vi "Main_Marvin Remake.vi"() -> ()   [LabVIEW 2017]
uses:
  PCAN_Driver/ControlCAN.llb/DevType.ctl
  PCAN_Driver/ControlCAN.llb/CAN Channel.ctl
  PCAN_Driver/ControlCAN.llb/VCI_INIT_CONFIG.ctl
  PCAN_Driver/ControlCAN.llb/InitFlag.ctl
  PCAN_Driver/ControlCAN.llb/Fliter.ctl
  PCAN_Driver/ControlCAN.llb/Mode.ctl
  <vilib>/Utility/miscctls.llb/LVRowAndColumnTypeDef.ctl
  <vilib>/Utility/config.llb/Read Key (String).vi
  <vilib>/Utility/config.llb/Write Key (String).vi
  <vilib>/Utility/cursorutil.llb/Set Cursor (Icon Pict).vi
  PCAN_Driver/ControlCAN.lvlib
  <vilib>/Utility/config.llb/NI_LVConfig.lvlib
panel:
  out "ClosePanel":bool=TRUE
  out "UUT SN Report":string
  out "Automation":bool
  out "Test Failed":bool
  out "AuxiOFFResult":bool
  out "AuxiONResult":bool
  out "SensCalResult":bool
  out "VisualInspectionResult":bool
  out "BurnResult":bool
  out "BurnSpeed":bool
  out "BurnTemp":bool
  out "BurnDC":bool
  out "TempControlResult":bool
  out "MotorTempResult":bool
  out "StopTimeResult":bool
  out "SpeedResult":bool=TRUE
  out "VenableDirectionResult":bool
  out "VenableResult":bool
  out "ComTestResult":bool=TRUE
  out "UUT SoftwareVer":string
  out "Next SN":i32
  in  "SetSN":bool
  out "Current SN":i32
  out "Cal":dbl
  out "AO[1]Meas":dbl
  out "FullSpeed2 Speed":dbl
  out "FullSpeed2 Current":dbl
  out "FullSpeed1 Current":dbl
  out "FullSpeed1 Speed":dbl
  out "MaxBurnInTempVal":dbl
  in  "Stop Burn-in":bool
  out "VISA Tester":refnum<visa-resource-name>
  out "UUT":u8
  out "CAN Status":bool
  in  "Channel 2":T1 caption="Channel" items=["Channel 1", "Channel 2"]
  out "Config_CANAT":T7 {"DevType" items=["USB-CAN"=3, "USB-CAN2"=4]; "CanIndex" items=["通道1", "通道2"]; "VCI_INIT_CONFIG"."Fliter" items=["接收所有类型"=3, "只接收标准帧"=4, "只接收扩展帧"=7]; "VCI_INIT_CONFIG"."Mode" items=["正常工作", "自测模式（环回）", "仅侦听模式"]; "VCI_INIT_CONFIG"."InitFlag" items=["使用Flash参数", "使用界面设置参数"]}
  out "Array":u64[][](array[numeric]) format="%016x"
  out "Motor Phase Current RMS":dbl
  out "Ambient Temperature":dbl
  out "Speed error":bool
  out "Commutation err":bool
  out "Under voltage/Over voltage":bool
  out "Derated drive temp":bool
  out "Motor Over temperature":bool
  out "Motor Sensor temp Fauilre":bool
  out "Drive Over temperature":bool
  out "Drive Sensor temp Failure":bool
  out "Ambient Over temp":bool
  out "Ambient Sensor temp":bool
  out "DC Voltage":dbl
  out "DC Current":dbl
  out "Power transistor Heat sink Temp.":dbl
  out "Motor Stator Temp.":dbl
  out "Motor Speed RPM":dbl
  out "ECS State":u16
  out "UUT":string="EBAY"
  in  "Logger Path":path
  in  "Report":bool
  in  "Start":bool
  in  "ATR":string[][](table)=[["Test Communication", "-", "-", "-", "-", ""], ["Set S/N", "-", "-", "-", "-", ""], ["Set Board Number", "-", "-", "-", "-", ""], [" ", "", "", "", "", ""], ["Test Communication", "-", "-", "-", "-", ""], ["Get S/N", "-", "-", "-", "", ""], ["Get Board Number", "-", "-", "-", "", ""], ["Get FW", "-", "-", "-", "", ""], ["Enable Motor", "", "", "", "", ""], ["Small position command", "", "", "", "", ""], ["Measure delta", "", "", "", "", ""], ["Velocity command", "", "", "", "", ""]]
  in  "Settings":bool
  in  "Refresh Button":bool
  out "Status":bool
  in  "VISA Marvin":refnum<visa-resource-name>="COM6"
  in  "Serial Com":bool
  in  "Help Button":bool
  out "Pannel User Message":string
  in  "Stop Button":bool
  # "Marvin"
  # "REDLER TECHNOLOGIES LTD"
  # "ver 1.2o"
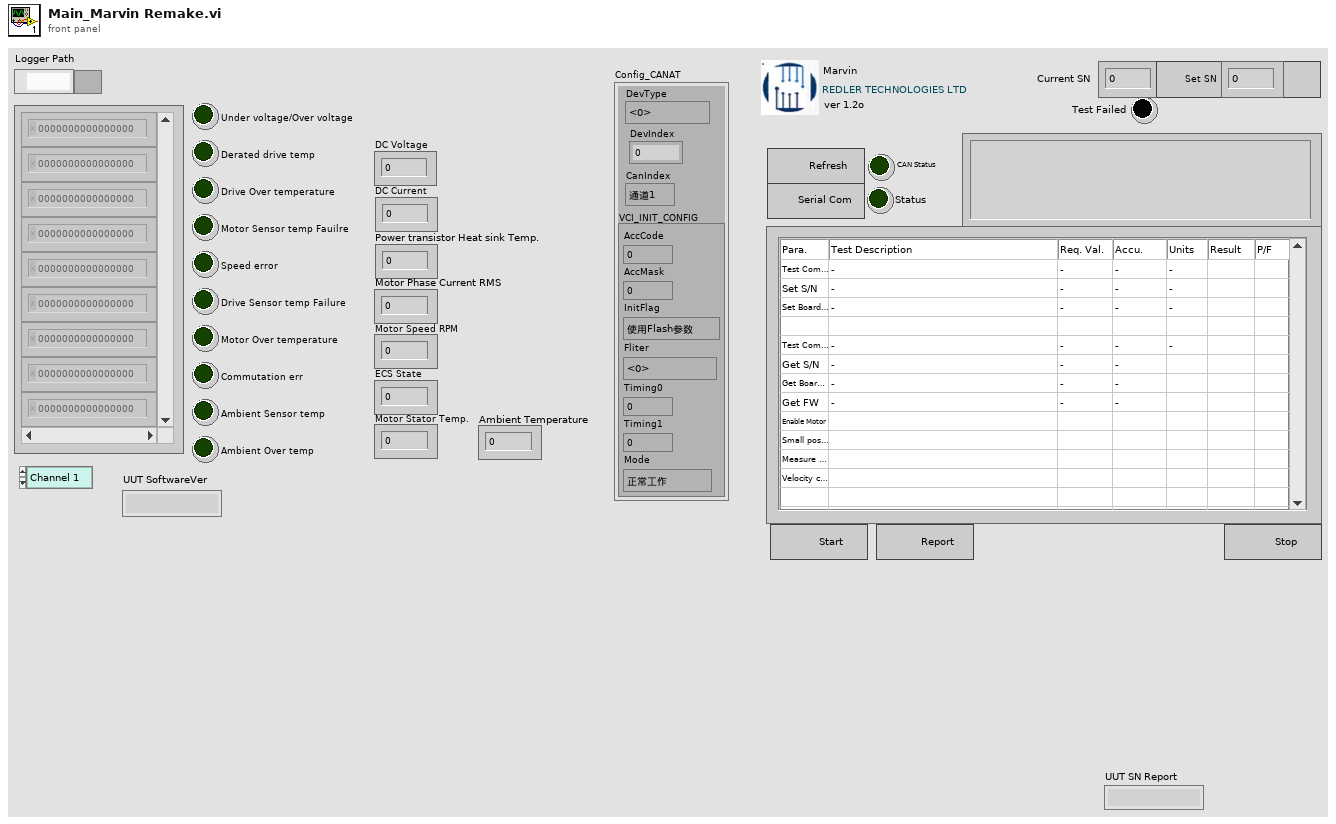
[diagram p1: front panel]
types:
  T1 = typedef "ControlCAN.lvlib/CAN Channel.ctl" = u32
  T2 = typedef "ControlCAN.lvlib/DevType.ctl" = u32
  T3 = typedef "ControlCAN.lvlib/VCI_INIT_CONFIG.ctl" = cluster{"AccCode":u32, "AccMask":u32, "InitFlag":T4, "Fliter":T5, "Timing0":u8, "Timing1":u8, "Mode":T6}
  T4 = typedef "ControlCAN.lvlib/InitFlag.ctl" = u32
  T5 = typedef "ControlCAN.lvlib/Fliter.ctl" = u8
  T6 = typedef "ControlCAN.lvlib/Mode.ctl" = u8
  T7 = cluster{"DevType":T2, "DevIndex":u32, "CanIndex":T1, "VCI_INIT_CONFIG":T3}
  T8 = cluster{"VISA":refnum<visa-resource-name>, "Array Test":enum16{"Auxiliary", "Temp Sens Cal", "Com Test", "Enable Test", "Speed Command", "Stop Time", "Temp Control", "Burn in", "Visual Inspec", "Empty"}[]}
  T9 = cluster{"ID":u32, "MSGTYPE":u8, "LEN":u8, "aDATA":u8[]}[]
  T10 = enum16{"Erase ATR Table", "Stop", "MainProgram", "Initialize"}
  T11 = enum16{"K15", "K16", "K17", "Venable", "Firmeware", "Fan", "Power", "120C", "110C", "100C", "90C", "80C", "70C", "60C", "50C", "40C", "30C", "25C", "20C", "10C", "0C"}
  T12 = enum16{"Stop", "Result", "FullSpeed2", "MD[1]=1", "FullSpeed1", "MD[1]=0"}
  T13 = enum8{"Term1", "Term2", "Current", "Fan", "TempCPU"}
  T14 = enum16{"Stop", "AO[1]=Meas.", "TA[5]", "AO[1]=0", "Start"}
  T15 = enum16{"Stop", "BurnIn", "Ambient Temp", "MotorSpeed", "DC Current Measure", "Start"}
  T16 = enum16{"Auxiliary", "Temp Sens Cal", "Com Test", "Enable Test", "Speed Command", "Stop Time", "Temp Control", "Burn in", "Visual Inspec", "Empty"}[]
  T17 = enum16{"K15", "K16", "K17", "Venable", "Firmeware", "Fan", "Power", "120C", "110C", "100C", "90C", "80C", "70C", "60C", "50C", "40C", "30C", "25C", "20C", "10C", "0C"}[]
  T18 = typedef "NI_LVConfig.lvlib/Config Data RefNum.ctl" = refnum<k1>
  T19 = enum32{"6000", "11500", "15100", "11500-2", "6000-2"}[]
  T20 = enum8{"Enabled", "Disabled", "Disabled and Grayed Out"}
  T21 = typedef "LVRowAndColumnTypeDef.ctl" = cluster{"Row":i32, "Column":i32}
  T22 = enum32{"Invalid", "Standard", "Closed", "Hidden", "Minimized", "Maximized"}
  T23 = cluster{"ID":u32, "MSGTYPE":u8, "LEN":u8, "aDATA":u8[]}
  T24 = enum16{"Auxiliary", "Temp Sens Cal", "Com Test", "Enable Test", "Speed Command", "Stop Time", "Temp Control", "Burn in", "Visual Inspec", "Empty"}
  T25 = enum16{"open", "replace", "create", "open or create", "replace or create", "replace or create with confirmation"}
  T26 = typedef "ControlCAN.lvlib/VCI_CAN_OBJ.ctl" = cluster{"ID":u32, "TimeStamp":u32, "TimeFlag":u8, "SendType":u8, "RemoteFlag":u8, "ExternFlag":u8, "DataLen":u8, "Data":u8[], "Reserved":u8[]}
  T27 = cluster{"Type":enum16{"接收", "发送"}, "Channel":T1, "Time":timestamp, "VCI_CAN_OBJ":T26}[]
  T28 = cluster{"Type":enum16{"接收", "发送"}, "Channel":T1, "Time":timestamp, "VCI_CAN_OBJ":T26}
  T29 = typedef "LVPoint32TypeDef.ctl" = cluster{"Horizontal":i32, "Vertical":i32}
  T30 = enum8{"Term1", "Term2", "Current", "Fan", "TempCPU"}[]
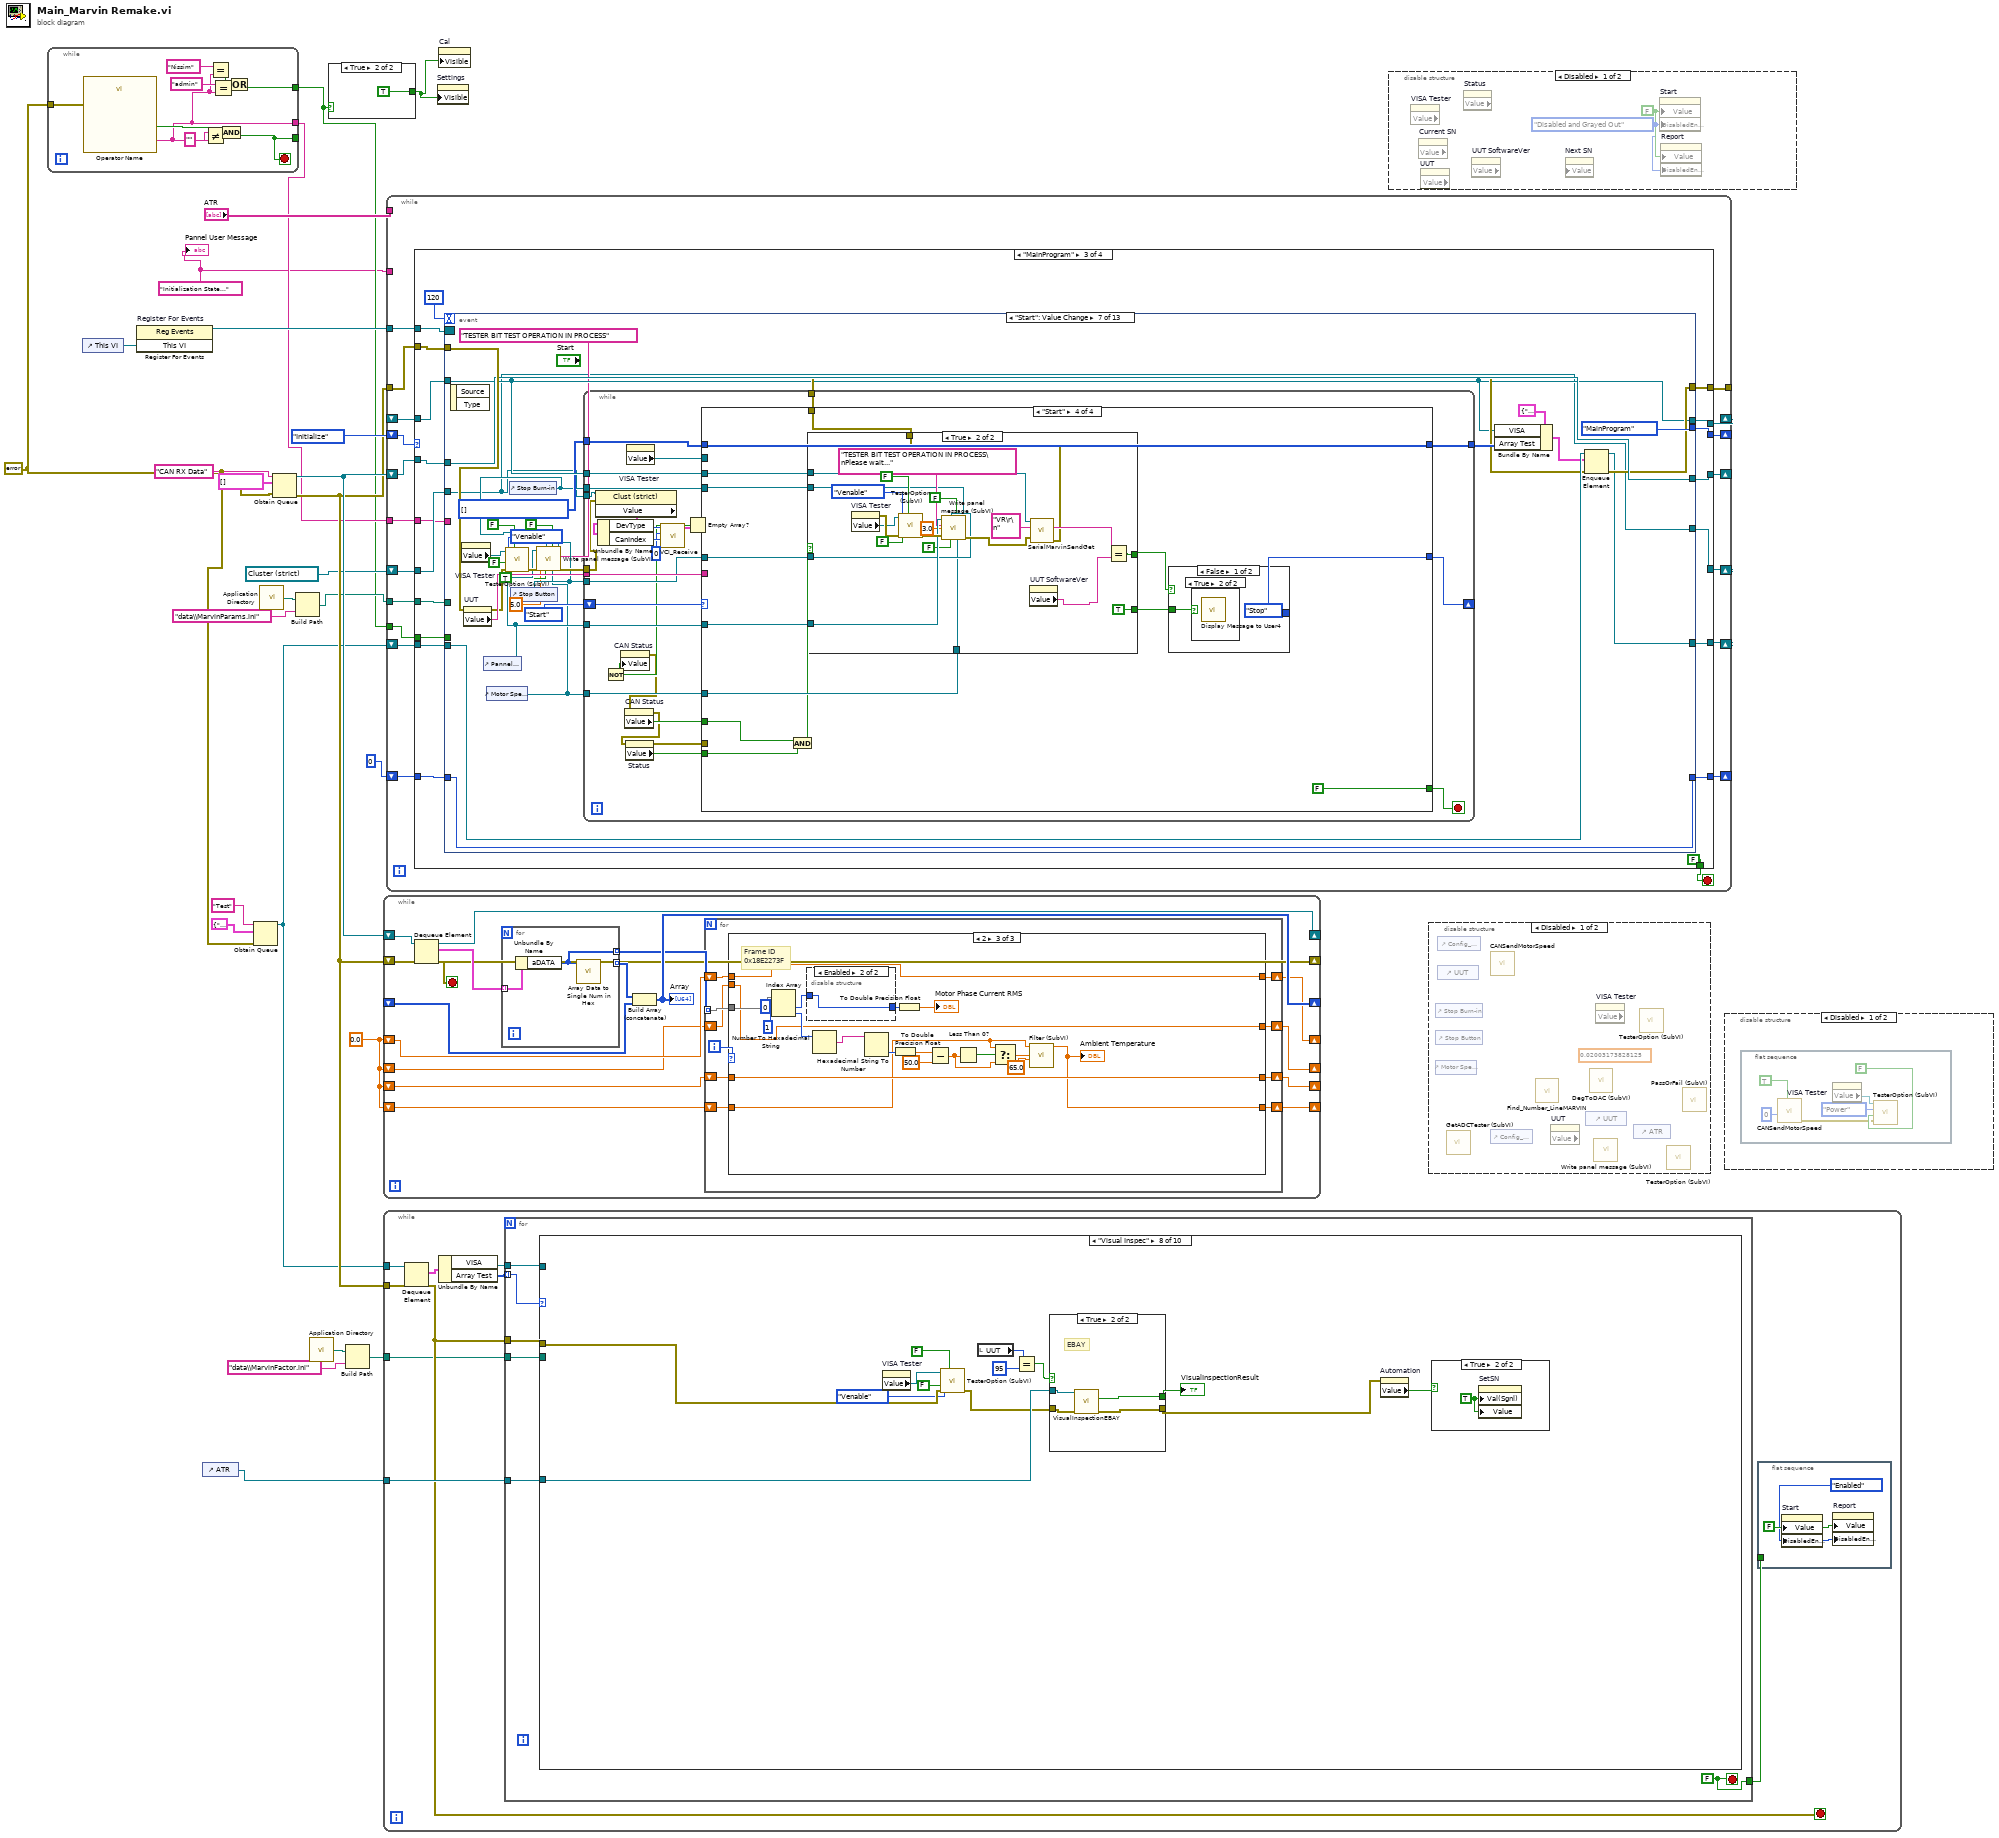
[diagram p0: block diagram]
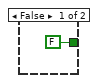
[diagram p2: hidden frame]
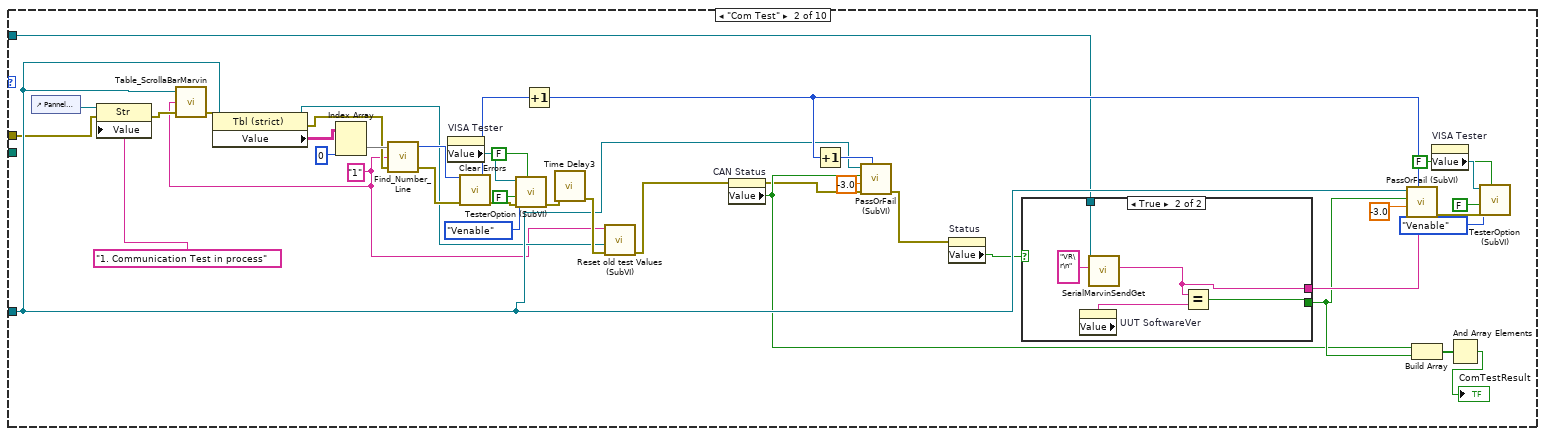
[diagram p7: hidden frame]
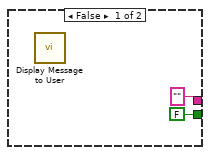
[diagram p8: hidden frame]
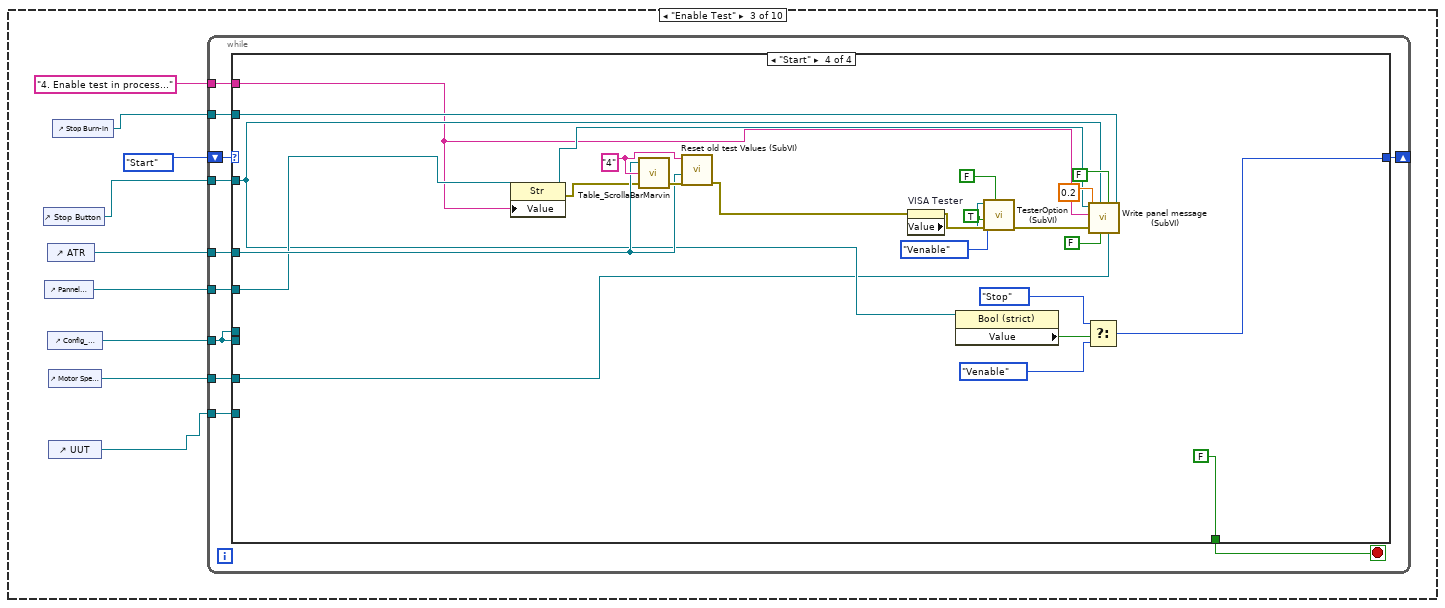
[diagram p9: hidden frame]
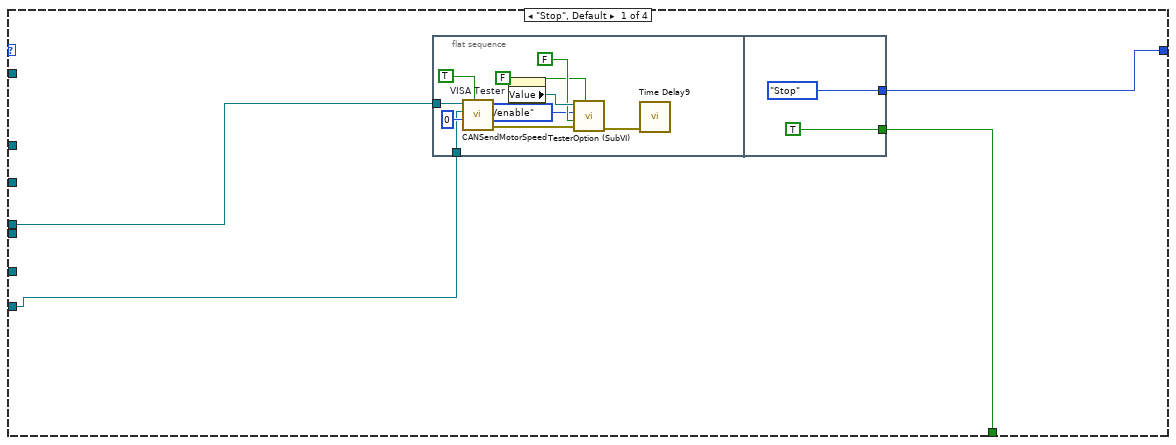
[diagram p10: hidden frame]
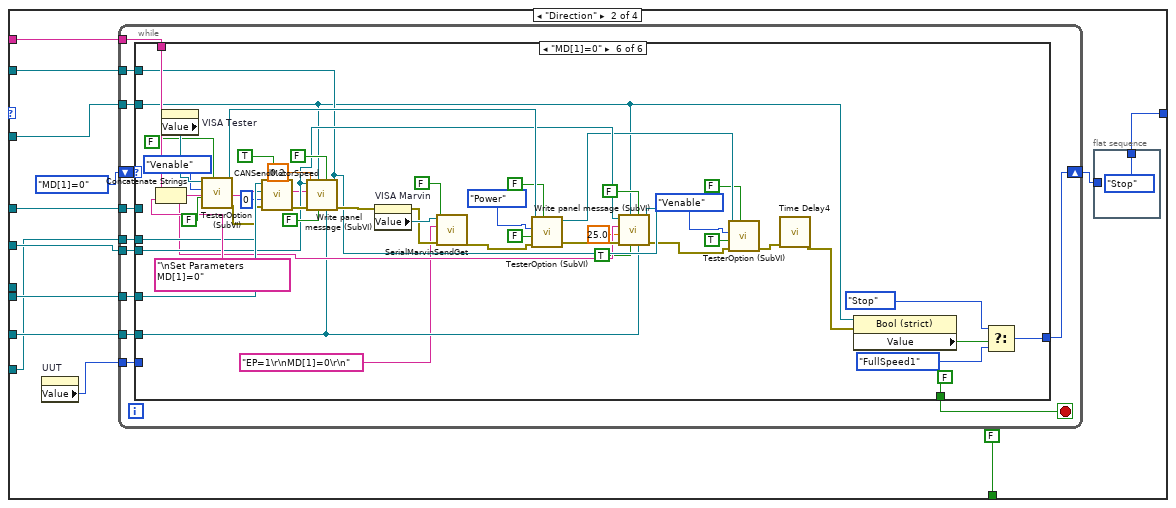
[diagram p11: hidden frame]
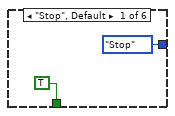
[diagram p12: hidden frame]
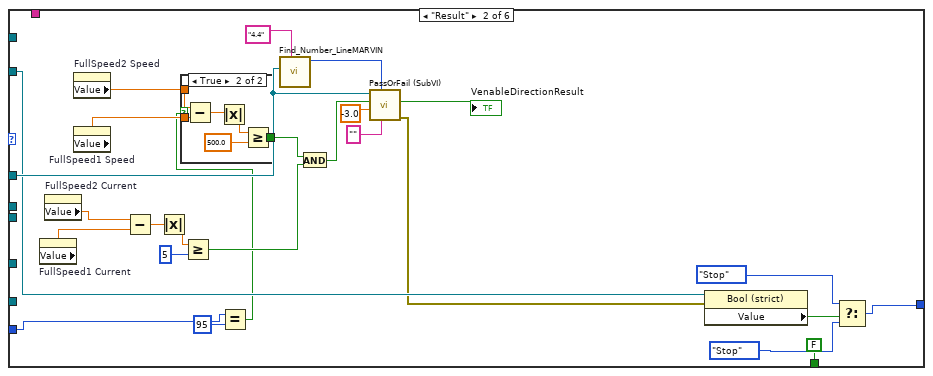
[diagram p13: hidden frame]
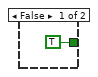
[diagram p14: hidden frame]
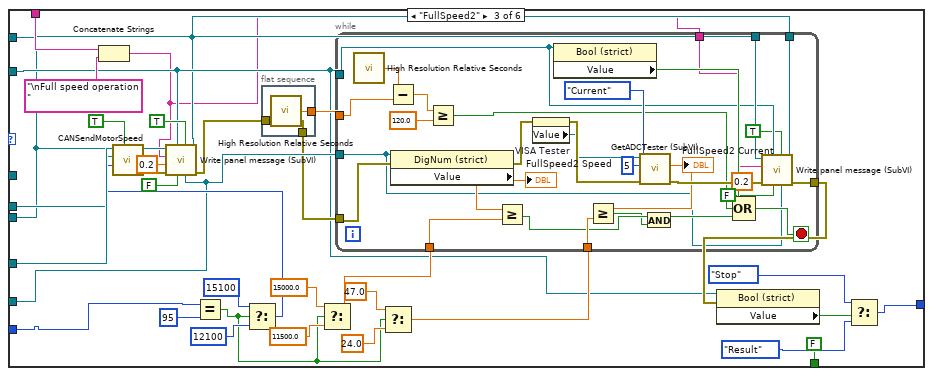
[diagram p15: hidden frame]
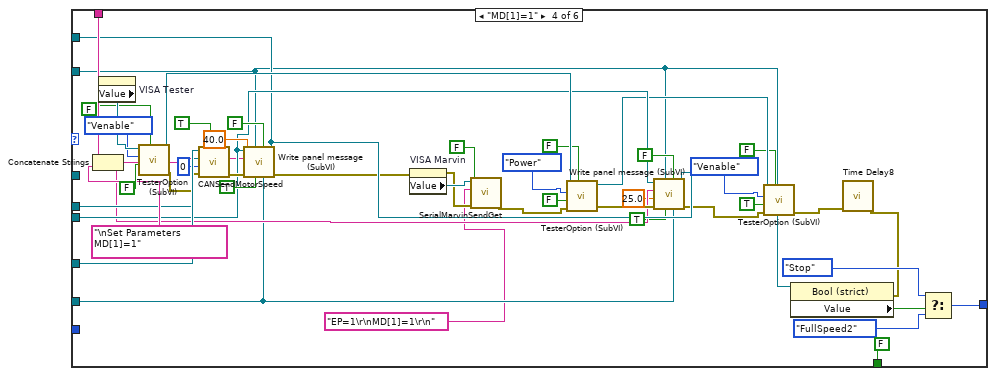
[diagram p16: hidden frame]
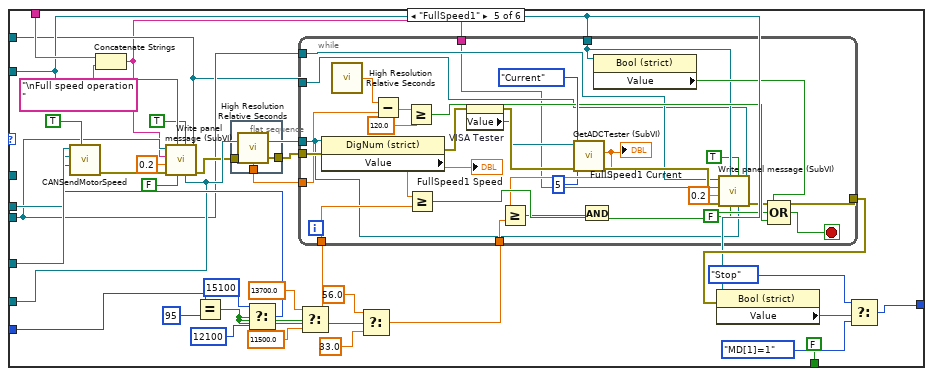
[diagram p17: hidden frame]
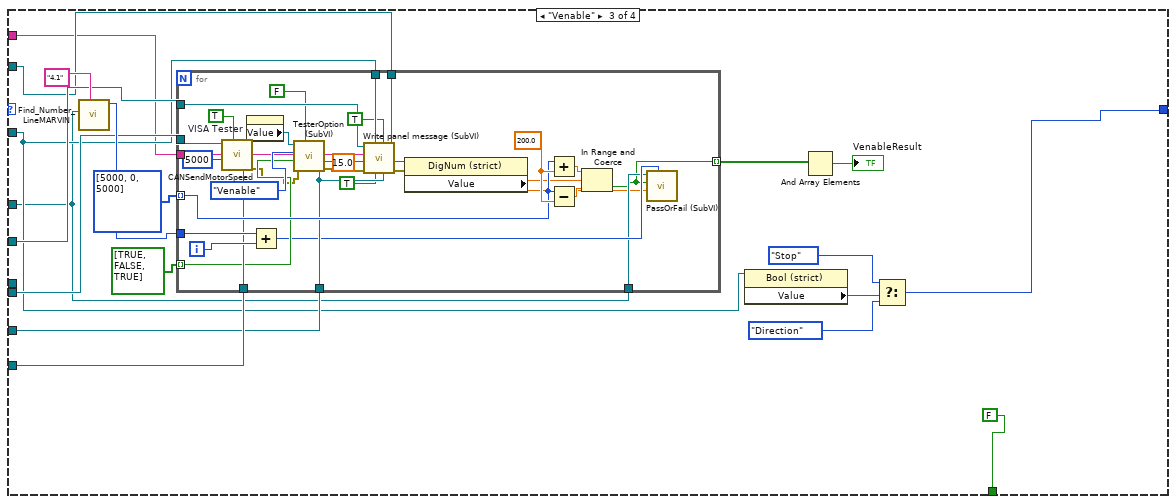
[diagram p18: hidden frame]
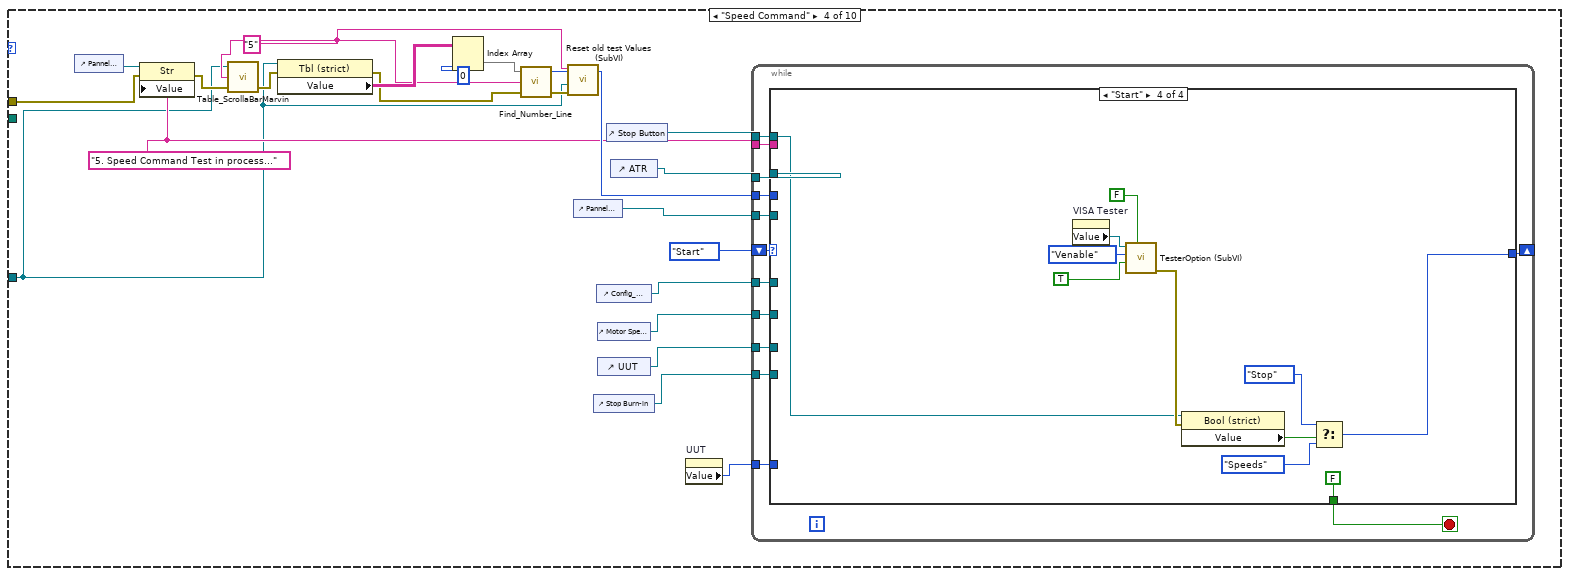
[diagram p19: hidden frame]
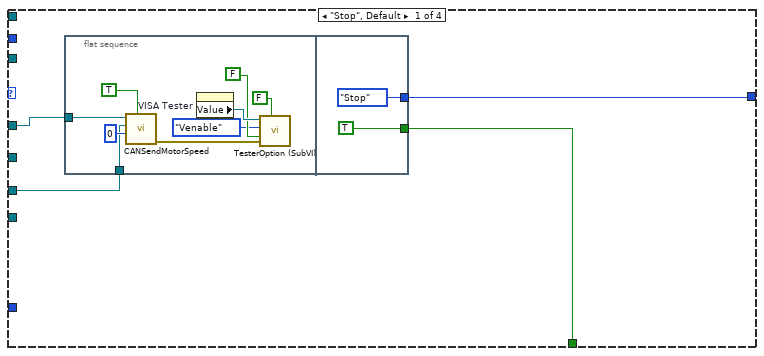
[diagram p20: hidden frame]
diagram:
  w5 = "Initialization State..."
  w16 = 0.0
  w15 = errorcluster {"status"=FALSE, "code"=0, "source"=""} ("error in (no error)")
  n1 = while {
    tunnel: [w34] -> _
    tunnel: [w30] -> w10
    tunnel: [w31] -> w6
    tunnel: w15 -> [w27]
    stop <- w34 stop-if-true
    n2 = call "Operator Name"("error in (no error)"=w27) -> ("Operator Name"=w30:string, "OK"=w35:bool)  [unwired: 16 in, 1 out]
    n3 = Not Equal?(x=w30, y="") -> (x != y?=w36:bool)
    n4 = Equal?(x="Nissim", y=w30) -> (x = y?=w28:bool)
    n5 = Equal?(x="admin", y=w30) -> (x = y?=w32:bool)
    n6 = And(x=w35, y=w36) -> (x .and. y?=w34:bool)
    n7 = Or(x=w28, y=w32) -> (x .or. y?=w31:bool)
  }
  n8 = control-ref of="This VI"() -> (w12:refnum<vi>)
  n9 = register-events "Register For Events"(w12) -> (reference out=w11:refnum<event-registration>)  [unwired: 2 in, 1 out]
  n10 = control-ref of="ATR"() -> (w4:refnum<vi>)
  n11 = Obtain Queue(name (unnamed)="Test", element data type=T8 {"VISA"="COM1", "Array Test"=[]}, error in (no error)=w15) -> (queue out=w20:refnum<queue>)  [unwired: 2 in, 2 out]
  n12 = call <vilib>:"Application Directory.vi"() -> ("Application Directory"=w14:path)
  n13 = Obtain Queue(name (unnamed)="CAN RX Data", element data type=T9 [], error in (no error)=w15) -> (queue out=w23:refnum<queue>, error out=w21:errorcluster)  [unwired: 2 in, 1 out]
  n14 = Build Path(base path=w14, name or relative path="data\\MarvinParams.ini") -> (appended path=w8:path)
  n15 = call <vilib>:"Application Directory.vi"() -> ("Application Directory"=w2:path)
  n16 = case shown="True" w6 {
    tunnel: [FALSE TRUE] -> w7
    frame False {
    }
    frame True {
    }
  }
  n17 = Build Path(base path=w2, name or relative path="data\\MarvinFactor.ini") -> (appended path=w1:path)
  n18 = while {
    shift-right: [w54] -> _
    shift-left: w23 -> [w56]
    shift-right: [w52] -> _
    shift-left: _ -> [w53]
    shift-right: [w48] -> _
    shift-left: w21 -> [w48]
    shift-right: [w46] -> _
    shift-left: w16 -> [w47]
    shift-right: [w45] -> _
    shift-left: w16 -> [w44]
    shift-right: [w43] -> _
    shift-left: w16 -> [w42]
    shift-right: [w41] -> _
    shift-left: w16 -> [w40]
    stop <- w55 stop-if-true
    n19 = Dequeue Element(queue=w56, error in (no error)=w48) -> (queue out=w54:refnum<queue>, element=w49:T9, error out=w55:errorcluster)  [unwired: 1 in, 1 out]
    n20 = for {
      tunnel: [w185] -> w51 mode=indexing
      tunnel: w49 -> [w184] mode=indexing
      tunnel: [w183] -> w50 mode=indexing
      n21 = Unbundle By Name(w184) -> ("aDATA"=w183:u8[])
      n22 = call "Array Data to Single Num in Hex.vi"("aDATA"=w183) -> ("Numeric"=w185:u64)  [unwired: 10 in]
    }
    n23 = Build Array (concatenate)(w51, w53) -> (w52:u64[][])
    "Array" <- w52
    n24 = for {
      tunnel: w50 -> [w66] mode=indexing
      shift-right: [w63] -> w46
      shift-left: w47 -> [w64]
      shift-right: [w62] -> w45
      shift-left: w44 -> [w61]
      shift-right: [w60] -> w43
      shift-left: w42 -> [w59]
      shift-right: [w58] -> w41
      shift-left: w40 -> [w57]
      i -> [w65]
      n25 = case shown="2" w65 {
        tunnel: w66 -> [w106 w139 w178]
        tunnel: w64 -> [w80 w128 w167]
        tunnel: [w78 w128 w167] -> w63
        tunnel: [w75 w127 w166] -> w62
        tunnel: w61 -> [w74 w127 w166]
        tunnel: [w69 w126 w165] -> w60
        tunnel: w59 -> [w68 w126 w165]
        tunnel: [w67 w125 w160] -> w58
        tunnel: w57 -> [w67 w125 w159]
        frame 0, Default {
          # "Frame ID\n0x18E1273F"
          n26 = Index Array(array=w106, index #1=0 ("index"), index #2=1 ("index"), index #3=2 ("index"), index #4=3 ("index"), index #5=4 ("index"), index #6=5 ("index"), index #7=6 ("index"), index #8=7 ("index")) -> (element #1=w90:u8, element #2=w92:u8, element #3=w93:u8, element #4=w97:u8, element #5=w100:u8, element #6=w104:u8, element #7=w105:u8, element #8=w103:u8)
          n27 = Number To Hexadecimal String(2:w103) -> (0:w117:string)  [unwired: 1 in]
          n28 = Join Numbers(hi=w105, lo=w104) -> ((hi.lo)=w124:u16)
          n29 = Join Numbers(hi=w93, lo=w92) -> ((hi.lo)=w94:u16)
          n30 = Number To Hexadecimal String(2:w100) -> (0:w101:string)  [unwired: 1 in]
          n31 = Number To Hexadecimal String(2:w124) -> (0:w123:string)  [unwired: 1 in]
          n32 = Number To Hexadecimal String(2:w90) -> (0:w91:string)  [unwired: 1 in]
          n33 = Number To Hexadecimal String(2:w94) -> (0:w95:string)  [unwired: 1 in]
          n34 = Number To Hexadecimal String(2:w97) -> (0:w98:string)  [unwired: 1 in]
          n35 = Hexadecimal String To Number(string=w117) -> (number=w116:u32)  [unwired: 2 in, 1 out]
          n36 = To Double Precision Float(number=w116) -> (double precision float=→"DC Current":dbl)
          n37 = Hexadecimal String To Number(string=w101) -> (number=w102:u32)  [unwired: 2 in, 1 out]
          n38 = Hexadecimal String To Number(string=w123) -> (number=w122:u32)  [unwired: 2 in, 1 out]
          n39 = Hexadecimal String To Number(string=w91) -> (number=w88:u32)  [unwired: 2 in, 1 out]
          n40 = Hexadecimal String To Number(string=w95) -> (number=w96:u32)  [unwired: 2 in, 1 out]
          n41 = Hexadecimal String To Number(string=w98) -> (number=w99:u32)  [unwired: 2 in, 1 out]
          n42 = To Double Precision Float(number=u32 10 ("y")) -> (double precision float=w120:dbl)
          n43 = To Double Precision Float(number=w122) -> (double precision float=w119:dbl)
          n44 = To Double Precision Float(number=w102) -> (double precision float=w85:dbl)
          n45 = To Double Precision Float(number=w96) -> (double precision float=w81:dbl)
          n46 = To Double Precision Float(number=w99) -> (double precision float=w87:dbl)
          n47 = Divide(x=w119, y=w120) -> (x/y=→"DC Voltage":dbl)
          n48 = To Unsigned Word Integer(number=w88) -> (unsigned 16bit integer=→"ECS State":u16)
          n49 = Subtract(x=w85, y=50.0 ("x")) -> (x-y=w73:dbl)
          n50 = Subtract(x=w87, y=50.0 ("x")) -> (x-y=w76:dbl)
          n51 = call "Filter (SubVI).vi"("Delta"=5000.0, "NewVal"=w81, "OldVal"=w80) -> ("Val"=w78:dbl)  [unwired: 8 in]
          "Motor Speed RPM" <- w78
          n52 = Less Than 0?(x=w76) -> (x < 0?=w83:bool)
          n53 = Less Than 0?(x=w73) -> (x < 0?=w82:bool)
          n54 = Select(t=w74, s=w83, f=w76) -> (s? t:f=w77:dbl)
          n55 = Select(t=w68, s=w82, f=w73) -> (s? t:f=w72:dbl)
          n56 = call "Filter (SubVI).vi"("Delta"=130.0, "NewVal"=w77, "OldVal"=w74) -> ("Val"=w75:dbl)  [unwired: 8 in]
          "Motor Stator Temp." <- w75
          n57 = call "Filter (SubVI).vi"("Delta"=100.0, "NewVal"=w72, "OldVal"=w68) -> ("Val"=w69:dbl)  [unwired: 8 in]
          "Power transistor Heat sink Temp." <- w69
        }
        frame 1 {
          # "Framde ID\n0x18E3273F"
          n58 = control-ref of="UUT"() -> (w129:refnum<vi>)
          n59 = property on="Property Node" class="DigNum (strict)"(reference=w129) -> ("Value"=w130:u8)  [unwired: 1 in, 2 out]
          n60 = Index Array(array=w139, index #1=0 ("index"), index #2=1 ("index")) -> (element #1=w137:u8, element #2=w132:u8)
          n61 = Number To Boolean Array(number=w137) -> (Boolean array=w136:bool[])
          n62 = Number To Boolean Array(number=w132) -> (Boolean array=w134:bool[])
          n63 = Boolean To (0,1)(Boolean=w134) -> (0, 1=w131:i16[])
          n64 = Boolean To (0,1)(Boolean=w136) -> (0, 1=w135:i16[])
          n65 = case shown="95" w130 {
            tunnel: w131 -> [_ w140]
            frame 0, Default {
            }
            frame 95 {
              n66 = for {
                tunnel: w140 -> [w145] mode=indexing
                i -> [w141]
                stop <- w143 stop-if-true
                n67 = Not Equal To 0?(x=w145) -> (x != 0?=w144:bool)
                n68 = case shown="0, Default" w141 {
                  tunnel: w144 -> [w146 w147]
                  frame 0, Default {
                    "Ambient Sensor temp" <- w146
                  }
                  frame 1 {
                    "Ambient Over temp" <- w147
                  }
                }
                n69 = Equal?(x=w141, y=1.0) -> (x = y?=w143:bool)
              }
            }
          }
          n70 = for {
            tunnel: w135 -> [w149] mode=indexing
            i -> [w150]
            n71 = Not Equal To 0?(x=w149) -> (x != 0?=w148:bool)
            n72 = case shown="1" w150 {
              tunnel: w148 -> [w151 w152 w153 w154 w155 w156 w157 w158]
              frame 0, Default {
                "Drive Sensor temp Failure" <- w151
              }
              frame 1 {
                "Drive Over temperature" <- w152
              }
              frame 2 {
                "Motor Sensor temp Fauilre" <- w153
              }
              frame 3 {
                "Motor Over temperature" <- w154
              }
              frame 4 {
                "Derated drive temp" <- w155
              }
              frame 5 {
                "Under voltage/Over voltage" <- w156
              }
              frame 6 {
                "Commutation err" <- w157
              }
              frame 7 {
                "Speed error" <- w158
              }
            }
          }
        }
        frame 2 {
          # "Frame ID\n0x18E2273F"
          n73 = Index Array(array=w178, index #1=0 ("index"), index #2=1 ("index")) -> (element #1=w175:u8, element #2=w172:u8)
          n74 = disable-structure shown="Enabled" {
            disable-tunnel: [w181 w182] -> w176
            disable-tunnel: w175 -> [w180 w182]
            frame Disabled {
              n75 = Number To Hexadecimal String(2:w180) -> (0:w179:string)  [unwired: 1 in]
              n76 = Hexadecimal String To Number(string=w179) -> (number=w181:u32)  [unwired: 2 in, 1 out]
            }
            frame Enabled {
            }
          }
          n77 = Number To Hexadecimal String(2:w172) -> (0:w170:string)  [unwired: 1 in]
          n78 = Hexadecimal String To Number(string=w170) -> (number=w171:u32)  [unwired: 2 in, 1 out]
          n79 = To Double Precision Float(number=w171) -> (double precision float=w169:dbl)
          n80 = To Double Precision Float(number=w176) -> (double precision float=→"Motor Phase Current RMS":dbl)
          n81 = Subtract(x=w169, y=50.0) -> (x-y=w163:dbl)
          n82 = Less Than 0?(x=w163) -> (x < 0?=w164:bool)
          n83 = Select(t=w159, s=w164, f=w163) -> (s? t:f=w162:dbl)
          n84 = call "Filter (SubVI).vi"("Delta"=65.0, "NewVal"=w162, "OldVal"=w159) -> ("Val"=w160:dbl)  [unwired: 8 in]
          "Ambient Temperature" <- w160
        }
      }
    }
  }
  n85 = while {
    tunnel: w4 -> [w194]
    tunnel: w21 -> [w192]
    tunnel: w20 -> [w193]
    tunnel: w1 -> [w186]
    stop <- w188 stop-if-true
    n86 = Dequeue Element(queue=w193, error in (no error)=w192) -> (element=w191:T8, error out=w188:errorcluster)  [unwired: 1 in, 2 out]
    n87 = Unbundle By Name(w191) -> ("VISA"=w190:refnum<visa-resource-name>, "Array Test"=w189:T16)
    n88 = for {
      tunnel: w189 -> [w199] mode=indexing
      tunnel: w190 -> [w202]
      tunnel: w194 -> [w201]
      tunnel: w188 -> [w200]
      tunnel: [w198] -> w187
      tunnel: w186 -> [w197]
      stop <- w198 stop-if-true
      w198 = FALSE
      n89 = case shown="\"Visual Inspec\"" w199 {
        tunnel: w202 -> [_ w226 _ _ w810 _ _ _ w1384 _]
        tunnel: w201 -> [_ w233 _ w645 w806 w983 _ w1370 w1391 w1603]
        tunnel: w200 -> [_ w230 _ w660 w816 w965 _ w1369 w1389 w1602]
        tunnel: w197 -> [_ _ _ _ _ w967 _ _ _ _]
        frame "Empty", Default {
        }
        frame "Com Test" {
          w209 = "1" ("Test Paragraph")
          n90 = control-ref of="Pannel User Message"() -> (w231:refnum<vi>)
          n91 = property class="Str"(reference=w231, error in=w230, "Value"="1. Communication Test in process") -> (error out=w229:errorcluster)  [unwired: 1 out]
          n92 = call "Table_ScrollaBarMarvin.vi"("error in"=w229, "Line to focus"=w209, "reference in"=w233) -> ("error out"=w232:errorcluster)  [unwired: 2 out]
          n93 = property class="Tbl (strict)"(reference=w233, error in=w232) -> (reference out=w210:refnum<vi>, error out=w240:errorcluster, "Value"=w241:string[][])
          n94 = Index Array(array=w241, index (col)=0 ("disabled index (col)")) -> (element=w242:string[])  [unwired: 1 in]
          n95 = call "Find_Number_Line.vi"("error in"=w240, "Test Paragraph"=w209, "Row Headers[]"=w242) -> ("error out"=w238:errorcluster, "Line number"=w237:i32)  [unwired: 1 out]
          n96 = property on="VISA Tester" class="VISAName"() -> ("Value"=w220:refnum<visa-resource-name>)  [unwired: 2 in, 2 out]
          n97 = call <vilib>:"Clear Errors.vi"("error in (no error)"=w238) -> ("error out"=w222:errorcluster)  [unwired: 5 in, 1 out]
          n98 = call "TesterOption (SubVI).vi"("2 Options"=FALSE, "error in (no error)"=w222, "On/Off"=FALSE, "Tester Option"=T11."Venable", "VISA Refnum in"=w220) -> ("error out"=w221:errorcluster)  [unwired: 5 in, 1 out]
          n99 = Increment(x=w237) -> (x+1=w236:i32)
          n100 = call "Time Delay3"("error in (no error)"=w221) -> ("error out"=w234:errorcluster)  [unwired: 10 in]
          n101 = call "Reset old test Values (SubVI).vi"("error in"=w234, "Atr in"=w210, "Test Paragraph"=w209) -> ("error out"=w204:errorcluster)  [unwired: 8 in]
          n102 = property on="CAN Status" class="Bool (strict)"(error in=w204) -> (error out=w203:errorcluster, "Value"=w205:bool)  [unwired: 1 in, 1 out]
          n103 = Increment(x=w236) -> (x+1=w235:i32)
          n104 = call "PassOrFail (SubVI).vi"("index (row)"=w235, "error in (no error)"=w203, "Data in"=-3.0, "Pass?Fail"=w205, "Table in"=w233) -> ("error out"=w225:errorcluster)  [unwired: 6 in]
          n105 = property on="Status" class="Bool (strict)"(error in=w225) -> ("Value"=w227:bool)  [unwired: 1 in, 2 out]
          n106 = case shown="True" w227 {
            tunnel: w226 -> [_ w249]
            tunnel: [FALSE w246] -> w207
            tunnel: ["" ("read buffer") w245] -> w224
            frame False {
              n107 = call "Display Message to User"() -> ()  [unwired: 10 in, 2 out]
            }
            frame True {
              n108 = property on="UUT SoftwareVer" class="Str"() -> ("Value"=w247:string)  [unwired: 2 in, 2 out]
              n109 = call "SerialMarvinSendGet.vi"("write buffer"="VR\r\n", "VISA resource name"=w249) -> ("read buffer"=w245:string)  [unwired: 8 in, 1 out]
              n110 = Equal?(x=w245, y=w247) -> (x = y?=w246:bool)
            }
          }
          n111 = call "PassOrFail (SubVI).vi"("String Res"=w224, "index (row)"=w236, "Data in"=-3.0, "Pass?Fail"=w207, "Table in"=w233) -> ("error out"=w216:errorcluster)  [unwired: 6 in]
          n112 = Build Array(w205, w207) -> (w208:bool[])
          n113 = property on="VISA Tester" class="VISAName"() -> ("Value"=w215:refnum<visa-resource-name>)  [unwired: 2 in, 2 out]
          n114 = And Array Elements(Boolean array=w208) -> (logical AND=→"ComTestResult":bool)
          n115 = call "TesterOption (SubVI).vi"("2 Options"=FALSE, "error in (no error)"=w216, "On/Off"=FALSE, "Tester Option"=T11."Venable", "VISA Refnum in"=w215) -> ()  [unwired: 5 in, 2 out]
        }
        frame "Enable Test" {
          n116 = control-ref of="Stop Button"() -> (w252:refnum<vi>)
          n117 = control-ref of="Pannel User Message"() -> (w254:refnum<vi>)
          n118 = control-ref of="ATR"() -> (w253:refnum<vi>)
          n119 = control-ref of="Config_CANAT"() -> (w255:refnum<vi>)
          n120 = control-ref of="Motor Speed RPM"() -> (w256:refnum<vi>)
          n121 = control-ref of="UUT"() -> (w257:refnum<vi>)
          n122 = control-ref of="Stop Burn-in"() -> (w258:refnum<vi>)
          n123 = while {
            shift-right: [w263] -> _
            shift-left: enum16{"Stop", "Direction", "Venable", "Start"}."Start" -> [w269]
            tunnel: w252 -> [w268]
            tunnel: w253 -> [w267]
            tunnel: w254 -> [w266]
            tunnel: w255 -> [w259]
            tunnel: w256 -> [w265]
            tunnel: w257 -> [w260]
            tunnel: w258 -> [w262]
            tunnel: "4. Enable test in process..." ("Strin") -> [w261]
            stop <- w264 stop-if-true
            n124 = case shown="\"Start\"" w269 {
              tunnel: w268 -> [_ w296 w577 w624]
              tunnel: w267 -> [_ w291 w575 w631]
              tunnel: w266 -> [_ w294 w579 w630]
              tunnel: w259 -> [_ w297 w582 _]
              tunnel: w265 -> [_ w293 w580 w622]
              tunnel: w260 -> [w270 w287 w581 _]
              tunnel: [w273 FALSE FALSE FALSE] -> w264
              tunnel: [w271 w290 w576 w628] -> w263
              tunnel: w262 -> [_ w295 w578 w623]
              tunnel: w261 -> [_ w292 w574 w621]
              tunnel: w259 -> [w272 _ _ _]
              frame "Stop", Default {
                n125 = flat-sequence {
                  tunnel: w270 -> [w279]
                  tunnel: w272 -> [w278]
                  tunnel: [TRUE] -> w273
                  tunnel: [enum16{"Stop", "Direction", "Venable", "Start"}."Stop"] -> w271
                  frame #0 {
                    n126 = call "CANSendMotorSpeed.vi"("Remote"=TRUE, "Motor Speed RPM"=u16 0, "UUT"=w279, "CAN Cluster in"=w278) -> ("error out"=w282:errorcluster)  [unwired: 7 in]
                    n127 = property on="VISA Tester" class="VISAName"() -> ("Value"=w283:refnum<visa-resource-name>)  [unwired: 2 in, 2 out]
                    n128 = call "TesterOption (SubVI).vi"("2 Options"=FALSE, "error in (no error)"=w282, "On/Off"=FALSE, "Tester Option"=T11."Venable", "VISA Refnum in"=w283) -> ("error out"=w274:errorcluster)  [unwired: 5 in, 1 out]
                    n129 = call "Time Delay9"("error in (no error)"=w274) -> ()  [unwired: 10 in, 1 out]
                  }
                  frame #1 {
                  }
                }
              }
              frame "Direction" {
                n130 = property on="UUT" class="DigNum (strict)"() -> ("Value"=w286:u8)  [unwired: 2 in, 2 out]
                n131 = while {
                  shift-right: [w310] -> w289
                  shift-left: T12."MD[1]=0" -> [w311]
                  tunnel: w297 -> [w308]
                  tunnel: w287 -> [w307]
                  tunnel: w296 -> [w306]
                  tunnel: w295 -> [w305]
                  tunnel: w294 -> [w304]
                  tunnel: w293 -> [w303]
                  tunnel: w292 -> [w302]
                  tunnel: w291 -> [w301]
                  tunnel: w286 -> [w300]
                  stop <- w309 stop-if-true
                  n132 = case shown="\"MD[1]=0\"" w311 {
                    tunnel: [T12."Stop" w335 w377 w457 w490 w570] -> w310
                    tunnel: [TRUE FALSE FALSE FALSE FALSE FALSE] -> w309
                    tunnel: w308 -> [_ _ w375 w451 w488 w564]
                    tunnel: w307 -> [_ _ w371 w430 w484 w542]
                    tunnel: w306 -> [_ w322 w350 w421 w466 w532]
                    tunnel: w305 -> [_ _ w348 w431 w464 w543]
                    tunnel: w304 -> [_ _ w349 w432 w465 w544]
                    tunnel: w303 -> [_ _ w366 w419 w480 w538]
                    tunnel: w302 -> [_ _ w361 w440 w478 w552]
                    tunnel: w301 -> [_ w326 _ _ _ _]
                    tunnel: w300 -> [_ w314 w346 _ w459 _]
                    frame "Stop", Default {
                    }
                    frame "Result" {
                      n133 = property on="FullSpeed1 Current" class="DigNum (strict)"() -> ("Value"=w330:dbl)  [unwired: 2 in, 2 out]
                      n134 = property on="FullSpeed2 Current" class="DigNum (strict)"() -> ("Value"=w331:dbl)  [unwired: 2 in, 2 out]
                      n135 = property on="FullSpeed2 Speed" class="DigNum (strict)"() -> ("Value"=w333:dbl)  [unwired: 2 in, 2 out]
                      n136 = property on="FullSpeed1 Speed" class="DigNum (strict)"() -> ("Value"=w332:dbl)  [unwired: 2 in, 2 out]
                      n137 = Subtract(x=w331, y=w330) -> (x-y=w329:dbl)
                      n138 = Absolute Value(x=w329) -> (abs(x)=w318:dbl)
                      n139 = Greater Or Equal?(x=w318, y=u32 5) -> (x >= y?=w324:bool)
                      n140 = Equal?(x=w314, y=u8 95) -> (x = y?=w316:bool)
                      n141 = case shown="True" w316 {
                        tunnel: w333 -> [_ w344]
                        tunnel: w332 -> [_ w343]
                        tunnel: [TRUE w340] -> w325
                        frame False {
                        }
                        frame True {
                          n142 = Subtract(x=w344, y=w343) -> (x-y=w345:dbl)
                          n143 = Absolute Value(x=w345) -> (abs(x)=w342:dbl)
                          n144 = Greater Or Equal?(x=w342, y=500.0) -> (x >= y?=w340:bool)
                        }
                      }
                      n145 = call "Find_Number_LineMARVIN.vi"("Test Paragraph"="4.4", "TableIn"=w326) -> ("Line number"=w323:i32)  [unwired: 3 in, 3 out]
                      n146 = And(x=w325, y=w324) -> (x .and. y?=w315:bool)
                      "VenableDirectionResult" <- w315
                      n147 = call "PassOrFail (SubVI).vi"("String Res"="", "index (row)"=w323, "Data in"=-3.0, "Pass?Fail"=w315, "Table in"=w326) -> ("error out"=w321:errorcluster)  [unwired: 6 in]
                      n148 = property class="Bool (strict)"(reference=w322, error in=w321) -> ("Value"=w338:bool)  [unwired: 2 out]
                      n149 = Select(t=T12."Stop", s=w338, f=T12."Stop") -> (s? t:f=w335:T12)
                    }
                    frame "FullSpeed2" {
                      n150 = Concatenate Strings(w361, "\nFull speed operation " ("string")) -> (w347:string)
                      n151 = Equal?(x=w346, y=u8 95) -> (x = y?=w356:bool)
                      n152 = Select(t=u16 15100, s=w356, f=u16 12100 ("y")) -> (s? t:f=w370:u16)
                      n153 = call "CANSendMotorSpeed.vi"("Remote"=TRUE, "Motor Speed RPM"=w370, "UUT"=w371, "CAN Cluster in"=w375) -> ("error out"=w368:errorcluster)  [unwired: 7 in]
                      n154 = call "Write panel message (SubVI).vi"("Stop BurnIn"=w348, 4:"rpm"=w366, 5:"rpm"=TRUE ("rpm"), "PrintTime"=FALSE, "Stop"=w350, "error in (no error)"=w368, "Time to wait"=0.2, "Strin"=w347, "String in"=w349) -> ("error out"=w353:errorcluster)  [unwired: 2 in]
                      n155 = flat-sequence {
                        tunnel: w353 -> [w382]
                        tunnel: [w382] -> w352
                        tunnel: [w381] -> w351
                        frame #0 {
                          n156 = call <vilib>:"High Resolution Relative Seconds.vi"() -> ("relative seconds"=w381:dbl)
                        }
                      }
                      n157 = Select(t=15000.0, s=w356, f=11500.0) -> (s? t:f=w355:dbl)
                      n158 = Select(t=47.0, s=w356, f=24.0) -> (s? t:f=w354:dbl)
                      n159 = while {
                        tunnel: w366 -> [w384]
                        tunnel: w352 -> [w412]
                        tunnel: [w392] -> w363
                        tunnel: w355 -> [w405]
                        tunnel: w354 -> [w404]
                        tunnel: w351 -> [w400]
                        tunnel: w350 -> [w390]
                        tunnel: w349 -> [w391]
                        tunnel: w348 -> [w388]
                        tunnel: w347 -> [w387]
                        stop <- w402 stop-if-true
                        n160 = call <vilib>:"High Resolution Relative Seconds.vi"() -> ("relative seconds"=w401:dbl)
                        n161 = Subtract(x=w401, y=w400) -> (x-y=w399:dbl)
                        n162 = property class="DigNum (strict)"(reference=w384, error in=w412) -> (error out=w411:errorcluster, "Value"=w406:dbl)  [unwired: 1 out]
                        "FullSpeed2 Speed" <- w406
                        n163 = Greater Or Equal?(x=w399, y=120.0) -> (x >= y?=w397:bool)
                        n164 = Greater Or Equal?(x=w406, y=w405) -> (x >= y?=w396:bool)
                        n165 = property on="VISA Tester" class="VISAName"(error in=w411) -> (error out=w410:errorcluster, "Value"=w409:refnum<visa-resource-name>)  [unwired: 1 in, 1 out]
                        n166 = property class="Bool (strict)"(reference=w390) -> ("Value"=w395:bool)  [unwired: 1 in, 2 out]
                        n167 = call "GetADCTester (SubVI).vi"("error in (no error)"=w410, "GetADCTester"=T13."Current", "TimeToGet"=5, "VISA Refnum in"=w409) -> ("error out"=w407:errorcluster, "ADCValOutput Single"=w403:dbl)  [unwired: 5 in, 1 out]
                        "FullSpeed2 Current" <- w403
                        n168 = Greater Or Equal?(x=w403, y=w404) -> (x >= y?=w393:bool)
                        n169 = And(x=w396, y=w393) -> (x .and. y?=w394:bool)
                        n170 = Compound Arithmetic op=OR(w395, w397, w394) -> (w402:bool)
                        n171 = call "Write panel message (SubVI).vi"("Stop BurnIn"=w388, 4:"rpm"=w384, 5:"rpm"=TRUE ("rpm"), "PrintTime"=FALSE, "Stop"=w390, "error in (no error)"=w407, "Time to wait"=0.2, "Strin"=w387, "String in"=w391) -> ("error out"=w392:errorcluster)  [unwired: 2 in]
                      }
                      n172 = property class="Bool (strict)"(reference=w350, error in=w363) -> ("Value"=w380:bool)  [unwired: 2 out]
                      n173 = Select(t=T12."Stop", s=w380, f=T12."Result") -> (s? t:f=w377:T12)
                    }
                    frame "MD[1]=1" {
                      n174 = Concatenate Strings(w440, "\nSet Parameters MD[1]=1" ("Strin")) -> (w429:string)
                      n175 = property on="VISA Tester" class="VISAName"() -> ("Value"=w445:refnum<visa-resource-name>)  [unwired: 2 in, 2 out]
                      n176 = call "TesterOption (SubVI).vi"("2 Options"=FALSE, "On/Off"=FALSE, "Tester Option"=T11."Venable", "VISA Refnum in"=w445) -> ("error out"=w446:errorcluster, "VISA Refnum out"=w436:refnum<visa-resource-name>)  [unwired: 6 in]
                      n177 = call "CANSendMotorSpeed.vi"("Remote"=TRUE, "error in (no error)"=w446, "Motor Speed RPM"=u16 0, "UUT"=w430, "CAN Cluster in"=w451) -> ("error out"=w448:errorcluster)  [unwired: 6 in]
                      n178 = call "Write panel message (SubVI).vi"("Stop BurnIn"=w431, 4:"rpm"=w419, 5:"rpm"=FALSE ("rpm"), "PrintTime"=TRUE, "Stop"=w421, "error in (no error)"=w448, "Time to wait"=40.0, "Strin"=w429, "String in"=w432) -> ("error out"=w418:errorcluster)  [unwired: 2 in]
                      n179 = property on="VISA Marvin" class="VISAName"(error in=w418) -> (error out=w447:errorcluster, "Value"=w453:refnum<visa-resource-name>)  [unwired: 1 in, 1 out]
                      n180 = call "SerialMarvinSendGet.vi"("error in (no error)"=w447, "Clear Log"=FALSE, "write buffer"="EP=1\r\nMD[1]=1\r\n", "VISA resource name"=w453) -> ("error out"=w435:errorcluster)  [unwired: 6 in, 1 out]
                      n181 = call "TesterOption (SubVI).vi"("2 Options"=FALSE, "error in (no error)"=w435, "On/Off"=FALSE, "Tester Option"=T11."Power", "VISA Refnum in"=w436) -> ("error out"=w433:errorcluster, "VISA Refnum out"=w422:refnum<visa-resource-name>)  [unwired: 5 in]
                      n182 = call "Write panel message (SubVI).vi"("Stop BurnIn"=w431, 4:"rpm"=w419, 5:"rpm"=FALSE ("rpm"), "PrintTime"=TRUE, "Stop"=w421, "error in (no error)"=w433, "Time to wait"=25.0, "Strin"=w429, "String in"=w432) -> ("error out"=w423:errorcluster)  [unwired: 2 in]
                      n183 = call "TesterOption (SubVI).vi"("2 Options"=FALSE, "error in (no error)"=w423, "On/Off"=TRUE, "Tester Option"=T11."Venable", "VISA Refnum in"=w422) -> ("error out"=w420:errorcluster)  [unwired: 5 in, 1 out]
                      n184 = call "Time Delay8"("error in (no error)"=w420) -> ("error out"=w416:errorcluster)  [unwired: 10 in]
                      n185 = property class="Bool (strict)"(reference=w421, error in=w416) -> ("Value"=w458:bool)  [unwired: 2 out]
                      n186 = Select(t=T12."Stop", s=w458, f=T12."FullSpeed2") -> (s? t:f=w457:T12)
                    }
                    frame "FullSpeed1" {
                      n187 = Concatenate Strings(w478, "\nFull speed operation " ("string")) -> (w463:string)
                      n188 = Equal?(x=w459, y=u8 95) -> (x = y?=w476:bool)
                      n189 = flat-sequence {
                        tunnel: w469 -> [w495]
                        tunnel: [w495] -> w468
                        tunnel: [w494] -> w467
                        frame #0 {
                          n190 = call <vilib>:"High Resolution Relative Seconds.vi"() -> ("relative seconds"=w494:dbl)
                        }
                      }
                      n191 = Select(t=u16 15100, s=w476, f=u16 12100 ("y")) -> (s? t:f=w483:u16)
                      n192 = call "CANSendMotorSpeed.vi"("Remote"=TRUE, "Motor Speed RPM"=w483, "UUT"=w484, "CAN Cluster in"=w488) -> ("error out"=w481:errorcluster)  [unwired: 7 in]
                      n193 = call "Write panel message (SubVI).vi"("Stop BurnIn"=w464, 4:"rpm"=w480, 5:"rpm"=TRUE ("rpm"), "PrintTime"=FALSE, "Stop"=w466, "error in (no error)"=w481, "Time to wait"=0.2, "Strin"=w463, "String in"=w465) -> ("error out"=w469:errorcluster)  [unwired: 2 in]
                      n194 = Select(t=13700.0, s=w476, f=11500.0) -> (s? t:f=w471:dbl)
                      n195 = Select(t=56.0, s=w476, f=33.0) -> (s? t:f=w470:dbl)
                      n196 = while {
                        tunnel: w480 -> [w497]
                        tunnel: w468 -> [w525]
                        tunnel: [w505] -> w479
                        tunnel: w471 -> [w517]
                        tunnel: w470 -> [w514]
                        tunnel: w467 -> [w512]
                        tunnel: w466 -> [w503]
                        tunnel: w465 -> [w504]
                        tunnel: w464 -> [w501]
                        tunnel: w463 -> [w500]
                        stop <- w519 stop-if-true
                        n197 = property class="DigNum (strict)"(reference=w497, error in=w525) -> (error out=w524:errorcluster, "Value"=w518:dbl)  [unwired: 1 out]
                        "FullSpeed1 Speed" <- w518
                        n198 = call <vilib>:"High Resolution Relative Seconds.vi"() -> ("relative seconds"=w513:dbl)
                        n199 = Subtract(x=w513, y=w512) -> (x-y=w511:dbl)
                        n200 = Greater Or Equal?(x=w511, y=120.0) -> (x >= y?=w509:bool)
                        n201 = Greater Or Equal?(x=w518, y=w517) -> (x >= y?=w516:bool)
                        n202 = property on="VISA Tester" class="VISAName"(error in=w524) -> (error out=w523:errorcluster, "Value"=w522:refnum<visa-resource-name>)  [unwired: 1 in, 1 out]
                        n203 = call "GetADCTester (SubVI).vi"("error in (no error)"=w523, "GetADCTester"=T13."Current", "TimeToGet"=5, "VISA Refnum in"=w522) -> ("error out"=w520:errorcluster, "ADCValOutput Single"=w515:dbl)  [unwired: 5 in, 1 out]
                        "FullSpeed1 Current" <- w515
                        n204 = Greater Or Equal?(x=w515, y=w514) -> (x >= y?=w506:bool)
                        n205 = And(x=w506, y=w516) -> (x .and. y?=w507:bool)
                        n206 = property class="Bool (strict)"(reference=w503) -> ("Value"=w508:bool)  [unwired: 1 in, 2 out]
                        n207 = call "Write panel message (SubVI).vi"("Stop BurnIn"=w501, 4:"rpm"=w497, 5:"rpm"=TRUE ("rpm"), "PrintTime"=FALSE, "Stop"=w503, "error in (no error)"=w520, "Time to wait"=0.2, "Strin"=w500, "String in"=w504) -> ("error out"=w505:errorcluster)  [unwired: 2 in]
                        n208 = Compound Arithmetic op=OR(w508, w507, w509) -> (w519:bool)
                      }
                      n209 = property class="Bool (strict)"(reference=w466, error in=w479) -> ("Value"=w493:bool)  [unwired: 2 out]
                      n210 = Select(t=T12."Stop", s=w493, f=T12."MD[1]=1") -> (s? t:f=w490:T12)
                    }
                    frame "MD[1]=0" {
                      n211 = Concatenate Strings(w552, "\nSet Parameters MD[1]=0" ("Strin")) -> (w541:string)
                      n212 = property on="VISA Tester" class="VISAName"() -> ("Value"=w558:refnum<visa-resource-name>)  [unwired: 2 in, 2 out]
                      n213 = call "TesterOption (SubVI).vi"("2 Options"=FALSE, "On/Off"=FALSE, "Tester Option"=T11."Venable", "VISA Refnum in"=w558) -> ("error out"=w559:errorcluster, "VISA Refnum out"=w548:refnum<visa-resource-name>)  [unwired: 6 in]
                      n214 = call "CANSendMotorSpeed.vi"("Remote"=TRUE, "error in (no error)"=w559, "Motor Speed RPM"=u16 0, "UUT"=w542, "CAN Cluster in"=w564) -> ("error out"=w561:errorcluster)  [unwired: 6 in]
                      n215 = call "Write panel message (SubVI).vi"("Stop BurnIn"=w543, 4:"rpm"=w538, 5:"rpm"=FALSE ("rpm"), "PrintTime"=FALSE, "Stop"=w532, "error in (no error)"=w561, "Time to wait"=0.2, "Strin"=w541, "String in"=w544) -> ("error out"=w555:errorcluster)  [unwired: 2 in]
                      n216 = property on="VISA Marvin" class="VISAName"(error in=w555) -> (error out=w560:errorcluster, "Value"=w566:refnum<visa-resource-name>)  [unwired: 1 in, 1 out]
                      n217 = call "SerialMarvinSendGet.vi"("error in (no error)"=w560, "Clear Log"=FALSE, "write buffer"="EP=1\r\nMD[1]=0\r\n", "VISA resource name"=w566) -> ("error out"=w547:errorcluster)  [unwired: 6 in, 1 out]
                      n218 = call "TesterOption (SubVI).vi"("2 Options"=FALSE, "error in (no error)"=w547, "On/Off"=FALSE, "Tester Option"=T11."Power", "VISA Refnum in"=w548) -> ("error out"=w545:errorcluster, "VISA Refnum out"=w533:refnum<visa-resource-name>)  [unwired: 5 in]
                      n219 = call "Write panel message (SubVI).vi"("Stop BurnIn"=w543, 4:"rpm"=w538, 5:"rpm"=FALSE ("rpm"), "PrintTime"=TRUE, "Stop"=w532, "error in (no error)"=w545, "Time to wait"=25.0, "Strin"=w541, "String in"=w544) -> ("error out"=w534:errorcluster)  [unwired: 2 in]
                      n220 = call "TesterOption (SubVI).vi"("2 Options"=FALSE, "error in (no error)"=w534, "On/Off"=TRUE, "Tester Option"=T11."Venable", "VISA Refnum in"=w533) -> ("error out"=w531:errorcluster)  [unwired: 5 in, 1 out]
                      n221 = call "Time Delay4"("error in (no error)"=w531) -> ("error out"=w527:errorcluster)  [unwired: 10 in]
                      n222 = property class="Bool (strict)"(reference=w532, error in=w527) -> ("Value"=w571:bool)  [unwired: 2 out]
                      n223 = Select(t=T12."Stop", s=w571, f=T12."FullSpeed1") -> (s? t:f=w570:T12)
                    }
                  }
                }
                n224 = flat-sequence {
                  tunnel: [enum16{"Stop", "Direction", "Venable", "Start"}."Stop"] -> w290
                  tunnel: w289 -> [_]
                  frame #0 {
                  }
                }
              }
              frame "Venable" {
                n225 = call "Find_Number_LineMARVIN.vi"("Test Paragraph"="4.1", "TableIn"=w575) -> ("Line number"=w583:i32)  [unwired: 3 in, 3 out]
                n226 = for {
                  tunnel: u16[] [5000, 0, 5000] -> [w613] mode=indexing
                  tunnel: bool[] [TRUE, FALSE, TRUE] -> [w608] mode=indexing
                  tunnel: w583 -> [w614]
                  tunnel: w582 -> [w612]
                  tunnel: w581 -> [w611]
                  tunnel: w580 -> [w599]
                  tunnel: w579 -> [w603]
                  tunnel: w577 -> [w602]
                  tunnel: w578 -> [w601]
                  tunnel: w575 -> [w595]
                  tunnel: w574 -> [w593]
                  tunnel: [w592] -> w573 mode=indexing
                  i -> [w615]
                  w617 = 200.0 ("y")
                  n227 = call "CANSendMotorSpeed.vi"("Remote"=TRUE, "Motor Speed RPM"=u16 5000, "UUT"=w611, "CAN Cluster in"=w612) -> ("error out"=w607:errorcluster)  [unwired: 7 in]
                  n228 = property on="VISA Tester" class="VISAName"() -> ("Value"=w606:refnum<visa-resource-name>)  [unwired: 2 in, 2 out]
                  n229 = Add(x=w614, y=w615) -> (x+y=w596:i32)
                  n230 = call "TesterOption (SubVI).vi"("2 Options"=FALSE, "error in (no error)"=w607, "On/Off"=w608, "Tester Option"=T11."Venable", "VISA Refnum in"=w606) -> ("error out"=w605:errorcluster)  [unwired: 5 in, 1 out]
                  n231 = call "Write panel message (SubVI).vi"("Stop BurnIn"=w601, 4:"rpm"=w599, 5:"rpm"=TRUE ("rpm"), "PrintTime"=TRUE, "Stop"=w602, "error in (no error)"=w605, "Time to wait"=15.0, "Strin"=w593, "String in"=w603) -> ("error out"=w604:errorcluster)  [unwired: 2 in]
                  n232 = property class="DigNum (strict)"(reference=w599, error in=w604) -> ("Value"=w594:dbl)  [unwired: 2 out]
                  n233 = Add(x=w613, y=w617) -> (x+y=w619:dbl)
                  n234 = Subtract(x=w613, y=w617) -> (x-y=w618:dbl)
                  n235 = In Range and Coerce(upper limit=w619, x=w594, lower limit=w618) -> (In Range?=w592:bool)  [unwired: 1 out]
                  n236 = call "PassOrFail (SubVI).vi"("index (row)"=w596, "Data in"=w594, "Pass?Fail"=w592, "Table in"=w595) -> ()  [unwired: 7 in, 1 out]
                }
                n237 = property class="Bool (strict)"(reference=w577) -> ("Value"=w590:bool)  [unwired: 1 in, 2 out]
                n238 = And Array Elements(Boolean array=w573) -> (logical AND=→"VenableResult":bool)
                n239 = Select(t=enum16{"Stop", "Direction", "Venable", "Start"}."Stop", s=w590, f=enum16{"Stop", "Direction", "Venable", "Start"}."Direction") -> (s? t:f=w576:enum16{"Stop", "Direction", "Venable", "Start"})
              }
              frame "Start" {
                w639 = "4" ("Test Paragraph")
                n240 = property class="Str"(reference=w630, "Value"=w621) -> (reference out=w640:refnum<vi>, error out=w627:errorcluster)  [unwired: 1 in]
                n241 = call "Table_ScrollaBarMarvin.vi"("error in"=w627, "Line to focus"=w639, "reference in"=w631) -> ("error out"=w636:errorcluster)  [unwired: 2 out]
                n242 = call "Reset old test Values (SubVI).vi"("error in"=w636, "Atr in"=w631, "Test Paragraph"=w639) -> ("error out"=w635:errorcluster)  [unwired: 8 in]
                n243 = property on="VISA Tester" class="VISAName"(error in=w635) -> (error out=w634:errorcluster, "Value"=w633:refnum<visa-resource-name>)  [unwired: 1 in, 1 out]
                n244 = property class="Bool (strict)"(reference=w624) -> ("Value"=w644:bool)  [unwired: 1 in, 2 out]
                n245 = call "TesterOption (SubVI).vi"("2 Options"=FALSE, "error in (no error)"=w634, "On/Off"=TRUE, "Tester Option"=T11."Venable", "VISA Refnum in"=w633) -> ("error out"=w632:errorcluster)  [unwired: 5 in, 1 out]
                n246 = Select(t=enum16{"Stop", "Direction", "Venable", "Start"}."Stop", s=w644, f=enum16{"Stop", "Direction", "Venable", "Start"}."Venable") -> (s? t:f=w628:enum16{"Stop", "Direction", "Venable", "Start"})
                n247 = call "Write panel message (SubVI).vi"("Stop BurnIn"=w623, 4:"rpm"=w622, 5:"rpm"=FALSE ("rpm"), "PrintTime"=FALSE, "Stop"=w624, "error in (no error)"=w632, "Time to wait"=0.2, "Strin"=w621, "String in"=w640) -> ()  [unwired: 2 in, 1 out]
              }
            }
          }
        }
        frame "Speed Command" {
          w649 = "5. Speed Command Test in process..." ("Value")
          w646 = "5" ("Test Paragraph")
          n248 = control-ref of="Pannel User Message"() -> (w661:refnum<vi>)
          n249 = property class="Str"(reference=w661, error in=w660, "Value"=w649) -> (error out=w659:errorcluster)  [unwired: 1 out]
          n250 = call "Table_ScrollaBarMarvin.vi"("error in"=w659, "Line to focus"=w646, "reference in"=w645) -> ("error out"=w662:errorcluster)  [unwired: 2 out]
          n251 = property class="Tbl (strict)"(reference=w645, error in=w662) -> (error out=w664:errorcluster, "Value"=w665:string[][])  [unwired: 1 out]
          n252 = Index Array(array=w665, index (col)=0 ("disabled index (col)")) -> (element=w666:string[])  [unwired: 1 in]
          n253 = call "Find_Number_Line.vi"("error in"=w664, "Test Paragraph"=w646, "Row Headers[]"=w666) -> ("error out"=w647:errorcluster, "Line number"=w650:i32)  [unwired: 1 out]
          n254 = call "Reset old test Values (SubVI).vi"("error in"=w647, "Atr in"=w645, "Test Paragraph"=w646) -> ()  [unwired: 8 in, 1 out]
          n255 = control-ref of="Pannel User Message"() -> (w654:refnum<vi>)
          n256 = control-ref of="Stop Burn-in"() -> (w658:refnum<vi>)
          n257 = control-ref of="Config_CANAT"() -> (w655:refnum<vi>)
          n258 = control-ref of="Motor Speed RPM"() -> (w656:refnum<vi>)
          n259 = control-ref of="UUT"() -> (w657:refnum<vi>)
          n260 = control-ref of="Stop Button"() -> (w652:refnum<vi>)
          n261 = control-ref of="ATR"() -> (w653:refnum<vi>)
          n262 = property on="UUT" class="DigNum (strict)"() -> ("Value"=w648:u8)  [unwired: 2 in, 2 out]
          n263 = while {
            shift-right: [w678] -> _
            shift-left: enum16{"Stop", "StopTime", "Speeds", "Start"}."Start" -> [w679]
            tunnel: w652 -> [w677]
            tunnel: w653 -> [w676]
            tunnel: w654 -> [w675]
            tunnel: w655 -> [w674]
            tunnel: w656 -> [w673]
            tunnel: w657 -> [w672]
            tunnel: w658 -> [w671]
            tunnel: w650 -> [w670]
            tunnel: w649 -> [w669]
            tunnel: w648 -> [w667]
            stop <- w668 stop-if-true
            n264 = case shown="\"Start\"" w679 {
              tunnel: [w683 w712 w753 w797] -> w678
              tunnel: w677 -> [_ w707 w757 w795]
              tunnel: w676 -> [_ w697 w761 _]
              tunnel: w675 -> [_ w708 w758 _]
              tunnel: w674 -> [w681 w710 w760 _]
              tunnel: w673 -> [_ w705 w755 _]
              tunnel: w672 -> [w682 w709 w752 _]
              tunnel: w671 -> [_ w706 w756 _]
              tunnel: w670 -> [_ _ w762 _]
              tunnel: w669 -> [_ _ w759 _]
              tunnel: [w680 w711 w754 FALSE ("Value")] -> w668
              tunnel: w667 -> [_ _ w745 _]
              frame "Stop", Default {
                n265 = flat-sequence {
                  tunnel: w682 -> [w686]
                  tunnel: w681 -> [w685]
                  tunnel: [enum16{"Stop", "StopTime", "Speeds", "Start"}."Stop"] -> w683
                  tunnel: [TRUE] -> w680
                  frame #0 {
                    n266 = call "CANSendMotorSpeed.vi"("Remote"=TRUE, "Motor Speed RPM"=u16 0, "UUT"=w686, "CAN Cluster in"=w685) -> ("error out"=w691:errorcluster)  [unwired: 7 in]
                    n267 = property on="VISA Tester" class="VISAName"() -> ("Value"=w692:refnum<visa-resource-name>)  [unwired: 2 in, 2 out]
                    n268 = call "TesterOption (SubVI).vi"("2 Options"=FALSE, "error in (no error)"=w691, "On/Off"=FALSE, "Tester Option"=T11."Venable", "VISA Refnum in"=w692) -> ()  [unwired: 5 in, 2 out]
                  }
                  frame #1 {
                  }
                }
              }
              frame "StopTime" {
                n269 = call "Table_ScrollaBarMarvin.vi"("Line to focus"="6", "reference in"=w697) -> ("error out"=w698:errorcluster)  [unwired: 1 in, 2 out]
                n270 = call "CANSendMotorSpeed.vi"("Remote"=TRUE, "error in (no error)"=w698, "Motor Speed RPM"=u16 0, "UUT"=w709, "CAN Cluster in"=w710) -> ("error out"=w716:errorcluster)  [unwired: 6 in]
                n271 = flat-sequence {
                  tunnel: [w742] -> w715
                  tunnel: w716 -> [w741]
                  tunnel: [w741] -> w717
                  frame #0 {
                    n272 = call <vilib>:"High Resolution Relative Seconds.vi"() -> ("relative seconds"=w742:dbl)
                  }
                }
                n273 = while {
                  tunnel: [w737] -> w711
                  tunnel: w708 -> [w735]
                  tunnel: w707 -> [w734]
                  tunnel: w706 -> [w732]
                  tunnel: w705 -> [w731]
                  tunnel: "6. Stop Time Test in process..." ("Value") -> [w719]
                  tunnel: [w727] -> w695
                  tunnel: w717 -> [w739]
                  tunnel: [w728] -> w703
                  tunnel: w715 -> [w738]
                  tunnel: [w726] -> w699
                  stop <- w718 stop-if-true
                  n274 = call "Write panel message (SubVI).vi"("Stop BurnIn"=w732, 4:"rpm"=w731, 5:"rpm"=TRUE ("rpm"), "PrintTime"=FALSE, "Stop"=w734, "error in (no error)"=w739, "Time to wait"=0.1, "Strin"=w719, "String in"=w735) -> ("error out"=w736:errorcluster)  [unwired: 2 in]
                  n275 = control-ref of="Motor Speed RPM"() -> (w725:refnum<vi>)
                  n276 = property class="DigNum (strict)"(reference=w725, error in=w736) -> (error out=w728:errorcluster, "Value"=w724:dbl)  [unwired: 1 out]
                  n277 = call <vilib>:"High Resolution Relative Seconds.vi"() -> ("relative seconds"=w722:dbl)
                  n278 = property class="Bool (strict)"(reference=w734) -> ("Value"=w737:bool)  [unwired: 1 in, 2 out]
                  n279 = Subtract(x=w722, y=w738) -> (x-y=w726:dbl)
                  n280 = Greater Or Equal?(x=w726, y=50.0) -> (x >= y?=w720:bool)
                  n281 = Less Or Equal?(x=w724, y=0.0) -> (x <= y?=w727:bool)
                  n282 = Compound Arithmetic op=OR(w727, w720, w737) -> (w718:bool)
                }
                "StopTimeResult" <- w695
                n283 = call "Find_Number_LineMARVIN.vi"("Test Paragraph"="6", "TableIn"=w697) -> ("Line number"=w700:i32)  [unwired: 3 in, 3 out]
                n284 = call "PassOrFail (SubVI).vi"("index (row)"=w700, "error in (no error)"=w703, "Data in"=w699, "Pass?Fail"=w695, "Table in"=w697) -> ("error out"=w702:errorcluster)  [unwired: 6 in]
                n285 = flat-sequence {
                  tunnel: [enum16{"Stop", "StopTime", "Speeds", "Start"}."Stop"] -> w712
                  tunnel: w702 -> [_]
                  frame #0 {
                  }
                }
              }
              frame "Speeds" {
                n286 = Equal?(x=w745, y=u8 95) -> (x = y?=w750:bool)
                n287 = Select(t=u16[] [6000, 11500, 15100], s=w750, f=u16[] [6000, 9000, 12100]) -> (s? t:f=w747:u16[])
                n288 = for {
                  tunnel: w747 -> [w788] mode=indexing
                  tunnel: w762 -> [w781]
                  tunnel: w761 -> [w780]
                  tunnel: w752 -> [w779]
                  tunnel: w760 -> [w778]
                  tunnel: w759 -> [w777]
                  tunnel: w758 -> [w776]
                  tunnel: w757 -> [w775]
                  tunnel: w756 -> [w773]
                  tunnel: w755 -> [w771]
                  tunnel: [w769] -> w754
                  tunnel: [w768] -> w746
                  tunnel: [w767] -> w744 mode=indexing
                  i -> [w787]
                  stop <- w769 stop-if-true
                  w789 = 200.0 ("y")
                  n289 = Increment(x=w787) -> (x+1=w786:i32)
                  n290 = Add(x=w781, y=w786) -> (x+y=w782:i32)
                  n291 = call "CANSendMotorSpeed.vi"("Remote"=TRUE, "Motor Speed RPM"=w788, "UUT"=w779, "CAN Cluster in"=w778) -> ("error out"=w793:errorcluster)  [unwired: 7 in]
                  n292 = control-ref of="Motor Speed RPM"() -> (w794:refnum<vi>)
                  n293 = call "Write panel message (SubVI).vi"("Stop BurnIn"=w773, 4:"rpm"=w771, 5:"rpm"=TRUE ("rpm"), "PrintTime"=TRUE, "Stop"=w775, "error in (no error)"=w793, "Time to wait"=25.0 ("Delay Time (sec)"), "Strin"=w777, "String in"=w776) -> ("error out"=w785:errorcluster)  [unwired: 2 in]
                  n294 = property class="DigNum (strict)"(reference=w794, error in=w785) -> (error out=w792:errorcluster, "Value"=w770:dbl)  [unwired: 1 out]
                  n295 = property class="Bool (strict)"(reference=w775) -> ("Value"=w769:bool)  [unwired: 1 in, 2 out]
                  n296 = Add(x=w788, y=w789) -> (x+y=w791:dbl)
                  n297 = Subtract(x=w788, y=w789) -> (x-y=w790:dbl)
                  n298 = In Range and Coerce(upper limit=w791, x=w770, lower limit=w790) -> (In Range?=w767:bool)  [unwired: 1 out]
                  n299 = call "PassOrFail (SubVI).vi"("index (row)"=w782, "error in (no error)"=w792, "Data in"=w770, "Pass?Fail"=w767, "Table in"=w780) -> ("error out"=w768:errorcluster)  [unwired: 6 in]
                }
                n300 = flat-sequence {
                  tunnel: w754 -> [w766]
                  tunnel: [w764] -> w753
                  tunnel: w746 -> [_]
                  frame #0 {
                    n301 = Select(t=enum16{"Stop", "StopTime", "Speeds", "Start"}."Stop", s=w766, f=enum16{"Stop", "StopTime", "Speeds", "Start"}."StopTime") -> (s? t:f=w764:enum16{"Stop", "StopTime", "Speeds", "Start"})
                  }
                }
                n302 = And Array Elements(Boolean array=w744) -> (logical AND=→"SpeedResult":bool)
              }
              frame "Start" {
                n303 = property on="VISA Tester" class="VISAName"() -> ("Value"=w805:refnum<visa-resource-name>)  [unwired: 2 in, 2 out]
                n304 = call "TesterOption (SubVI).vi"("2 Options"=FALSE, "On/Off"=TRUE, "Tester Option"=T11."Venable", "VISA Refnum in"=w805) -> ("error out"=w796:errorcluster)  [unwired: 6 in, 1 out]
                n305 = property class="Bool (strict)"(reference=w795, error in=w796) -> ("Value"=w801:bool)  [unwired: 2 out]
                n306 = Select(t=enum16{"Stop", "StopTime", "Speeds", "Start"}."Stop", s=w801, f=enum16{"Stop", "StopTime", "Speeds", "Start"}."Speeds") -> (s? t:f=w797:enum16{"Stop", "StopTime", "Speeds", "Start"})
              }
            }
          }
        }
        frame "Stop Time" {
          w809 = "3. Motor Temperature test in process..." ("Value")
          w807 = "3" ("Test Paragraph")
          n307 = control-ref of="Pannel User Message"() -> (w817:refnum<vi>)
          n308 = property class="Str"(reference=w817, error in=w816, "Value"=w809) -> (error out=w815:errorcluster)  [unwired: 1 out]
          n309 = call "Table_ScrollaBarMarvin.vi"("error in"=w815, "Line to focus"=w807, "reference in"=w806) -> ("error out"=w819:errorcluster)  [unwired: 2 out]
          n310 = property class="Tbl (strict)"(reference=w806, error in=w819) -> (reference out=w812:refnum<vi>, error out=w821:errorcluster, "Value"=w822:string[][])
          n311 = Index Array(array=w822, index (col)=0 ("disabled index (col)")) -> (element=w823:string[])  [unwired: 1 in]
          n312 = call "Find_Number_LineMARVIN.vi"("Test Paragraph"=w807, "error in"=w821, "TableIn"=w806, "Row Headers[]"=w823) -> ("error out"=w818:errorcluster, "Line number"=w811:i32)  [unwired: 1 in, 2 out]
          n313 = call "Reset old test Values (SubVI).vi"("error in"=w818, "Atr in"=w806, "Test Paragraph"=w807) -> ("error out"=w808:errorcluster)  [unwired: 8 in]
          n314 = property on="Status" class="Bool (strict)"(error in=w808) -> (error out=w813:errorcluster, "Value"=w814:bool)  [unwired: 1 in, 1 out]
          n315 = case shown="True" w814 {
            selector: w814 -> [w827 _]
            tunnel: w813 -> [w829 _]
            tunnel: w812 -> [w826 _]
            tunnel: w811 -> [w825 w832]
            tunnel: w810 -> [_ w837]
            tunnel: w809 -> [_ w833]
            frame False {
              n316 = flat-sequence {
                tunnel: w829 -> [w830]
                tunnel: [w830] -> w828
                frame #0 {
                  n317 = One Button Dialog(message="Please establish RS connection.") -> ()  [unwired: 1 in, 1 out]
                }
              }
              n318 = Increment(x=w825) -> (x+1=w824:i32)
              n319 = call "PassOrFail (SubVI).vi"("index (row)"=w824, "error in (no error)"=w828, "Pass?Fail"=w827, "Table in"=w826) -> ()  [unwired: 7 in, 1 out]
            }
            frame True {
              n320 = control-ref of="Stop Burn-in"() -> (w839:refnum<vi>)
              n321 = control-ref of="Pannel User Message"() -> (w841:refnum<vi>)
              n322 = control-ref of="Config_CANAT"() -> (w835:refnum<vi>)
              n323 = control-ref of="ATR"() -> (w842:refnum<vi>)
              n324 = control-ref of="Motor Speed RPM"() -> (w843:refnum<vi>)
              n325 = control-ref of="UUT"() -> (w834:refnum<vi>)
              n326 = control-ref of="Stop Button"() -> (w840:refnum<vi>)
              n327 = property on="VISA Tester" class="VISAName"() -> ("Value"=w836:refnum<visa-resource-name>)  [unwired: 2 in, 2 out]
              n328 = while {
                shift-right: [w847] -> _
                shift-left: T14."Start" -> [w857]
                tunnel: w839 -> [w856]
                tunnel: w840 -> [w855]
                tunnel: w841 -> [w854]
                tunnel: w842 -> [w853]
                tunnel: w843 -> [w852]
                tunnel: w837 -> [w851]
                tunnel: w836 -> [w850]
                tunnel: w835 -> [w849]
                tunnel: w834 -> [w848]
                tunnel: w833 -> [w845]
                tunnel: w832 -> [w844]
                stop <- w846 stop-if-true
                n329 = case shown="\"Start\"" w857 {
                  tunnel: w856 -> [_ w880 w939]
                  tunnel: w855 -> [_ w872 w941]
                  tunnel: w854 -> [_ w881 w943]
                  tunnel: w853 -> [_ w870 _]
                  tunnel: w852 -> [_ w879 w938]
                  tunnel: w851 -> [_ w884 _]
                  tunnel: w850 -> [w860 w883 w932]
                  tunnel: w849 -> [_ _ w949]
                  tunnel: w848 -> [_ _ w948]
                  tunnel: [w858 w873 w934] -> w847
                  tunnel: [w859 FALSE FALSE] -> w846
                  tunnel: w845 -> [_ w882 _]
                  tunnel: w844 -> [_ w869 _]
                  frame "Stop", Default {
                    n330 = flat-sequence {
                      tunnel: w860 -> [w861]
                      tunnel: [TRUE] -> w859
                      tunnel: [T14."Stop"] -> w858
                      frame #0 {
                        n331 = call "TesterOption (SubVI).vi"("2 Options"=FALSE, "On/Off"=FALSE, "Tester Option"=T11."Venable", "VISA Refnum in"=w861) -> ()  [unwired: 6 in, 2 out]
                      }
                      frame #1 {
                      }
                    }
                  }
                  frame "TA[5]" {
                    w885 = T17 [enum."60C", enum."90C", enum."120C"] items=["K15", "K16", "K17", "Venable", "Firmeware", "Fan", "Power", "120C", "110C", "100C", "90C", "80C", "70C", "60C", "50C", "40C", "30C", "25C", "20C", "10C", "0C"]
                    n332 = for {
                      tunnel: w885 -> [w909] mode=indexing
                      tunnel: w884 -> [w908]
                      tunnel: w883 -> [w907]
                      tunnel: w882 -> [w906]
                      tunnel: w881 -> [w905]
                      tunnel: w872 -> [w904]
                      tunnel: w880 -> [w903]
                      tunnel: w879 -> [w902]
                      tunnel: dbl[] [60.0, 90.0, 120.0] -> [w892] mode=indexing
                      tunnel: [w891] -> w871
                      tunnel: w870 -> [w898]
                      tunnel: w869 -> [w897]
                      tunnel: [w886] -> w868 mode=indexing
                      i -> [w895]
                      w890 = 3.0 ("y")
                      n333 = for {
                        N: 5 -> [_]
                        tunnel: w909 -> [w911]
                        tunnel: w908 -> [w927]
                        tunnel: w907 -> [w923]
                        tunnel: w906 -> [w921]
                        tunnel: w905 -> [w920]
                        tunnel: w904 -> [w919]
                        tunnel: w903 -> [w917]
                        tunnel: w902 -> [w914]
                        tunnel: [w913] -> w901 mode=indexing
                        tunnel: [w912] -> w899
                        n334 = call "TesterOption (SubVI).vi"("2 Options"=FALSE, "On/Off"=TRUE, "Tester Option"=w911, "VISA Refnum in"=w923) -> ("error out"=w924:errorcluster)  [unwired: 6 in, 1 out]
                        n335 = call "Write panel message (SubVI).vi"("Stop BurnIn"=w917, 4:"rpm"=w914, 5:"rpm"=FALSE ("rpm"), "PrintTime"=FALSE, "Stop"=w919, "error in (no error)"=w924, "Time to wait"=1.0, "Strin"=w921, "String in"=w920) -> ("error out"=w922:errorcluster)  [unwired: 2 in]
                        n336 = call "SerialMarvinSendGet.vi"("error in (no error)"=w922, "write buffer"="TA[2]\r\n", "VISA resource name"=w927) -> ("error out"=w912:errorcluster, "read buffer"=w925:string)  [unwired: 7 in]
                        n337 = Fract/Exp String To Number(string=w925) -> (number=w913:dbl)  [unwired: 3 in, 1 out]
                      }
                      n338 = Increment(x=w895) -> (x+1=w894:i32)
                      n339 = Add Array Elements(numeric array=w901) -> (sum=w900:dbl)
                      n340 = Add(x=w892, y=w890) -> (x+y=w889:dbl)
                      n341 = Subtract(x=w892, y=w890) -> (x-y=w888:dbl)
                      n342 = Divide(x=w900, y=5.0) -> (x/y=w887:dbl)
                      n343 = In Range and Coerce(upper limit=w889, x=w887, lower limit=w888) -> (In Range?=w886:bool)  [unwired: 1 out]
                      n344 = Add(x=w897, y=w894) -> (x+y=w896:i32)
                      n345 = call "PassOrFail (SubVI).vi"("index (row)"=w896, "error in (no error)"=w899, "Data in"=w887, "Pass?Fail"=w886, "Table in"=w898) -> ("error out"=w891:errorcluster)  [unwired: 6 in]
                    }
                    n346 = property class="Bool (strict)"(reference=w872, error in=w871) -> ("Value"=w877:bool)  [unwired: 2 out]
                    n347 = Select(t=T14."Stop", s=w877, f=T14."Stop") -> (s? t:f=w873:T14)
                    n348 = And Array Elements(Boolean array=w868) -> (logical AND=→"MotorTempResult":bool)
                  }
                  frame "Start" {
                    n349 = call "Write panel message (SubVI).vi"("Stop BurnIn"=w939, 4:"rpm"=w938, 5:"rpm"=FALSE ("rpm"), "PrintTime"=FALSE, "Stop"=w941, "Time to wait"=0.1, "Strin"="3. Motor Temperature test in process...\nInitialization state...", "String in"=w943) -> ("error out"=w944:errorcluster)  [unwired: 3 in]
                    n350 = call "TesterOption (SubVI).vi"("2 Options"=FALSE, "error in (no error)"=w944, "On/Off"=FALSE, "Tester Option"=T11."Venable", "VISA Refnum in"=w932) -> ("error out"=w946:errorcluster)  [unwired: 5 in, 1 out]
                    n351 = call "CANSendMotorSpeed.vi"("Remote"=TRUE, "error in (no error)"=w946, "Motor Speed RPM"=u16 0, "UUT"=w948, "CAN Cluster in"=w949) -> ("error out"=w931:errorcluster)  [unwired: 6 in]
                    n352 = property class="Bool (strict)"(reference=w941, error in=w931) -> ("Value"=w953:bool)  [unwired: 2 out]
                    n353 = Select(t=T14."Stop", s=w953, f=T14."TA[5]") -> (s? t:f=w934:T14)
                  }
                }
              }
            }
          }
        }
        frame "Temp Control" {
          w971 = "7. Temperature control test in process..." ("Value")
          w969 = "7" ("Test Paragraph")
          n354 = control-ref of="Pannel User Message"() -> (w982:refnum<vi>)
          n355 = call <vilib>:"Open Config Data.vi"("error in (no error)"=w965, "create file if necessary (T)"=FALSE, "configuration file path"=w967) -> ("error out"=w968:errorcluster, "refnum"=w964:T18)  [unwired: 7 out]
          n356 = property class="Str"(reference=w982, error in=w965, "Value"=w971) -> (error out=w981:errorcluster)  [unwired: 1 out]
          n357 = call-poly <vilib>:"Read Key.vi"("section"="Marvin", "error in (no error)"=w968, "default value"="10", "key"="Temp Algorithm", "refnum"=w964) -> ("error out"=w960:errorcluster, "value"=w958:string, "refnum out"=w959:T18)  [unwired: 1 in, 3 out]
          n358 = Decimal String To Number(string=w958) -> (number=w956:i32)  [unwired: 2 in, 1 out]
          n359 = Less Or Equal To 0?(x=w956) -> (x <= 0?=w957:bool)
          n360 = Select(t=10, s=w957, f=w956) -> (s? t:f=w955:i32)
          n361 = call <vilib>:"Close Config Data.vi"("error in (no error)"=w960, "refnum"=w959) -> ()  [unwired: 8 in, 2 out]
          n362 = control-ref of="Pannel User Message"() -> (w976:refnum<vi>)
          n363 = control-ref of="Motor Speed RPM"() -> (w974:refnum<vi>)
          n364 = control-ref of="Stop Button"() -> (w978:refnum<vi>)
          n365 = control-ref of="ATR"() -> (w977:refnum<vi>)
          n366 = control-ref of="Config_CANAT"() -> (w975:refnum<vi>)
          n367 = control-ref of="UUT"() -> (w973:refnum<vi>)
          n368 = control-ref of="Stop Burn-in"() -> (w972:refnum<vi>)
          n369 = call "Table_ScrollaBarMarvin.vi"("error in"=w981, "Line to focus"=w969, "reference in"=w983) -> ("error out"=w980:errorcluster)  [unwired: 2 out]
          n370 = call "Reset old test Values (SubVI).vi"("error in"=w980, "Atr in"=w983, "Test Paragraph"=w969) -> ("error out"=w970:errorcluster)  [unwired: 8 in]
          n371 = while {
            tunnel: w970 -> [w996]
            shift-right: [w994] -> _
            shift-left: enum16{"Stop", "Algorithm", "Start"}."Start" -> [w995]
            tunnel: w978 -> [w993]
            tunnel: w977 -> [w992]
            tunnel: w976 -> [w991]
            tunnel: w975 -> [w990]
            tunnel: w974 -> [w989]
            tunnel: w973 -> [w988]
            tunnel: w972 -> [w986]
            tunnel: w971 -> [w985]
            tunnel: w955 -> [w984]
            stop <- w987 stop-if-true
            n372 = case shown="\"Algorithm\"" w995 {
              tunnel: w996 -> [_ _ w1120]
              tunnel: [w997 w1018 w1109] -> w994
              tunnel: w993 -> [_ w1029 w1113]
              tunnel: w992 -> [_ w1025 _]
              tunnel: w991 -> [_ w1030 _]
              tunnel: w990 -> [w1000 _ w1106]
              tunnel: w989 -> [_ w1026 _]
              tunnel: w988 -> [w999 _ w1105]
              tunnel: [w998 FALSE FALSE] -> w987
              tunnel: w986 -> [_ w1028 _]
              tunnel: w985 -> [_ w1027 _]
              tunnel: w984 -> [_ w1012 _]
              frame "Stop", Default {
                n373 = flat-sequence {
                  tunnel: w1000 -> [w1005]
                  tunnel: w999 -> [w1003]
                  tunnel: [TRUE] -> w998
                  tunnel: [enum16{"Stop", "Algorithm", "Start"}."Stop"] -> w997
                  frame #0 {
                    n374 = call "CANSendMotorSpeed.vi"("Remote"=TRUE, "Motor Speed RPM"=u16 0, "UUT"=w1003, "CAN Cluster in"=w1005) -> ("error out"=w1001:errorcluster)  [unwired: 7 in]
                    n375 = property on="VISA Tester" class="VISAName"() -> ("Value"=w1009:refnum<visa-resource-name>)  [unwired: 2 in, 2 out]
                    n376 = call "TesterOption (SubVI).vi"("2 Options"=FALSE, "error in (no error)"=w1001, "On/Off"=FALSE, "Tester Option"=T11."Venable", "VISA Refnum in"=w1009) -> ()  [unwired: 5 in, 2 out]
                  }
                  frame #1 {
                  }
                  frame #2 {
                  }
                }
              }
              frame "Algorithm" {
                w1013 = T19 [enum."6000", enum."11500", enum."15100", enum."11500-2", enum."6000-2"] items=["6000", "11500", "15100", "11500-2", "6000-2"]
                # "Speed Goal"
                # "Speed Ind"
                # "Temp Goal"
                # "50 Deg"
                n377 = for {
                  tunnel: w1030 -> [w1058]
                  tunnel: w1029 -> [w1057]
                  tunnel: w1028 -> [w1056]
                  tunnel: w1027 -> [w1055]
                  tunnel: w1026 -> [w1054]
                  tunnel: w1025 -> [w1041]
                  tunnel: string[] ["7.1", "7.3", "7.5", "7.7", "7.9"] -> [w1039] mode=indexing
                  shift-right: [w1051] -> _
                  shift-left: 1202.0 ("Rt") -> [w1052]
                  tunnel: dbl[] [68.0, 68.0, 88.0, 80.0, 60.0] -> [w1050] mode=indexing
                  tunnel: dbl[] [6000.0, 11500.0, 15100.0, 11500.0, 6000.0] -> [w1049] mode=indexing
                  tunnel: dbl[] [6000.0, 6400.0, 11700.0, 14600.0, 11000.0] -> [w1048] mode=indexing
                  tunnel: [w1037] -> w1019
                  tunnel: [w1036] -> w1015 mode=indexing
                  tunnel: [w1035] -> w1016 mode=indexing
                  tunnel: w1013 -> [w1034] mode=indexing
                  tunnel: w1012 -> [w1033]
                  stop <- w1053 stop-if-true
                  n378 = call <vilib>:"High Resolution Relative Seconds.vi"() -> ("relative seconds"=w1047:dbl)
                  n379 = while {
                    tunnel: w1058 -> [w1087]
                    tunnel: w1057 -> [w1079]
                    tunnel: w1056 -> [w1086]
                    tunnel: w1055 -> [w1065]
                    tunnel: w1054 -> [w1088]
                    shift-right: [w1084] -> w1051
                    shift-left: w1052 -> [w1083]
                    tunnel: w1034 -> [w1085]
                    tunnel: w1050 -> [w1082]
                    tunnel: w1049 -> [w1081]
                    tunnel: w1048 -> [w1080]
                    tunnel: w1047 -> [w1076]
                    tunnel: [w1071] -> w1042
                    tunnel: [w1070] -> w1035
                    tunnel: [w1069] -> w1040
                    tunnel: [w1068] -> w1036
                    tunnel: [w1067] -> w1038
                    tunnel: w1033 -> [w1059]
                    stop <- w1077 stop-if-true
                    n380 = call "DegToDAC (SubVI).vi"("R2"=0.0, "Rt"=w1083) -> ("error out"=w1095:errorcluster, "output array"=w1096:u8[])  [unwired: 8 in]
                    n381 = call <vilib>:"High Resolution Relative Seconds.vi"() -> ("relative seconds"=w1075:dbl)
                    n382 = property on="VISA Tester" class="VISAName"() -> ("Value"=w1098:refnum<visa-resource-name>)  [unwired: 2 in, 2 out]
                    n383 = Byte Array To String(unsigned byte array=w1096) -> (string=w1097:string)
                    n384 = Subtract(x=w1076, y=w1075) -> (x-y=w1074:dbl)
                    n385 = VISA Write(VISA resource name=w1098, write buffer=w1097, error in (no error)=w1095) -> (error out=w1094:errorcluster)  [unwired: 2 out]
                    n386 = Greater Or Equal?(x=w1074, y=120.0) -> (x >= y?=w1072:bool)
                    n387 = call <vilib>:"Clear Errors.vi"("error in (no error)"=w1094) -> ("error out"=w1093:errorcluster)  [unwired: 5 in, 1 out]
                    n388 = control-ref of="Ambient Temperature"() -> (w1066:refnum<vi>)
                    n389 = property class="DigNum (strict)"(reference=w1066) -> ("Value"=w1064:dbl)  [unwired: 1 in, 2 out]
                    n390 = property class="Bool (strict)"(reference=w1079) -> ("Value"=w1078:bool)  [unwired: 1 in, 2 out]
                    n391 = Number To Fractional String(number=w1064, precision (6)=i16 2) -> (F-format string=w1061:string)  [unwired: 2 in]
                    n392 = Concatenate Strings(w1065, "\nAmbient  Temp. [C]: " ("string"), w1061) -> (w1060:string)
                    n393 = call "Write panel message (SubVI).vi"("Stop BurnIn"=w1086, 4:"rpm"=w1088, 5:"rpm"=TRUE ("rpm"), "PrintTime"=TRUE, "Stop"=w1079, "error in (no error)"=w1093, "Time to wait"=3.0, "Strin"=w1060, "String in"=w1087) -> ("error out"=w1092:errorcluster)  [unwired: 2 in]
                    n394 = call "TempAlgoTest (SubVI).vi"("Temp"=w1066, "Speed Ind"=w1080, "Motor Speed RPM"=w1088, "Round"=w1085, "Temp Up In"=w1083, "error in (no error)"=w1092, "String in"=w1087, "Temp Goal"=w1082, "Stop"=w1079, "Speed Goal"=w1081, "Stop BurnIn"=w1086, "AD Resistor Step"=w1059, "Strin"=w1060) -> (14:"Speed Pass/Fail"=w1070:bool, "Temp  Pass/Fail"=w1069:dbl, "Temp Up Out"=w1084:dbl, 17:"Speed Pass/Fail"=w1071:dbl, "Temp Pass/Fail"=w1068:bool, "error out"=w1067:errorcluster)  [unwired: 1 in]
                    n395 = Compound Arithmetic op=OR(w1072, w1070, w1078) -> (w1077:bool)
                  }
                  n396 = property class="Bool (strict)"(reference=w1057) -> ("Value"=w1053:bool)  [unwired: 1 in, 2 out]
                  n397 = call "Find_Number_LineMARVIN.vi"("Test Paragraph"=w1039, "error in"=w1038, "TableIn"=w1041) -> ("error out"=w1043:errorcluster, "Line number"=w1046:i32)  [unwired: 2 in, 2 out]
                  n398 = Increment(x=w1046) -> (x+1=w1045:i32)
                  n399 = call "PassOrFail (SubVI).vi"("index (row)"=w1045, "error in (no error)"=w1043, "Data in"=w1040, "Pass?Fail"=w1036, "Table in"=w1041) -> ("error out"=w1044:errorcluster)  [unwired: 6 in]
                  n400 = call "PassOrFail (SubVI).vi"("index (row)"=w1046, "error in (no error)"=w1044, "Data in"=w1042, "Pass?Fail"=w1035, "Table in"=w1041) -> ("error out"=w1037:errorcluster)  [unwired: 6 in]
                }
                n401 = Build Array (concatenate)(w1016, w1015) -> (w1017:bool[])
                n402 = flat-sequence {
                  tunnel: w1019 -> [_]
                  tunnel: [enum16{"Stop", "Algorithm", "Start"}."Stop"] -> w1018
                  frame #0 {
                  }
                }
                n403 = And Array Elements(Boolean array=w1017) -> (logical AND=→"TempControlResult":bool)
              }
              frame "Start" {
                n404 = call <vilib>:"Clear Errors.vi"("error in (no error)"=w1120) -> ("error out"=w1102:errorcluster)  [unwired: 5 in, 1 out]
                n405 = property on="VISA Tester" class="VISAName"() -> ("Value"=w1119:refnum<visa-resource-name>)  [unwired: 2 in, 2 out]
                n406 = call "TesterOption (SubVI).vi"("On/Off 2"=TRUE, "Tester Option 2"=T11."Venable", "2 Options"=TRUE, "error in (no error)"=w1102, "On/Off"=TRUE, "Tester Option"=T11."K16", "VISA Refnum in"=w1119) -> ("error out"=w1101:errorcluster)  [unwired: 3 in, 1 out]
                n407 = call "Time Delay12"("error in (no error)"=w1101) -> ("error out"=w1100:errorcluster)  [unwired: 10 in]
                n408 = call "CANSendMotorSpeed.vi"("Remote"=FALSE, "error in (no error)"=w1100, "Motor Speed RPM"=u16 0, "UUT"=w1105, "CAN Cluster in"=w1106) -> ("error out"=w1107:errorcluster)  [unwired: 6 in]
                n409 = property class="Bool (strict)"(reference=w1113, error in=w1107) -> ("Value"=w1112:bool)  [unwired: 2 out]
                n410 = Select(t=enum16{"Stop", "Algorithm", "Start"}."Stop", s=w1112, f=enum16{"Stop", "Algorithm", "Start"}."Algorithm") -> (s? t:f=w1109:enum16{"Stop", "Algorithm", "Start"})
              }
            }
          }
        }
        frame "Burn in" {
          n411 = control-ref of="Stop Button"() -> (w1124:refnum<vi>)
          n412 = control-ref of="Pannel User Message"() -> (w1127:refnum<vi>)
          n413 = control-ref of="ATR"() -> (w1123:refnum<vi>)
          n414 = control-ref of="Config_CANAT"() -> (w1126:refnum<vi>)
          n415 = control-ref of="UUT"() -> (w1125:refnum<vi>)
          n416 = control-ref of="Stop Burn-in"() -> (w1122:refnum<vi>)
          n417 = property on="UUT" class="DigNum (strict)"() -> ("Value"=w1121:u8)  [unwired: 2 in, 2 out]
          n418 = while {
            tunnel: w1127 -> [w1138]
            tunnel: w1123 -> [w1137]
            tunnel: w1126 -> [w1136]
            tunnel: w1125 -> [w1135]
            tunnel: w1124 -> [w1134]
            shift-right: [w1133] -> _
            shift-left: T15."Start" -> [w1140]
            shift-right: [w1139] -> _
            shift-left: _ -> [w1131]
            tunnel: w1122 -> [w1130]
            tunnel: w1121 -> [w1129]
            stop <- w1132 stop-if-true
            n419 = case shown="\"BurnIn\"" w1140 {
              tunnel: [w1143 w1178 w1246 w1275 w1308 w1344] -> w1139
              tunnel: w1138 -> [_ w1170 _ _ _ w1343]
              tunnel: w1137 -> [_ w1173 w1219 w1262 w1294 w1330]
              tunnel: w1136 -> [_ w1169 _ _ _ w1342]
              tunnel: w1135 -> [_ w1166 _ _ _ w1321]
              tunnel: w1134 -> [_ _ w1248 w1277 w1312 w1336]
              tunnel: [w1141 T15."Stop" w1249 w1278 w1313 w1332] -> w1133
              tunnel: [w1142 FALSE FALSE FALSE FALSE FALSE] -> w1132
              tunnel: w1131 -> [w1143 w1178 w1246 w1275 w1308 _]
              tunnel: w1130 -> [_ _ _ _ _ w1326]
              tunnel: w1129 -> [_ w1158 w1210 w1254 w1286 w1320]
              frame "Stop", Default {
                n420 = flat-sequence {
                  tunnel: [TRUE] -> w1142
                  tunnel: [T15."Stop"] -> w1141
                  frame #0 {
                    n421 = property on="VISA Tester" class="VISAName"() -> ("Value"=w1148:refnum<visa-resource-name>)  [unwired: 2 in, 2 out]
                    n422 = call "TesterOption (SubVI).vi"("2 Options"=FALSE, "On/Off"=FALSE, "Tester Option"=T11."Venable", "VISA Refnum in"=w1148) -> ("error out"=w1145:errorcluster)  [unwired: 6 in, 1 out]
                    n423 = property on="Stop Burn-in" class="Bool (strict)"(error in=w1145, "Visible"=FALSE) -> ()  [unwired: 1 in, 2 out]
                  }
                  frame #1 {
                  }
                }
              }
              frame "BurnIn" {
                w1162 = FALSE ("Stop Burn-in")
                n424 = control-ref of="Motor Speed RPM"() -> (w1172:refnum<vi>)
                n425 = control-ref of="Stop Button"() -> (w1171:refnum<vi>)
                n426 = property on="Stop Burn-in" class="Bool (strict)"("Visible"=TRUE) -> (error out=w1174:errorcluster)  [unwired: 2 in, 1 out]
                n427 = Equal?(x=w1158, y=u8 95) -> (x = y?=w1155:bool)
                n428 = Select(t="8. " ("Test Paragraph"), s=w1155, f="7. " ("Test Paragraph")) -> (s? t:f=w1154:string)
                n429 = Select(t="8.4" ("Test Paragraph"), s=w1155, f="7.4" ("Test Paragraph")) -> (s? t:f=w1159:string)
                n430 = call "Find_Number_LineMARVIN.vi"("Test Paragraph"=w1159, "error in"=w1174, "TableIn"=w1173) -> ("error out"=w1176:errorcluster, "Line number"=w1177:i32)  [unwired: 2 in, 2 out]
                n431 = Select(t=u16 15100, s=w1155, f=u16 12100 ("y")) -> (s? t:f=w1164:u16)
                n432 = for {
                  tunnel: w1176 -> [w1198]
                  tunnel: dbl[] [600.0, 600.0, 600.0] -> [w1202] mode=indexing
                  tunnel: w1177 -> [w1207]
                  tunnel: w1173 -> [w1197]
                  tunnel: w1172 -> [w1196]
                  tunnel: w1171 -> [w1195]
                  tunnel: w1170 -> [w1194]
                  tunnel: w1169 -> [w1190]
                  tunnel: w1166 -> [w1189]
                  tunnel: w1164 -> [w1188]
                  tunnel: [w1186] -> w1163
                  tunnel: w1154 -> [w1183]
                  tunnel: [w1182] -> w1153 mode=indexing
                  i -> [w1204]
                  n433 = call "CANSendMotorSpeed.vi"("Remote"=TRUE, "error in (no error)"=w1198, "Motor Speed RPM"=w1188, "UUT"=w1189, "CAN Cluster in"=w1190) -> ("error out"=w1192:errorcluster)  [unwired: 6 in]
                  n434 = control-ref of="Stop Burn-in"() -> (w1193:refnum<vi>)
                  n435 = Concatenate Strings(w1183, "Burn-in test in process..." ("Strin")) -> (w1184:string)
                  n436 = Add(x=w1207, y=w1204) -> (x+y=w1203:i32)
                  n437 = call "Write panel message (SubVI).vi"("Stop BurnIn"=w1193, 4:"rpm"=w1196, 5:"rpm"=TRUE ("rpm"), "PrintTime"=TRUE, "Stop"=w1195, "error in (no error)"=w1192, "Time to wait"=w1202, "Strin"=w1184, "String in"=w1194) -> ("error out"=w1199:errorcluster)  [unwired: 2 in]
                  n438 = control-ref of="Power transistor Heat sink Temp."() -> (w1208:refnum<vi>)
                  n439 = property on="MaxBurnInTempVal" class="DigNum (strict)"() -> ("Value"=w1206:dbl)  [unwired: 2 in, 2 out]
                  n440 = property class="DigNum (strict)"(reference=w1208, error in=w1199) -> (error out=w1187:errorcluster, "Value"=w1205:dbl)  [unwired: 1 out]
                  n441 = Less Or Equal?(x=w1205, y=w1206) -> (x <= y?=w1182:bool)
                  n442 = call "PassOrFail (SubVI).vi"("index (row)"=w1203, "error in (no error)"=w1187, "Data in"=w1205, "Pass?Fail"=w1182, "Table in"=w1197) -> ("error out"=w1186:errorcluster)  [unwired: 6 in]
                }
                n443 = And Array Elements(Boolean array=w1153) -> (logical AND=→"BurnResult":bool)
                n444 = property on="Stop Burn-in" class="Bool (strict)"(error in=w1163, "Value"=w1162, "Visible"=w1162) -> ()  [unwired: 1 in, 2 out]
              }
              frame "Ambient Temp" {
                w1224 = 2 ("disabled index (col)")
                n445 = control-ref of="Power transistor Heat sink Temp."() -> (w1234:refnum<vi>)
                n446 = Equal?(x=w1210, y=u8 95) -> (x = y?=w1213:bool)
                n447 = Select(t="8.3" ("Test Paragraph"), s=w1213, f="7.3" ("Test Paragraph")) -> (s? t:f=w1211:string)
                n448 = call "Find_Number_LineMARVIN.vi"("Test Paragraph"=w1211, "TableIn"=w1219) -> ("error out"=w1245:errorcluster, "Line number"=w1225:i32)  [unwired: 3 in, 2 out]
                n449 = property class="DigNum (strict)"(reference=w1234, error in=w1245) -> (error out=w1236:errorcluster, "Value"=w1226:dbl)  [unwired: 1 out]
                n450 = Select(t=25.0 ("y"), s=w1213, f=25.0 ("y")) -> (s? t:f=w1235:dbl)
                n451 = Select(t=13.0 ("y"), s=w1213, f=13.0) -> (s? t:f=w1237:dbl)
                n452 = Add(x=w1235, y=w1237) -> (x+y=w1244:dbl)
                n453 = Subtract(x=w1235, y=w1237) -> (x-y=w1243:dbl)
                n454 = In Range and Coerce(upper limit=w1244, x=w1226, lower limit=w1243) -> (In Range?=w1209:bool)  [unwired: 1 out]
                "BurnTemp" <- w1209
                n455 = call "PassOrFail (SubVI).vi"("index (row)"=w1225, "error in (no error)"=w1236, "Data in"=w1226, "Pass?Fail"=w1209, "Table in"=w1219) -> ("error out"=w1216:errorcluster)  [unwired: 6 in]
                n456 = property class="Tbl (strict)"(reference=w1219, error in=w1216) -> (reference out=w1218:refnum<vi>, error out=w1233:errorcluster, "Value"=w1232:string[][])
                n457 = Add(x=w1226, y=25.0) -> (x+y=w1217:dbl)
                "MaxBurnInTempVal" <- w1217
                n458 = Number To Fractional String(number=w1217, precision (6)=i16 0) -> (F-format string=w1231:string)  [unwired: 2 in]
                n459 = Concatenate Strings("< " ("string"), w1231) -> (w1220:string)
                n460 = Increment(x=w1225) -> (x+1=w1223:i32)
                n461 = Increment(x=w1223) -> (x+1=w1222:i32)
                n462 = Increment(x=w1222) -> (x+1=w1221:i32)
                n463 = Replace Array Subset(array=w1232, new element #1=w1220, index (row) #1=w1223, index (col) #1=w1224, new element #2=w1220, index (row) #2=w1222, index (col) #2=w1224, new element #3=w1220, index (row) #3=w1221, index (col) #3=w1224) -> (w1230:string[][])
                n464 = property class="Tbl (strict)"(reference=w1218, error in=w1233, "Value"=w1230) -> (error out=w1215:errorcluster)  [unwired: 1 out]
                n465 = property class="Bool (strict)"(reference=w1248, error in=w1215) -> ("Value"=w1252:bool)  [unwired: 2 out]
                n466 = Select(t=T15."Stop", s=w1252, f=T15."BurnIn") -> (s? t:f=w1249:T15)
              }
              frame "MotorSpeed" {
                n467 = control-ref of="Motor Speed RPM"() -> (w1260:refnum<vi>)
                n468 = Equal?(x=w1254, y=u8 95) -> (x = y?=w1257:bool)
                n469 = Select(t="8.2" ("Test Paragraph"), s=w1257, f="7.2" ("Test Paragraph")) -> (s? t:f=w1255:string)
                n470 = call "Find_Number_LineMARVIN.vi"("Test Paragraph"=w1255, "TableIn"=w1262) -> ("error out"=w1274:errorcluster, "Line number"=w1265:i32)  [unwired: 3 in, 2 out]
                n471 = property class="DigNum (strict)"(reference=w1260, error in=w1274) -> (error out=w1263:errorcluster, "Value"=w1264:dbl)  [unwired: 1 out]
                n472 = Select(t=15100.0 ("y"), s=w1257, f=12100.0 ("y")) -> (s? t:f=w1261:dbl)
                n473 = Select(t=200.0 ("y"), s=w1257, f=200.0) -> (s? t:f=w1266:dbl)
                n474 = Add(x=w1261, y=w1266) -> (x+y=w1273:dbl)
                n475 = Subtract(x=w1261, y=w1266) -> (x-y=w1272:dbl)
                n476 = In Range and Coerce(upper limit=w1273, x=w1264, lower limit=w1272) -> (In Range?=w1253:bool)  [unwired: 1 out]
                "BurnSpeed" <- w1253
                n477 = call "PassOrFail (SubVI).vi"("index (row)"=w1265, "error in (no error)"=w1263, "Data in"=w1264, "Pass?Fail"=w1253, "Table in"=w1262) -> ("error out"=w1259:errorcluster)  [unwired: 6 in]
                n478 = property class="Bool (strict)"(reference=w1277, error in=w1259) -> ("Value"=w1281:bool)  [unwired: 2 out]
                n479 = Select(t=T15."Stop", s=w1281, f=T15."Ambient Temp") -> (s? t:f=w1278:T15)
              }
              frame "DC Current Measure" {
                n480 = property on="VISA Tester" class="VISAName"() -> (error out=w1306:errorcluster, "Value"=w1310:refnum<visa-resource-name>)  [unwired: 2 in, 1 out]
                n481 = call "GetADCTester (SubVI).vi"("error in (no error)"=w1306, "GetADCTester"=T13."Current", "TimeToGet"=10, "VISA Refnum in"=w1310) -> ("error out"=w1307:errorcluster, "ADCValOutput Single"=w1293:dbl)  [unwired: 5 in, 1 out]
                n482 = Equal?(x=w1286, y=u8 95) -> (x = y?=w1290:bool)
                n483 = Select(t="8.1" ("Test Paragraph"), s=w1290, f="7.1" ("Test Paragraph")) -> (s? t:f=w1288:string)
                n484 = call "Find_Number_LineMARVIN.vi"("Test Paragraph"=w1288, "error in"=w1307, "TableIn"=w1294) -> ("error out"=w1305:errorcluster, "Line number"=w1295:i32)  [unwired: 2 in, 2 out]
                n485 = Select(t=50.0 ("y"), s=w1290, f=28.0 ("y")) -> (s? t:f=w1297:dbl)
                n486 = Select(t=5.0 ("y"), s=w1290, f=3.0) -> (s? t:f=w1296:dbl)
                n487 = Add(x=w1297, y=w1296) -> (x+y=w1304:dbl)
                n488 = Subtract(x=w1297, y=w1296) -> (x-y=w1303:dbl)
                n489 = In Range and Coerce(upper limit=w1304, x=w1293, lower limit=w1303) -> (In Range?=w1284:bool)  [unwired: 1 out]
                "BurnDC" <- w1284
                n490 = call "PassOrFail (SubVI).vi"("index (row)"=w1295, "error in (no error)"=w1305, "Data in"=w1293, "Pass?Fail"=w1284, "Table in"=w1294) -> ("error out"=w1292:errorcluster)  [unwired: 6 in]
                n491 = property class="Bool (strict)"(reference=w1312, error in=w1292) -> ("Value"=w1283:bool)  [unwired: 2 out]
                n492 = Not(x=w1284) -> (.not. x?=w1282:bool)
                n493 = Or(x=w1282, y=w1283) -> (x .or. y?=w1285:bool)
                n494 = Select(t=T15."Stop", s=w1285, f=T15."MotorSpeed") -> (s? t:f=w1313:T15)
              }
              frame "Start" {
                n495 = Equal?(x=w1320, y=u8 95) -> (x = y?=w1322:bool)
                n496 = Select(t="8" ("Test Paragraph"), s=w1322, f="7" ("Test Paragraph")) -> (s? t:f=w1317:string)
                n497 = Concatenate Strings(w1317, ". Burn-in test in process...\nFull Speed Operation" ("Value")) -> (w1316:string)
                n498 = property class="Str"(reference=w1343, "Value"=w1316) -> (reference out=w1340:refnum<vi>, error out=w1325:errorcluster)  [unwired: 1 in]
                n499 = call "Find_Number_LineMARVIN.vi"("Test Paragraph"=w1317, "error in"=w1325, "TableIn"=w1330) -> ("error out"=w1350:errorcluster, "Line number"=w1351:i32)  [unwired: 2 in, 2 out]
                n500 = Select(t=u16 15100 ("y"), s=w1322, f=u16 12100 ("y")) -> (s? t:f=w1357:u16)
                n501 = call "Table_ScrollaBarMarvin.vi"("error in"=w1350, "Line to focus"=w1317, "reference in"=w1330) -> ("error out"=w1352:errorcluster)  [unwired: 2 out]
                n502 = call "Reset old test Values (SubVI).vi"("error in"=w1352, "Atr in"=w1330, "Test Paragraph"=w1317) -> ("error out"=w1353:errorcluster)  [unwired: 8 in]
                n503 = Increment(x=w1351) -> (x+1=w1344:i32)
                n504 = property on="VISA Tester" class="VISAName"(error in=w1353) -> (error out=w1354:errorcluster, "Value"=w1355:refnum<visa-resource-name>)  [unwired: 1 in, 1 out]
                n505 = call "TesterOption (SubVI).vi"("2 Options"=FALSE, "error in (no error)"=w1354, "On/Off"=TRUE, "Tester Option"=T11."Venable", "VISA Refnum in"=w1355) -> ("error out"=w1356:errorcluster)  [unwired: 5 in, 1 out]
                n506 = call "CANSendMotorSpeed.vi"("Remote"=TRUE, "error in (no error)"=w1356, "Motor Speed RPM"=w1357, "UUT"=w1321, "CAN Cluster in"=w1342) -> ("error out"=w1341:errorcluster)  [unwired: 6 in]
                n507 = control-ref of="Motor Speed RPM"() -> (w1329:refnum<vi>)
                n508 = call "Write panel message (SubVI).vi"("Stop BurnIn"=w1326, 4:"rpm"=w1329, 5:"rpm"=TRUE ("rpm"), "PrintTime"=TRUE, "Stop"=w1336, "error in (no error)"=w1341, "Time to wait"=50.0, "Strin"=w1316, "String in"=w1340) -> ("error out"=w1328:errorcluster)  [unwired: 2 in]
                n509 = property class="Bool (strict)"(reference=w1336, error in=w1328) -> ("Value"=w1335:bool)  [unwired: 2 out]
                n510 = Select(t=T15."Stop", s=w1335, f=T15."DC Current Measure") -> (s? t:f=w1332:T15)
              }
            }
          }
        }
        frame "Visual Inspec" {
          n511 = property on="VISA Tester" class="VISAName"() -> ("Value"=w1368:refnum<visa-resource-name>)  [unwired: 2 in, 2 out]
          n512 = call "TesterOption (SubVI).vi"("2 Options"=FALSE, "error in (no error)"=w1369, "On/Off"=FALSE, "Tester Option"=T11."Venable", "VISA Refnum in"=w1368) -> ("error out"=w1364:errorcluster)  [unwired: 5 in, 1 out]
          n513 = local read "UUT"() -> (w1360:u8)
          n514 = Equal?(x=w1360, y=u8 95) -> (x = y?=w1361:bool)
          n515 = case shown="True" w1361 {
            tunnel: w1370 -> [w1374 w1378]
            tunnel: w1364 -> [w1373 w1377]
            tunnel: [w1371 w1376] -> w1363
            tunnel: [w1372 w1375] -> w1359
            frame False {
              # "AHU"
              n516 = call "VisualInspectionAHU.vi"("error in (no error)"=w1373, "TableRef"=w1374) -> ("error out"=w1372:errorcluster, "VisualInspectionResult"=w1371:bool)  [unwired: 8 in]
            }
            frame True {
              # "EBAY"
              n517 = call "VisualInspectionEBAY.vi"("error in (no error)"=w1377, "TableRef"=w1378) -> ("error out"=w1375:errorcluster, "VisualInspectionResult"=w1376:bool)  [unwired: 8 in]
            }
          }
          "VisualInspectionResult" <- w1363
          n518 = property on="Automation" class="Bool (strict)"(error in=w1359) -> ("Value"=w1358:bool)  [unwired: 1 in, 2 out]
          n519 = case shown="True" w1358 {
            frame False {
            }
            frame True {
              w1379 = TRUE ("Value (Signaling)")
              n520 = property on="SetSN" class="Bool (strict)"("Val(Sgnl)"=w1379, "Value"=w1379) -> ()  [unwired: 2 in, 2 out]
            }
          }
        }
        frame "Temp Sens Cal" {
          w1383 = "2. Temperature sensor calibration test in process..." ("Value")
          w1381 = "2" ("Test Paragraph")
          n521 = control-ref of="Pannel User Message"() -> (w1390:refnum<vi>)
          n522 = property class="Str"(reference=w1390, error in=w1389, "Value"=w1383) -> (error out=w1388:errorcluster)  [unwired: 1 out]
          n523 = call "Table_ScrollaBarMarvin.vi"("error in"=w1388, "Line to focus"=w1381, "reference in"=w1391) -> ("error out"=w1393:errorcluster)  [unwired: 2 out]
          n524 = property class="Tbl (strict)"(reference=w1391, error in=w1393) -> (reference out=w1380:refnum<vi>, error out=w1395:errorcluster, "Value"=w1396:string[][])
          n525 = Index Array(array=w1396, index (col)=0 ("disabled index (col)")) -> (element=w1397:string[])  [unwired: 1 in]
          n526 = call "Find_Number_Line.vi"("error in"=w1395, "Test Paragraph"=w1381, "Row Headers[]"=w1397) -> ("error out"=w1392:errorcluster, "Line number"=w1385:i32)  [unwired: 1 out]
          n527 = property on="Status" class="Bool (strict)"(error in=w1392) -> (error out=w1386:errorcluster, "Value"=w1387:bool)  [unwired: 1 in, 1 out]
          n528 = call "Reset old test Values (SubVI).vi"("error in"=w1386, "Atr in"=w1380, "Test Paragraph"=w1381) -> ("error out"=w1382:errorcluster)  [unwired: 8 in]
          n529 = case shown="True" w1387 {
            selector: w1387 -> [w1401 _]
            tunnel: w1382 -> [w1403 _]
            tunnel: w1380 -> [w1400 _]
            tunnel: w1385 -> [w1399 _]
            tunnel: w1384 -> [_ w1410]
            tunnel: w1383 -> [_ w1406]
            frame False {
              n530 = flat-sequence {
                tunnel: w1403 -> [w1404]
                tunnel: [w1404] -> w1402
                frame #0 {
                  n531 = One Button Dialog(message="Please establish RS connection.") -> ()  [unwired: 1 in, 1 out]
                }
              }
              n532 = Increment(x=w1399) -> (x+1=w1398:i32)
              n533 = call "PassOrFail (SubVI).vi"("index (row)"=w1398, "error in (no error)"=w1402, "Pass?Fail"=w1401, "Table in"=w1400) -> ()  [unwired: 7 in, 1 out]
            }
            frame True {
              n534 = control-ref of="Stop Burn-in"() -> (w1412:refnum<vi>)
              n535 = control-ref of="Pannel User Message"() -> (w1414:refnum<vi>)
              n536 = control-ref of="Config_CANAT"() -> (w1408:refnum<vi>)
              n537 = control-ref of="ATR"() -> (w1415:refnum<vi>)
              n538 = control-ref of="Motor Speed RPM"() -> (w1416:refnum<vi>)
              n539 = control-ref of="UUT"() -> (w1407:refnum<vi>)
              n540 = control-ref of="Stop Button"() -> (w1413:refnum<vi>)
              n541 = property on="VISA Tester" class="VISAName"() -> ("Value"=w1409:refnum<visa-resource-name>)  [unwired: 2 in, 2 out]
              n542 = while {
                shift-right: [w1419] -> _
                shift-left: T14."Start" -> [w1429]
                tunnel: w1412 -> [w1428]
                tunnel: w1413 -> [w1427]
                tunnel: w1414 -> [w1426]
                tunnel: w1415 -> [w1425]
                tunnel: w1416 -> [w1424]
                tunnel: w1410 -> [w1423]
                tunnel: w1409 -> [w1422]
                tunnel: w1408 -> [w1421]
                tunnel: w1407 -> [w1420]
                tunnel: w1406 -> [w1417]
                stop <- w1418 stop-if-true
                n543 = case shown="\"Start\"" w1429 {
                  tunnel: w1428 -> [_ w1464 w1491 w1546 w1576]
                  tunnel: w1427 -> [_ w1465 w1483 w1532 w1578]
                  tunnel: w1426 -> [_ w1462 w1492 w1544 w1580]
                  tunnel: w1425 -> [_ w1442 _ _ _]
                  tunnel: w1424 -> [_ w1466 w1490 w1547 w1575]
                  tunnel: w1423 -> [_ w1475 w1495 w1556 w1572]
                  tunnel: w1422 -> [w1432 w1471 w1494 w1552 w1560]
                  tunnel: w1421 -> [_ _ _ _ w1586]
                  tunnel: w1420 -> [_ _ _ _ w1585]
                  tunnel: [w1430 w1451 w1484 w1535 w1563] -> w1419
                  tunnel: [w1431 FALSE FALSE FALSE FALSE] -> w1418
                  tunnel: w1417 -> [_ _ w1493 _ _]
                  frame "Stop", Default {
                    n544 = flat-sequence {
                      tunnel: w1432 -> [w1433]
                      tunnel: [TRUE] -> w1431
                      tunnel: [T14."Stop"] -> w1430
                      frame #0 {
                        n545 = call "TesterOption (SubVI).vi"("2 Options"=FALSE, "On/Off"=FALSE, "Tester Option"=T11."Venable", "VISA Refnum in"=w1433) -> ()  [unwired: 6 in, 2 out]
                      }
                      frame #1 {
                      }
                    }
                  }
                  frame "AO[1]=Meas." {
                    n546 = property on="AO[1]Meas" class="DigNum (strict)"() -> ("Value"=w1445:dbl)  [unwired: 2 in, 2 out]
                    n547 = Number To Fractional String(number=w1445) -> (F-format string=w1453:string)  [unwired: 3 in]
                    n548 = Search and Replace String(input string="EP=1\r\nAO[1]=0\r\n" ("write buffer"), search string="0", replace string=w1453) -> (result string=w1452:string)  [unwired: 5 in, 3 out]
                    n549 = call "SerialMarvinSendGet.vi"("Clear Log"=FALSE, "write buffer"=w1452, "VISA resource name"=w1475) -> ("error out"=w1470:errorcluster)  [unwired: 7 in, 1 out]
                    n550 = call "TesterOption (SubVI).vi"("2 Options"=FALSE, "error in (no error)"=w1470, "On/Off"=FALSE, "Tester Option"=T11."Power", "VISA Refnum in"=w1471) -> ("error out"=w1469:errorcluster, "VISA Refnum out"=w1456:refnum<visa-resource-name>)  [unwired: 5 in]
                    n551 = call "Write panel message (SubVI).vi"("Stop BurnIn"=w1464, 4:"rpm"=w1466, 5:"rpm"=FALSE ("rpm"), "PrintTime"=TRUE, "Stop"=w1465, "error in (no error)"=w1469, "Time to wait"=20.0, "Strin"="2. Temperature sensor calibration test in process...\nSet Parameters...", "String in"=w1462) -> ("error out"=w1457:errorcluster)  [unwired: 2 in]
                    n552 = call "TesterOption (SubVI).vi"("2 Options"=FALSE, "error in (no error)"=w1457, "On/Off"=FALSE, "Tester Option"=T11."Venable", "VISA Refnum in"=w1456) -> ("error out"=w1450:errorcluster)  [unwired: 5 in, 1 out]
                    n553 = flat-sequence {
                      tunnel: [T14."Stop"] -> w1451
                      tunnel: w1443 -> [_]
                      frame #0 {
                      }
                    }
                    n554 = In Range and Coerce(upper limit=0.1, x=w1445, lower limit=-0.1) -> (In Range?=w1440:bool)  [unwired: 1 out]
                    "SensCalResult" <- w1440
                    n555 = call "Find_Number_LineMARVIN.vi"("Test Paragraph"="2.1", "error in"=w1450, "TableIn"=w1442) -> ("error out"=w1444:errorcluster, "Line number"=w1448:i32)  [unwired: 2 in, 2 out]
                    n556 = call "PassOrFail (SubVI).vi"("Test#"="2", "index (row)"=w1448, "error in (no error)"=w1444, "Data in"=w1445, "Pass?Fail"=w1440, "Table in"=w1442) -> ("error out"=w1443:errorcluster)  [unwired: 5 in]
                  }
                  frame "TA[5]" {
                    w1496 = T17 [enum."50C", enum."80C", enum."100C", enum."120C"] items=["K15", "K16", "K17", "Venable", "Firmeware", "Fan", "Power", "120C", "110C", "100C", "90C", "80C", "70C", "60C", "50C", "40C", "30C", "25C", "20C", "10C", "0C"]
                    n557 = for {
                      tunnel: w1496 -> [w1511] mode=indexing
                      tunnel: w1495 -> [w1510]
                      tunnel: w1494 -> [w1509]
                      tunnel: w1493 -> [w1508]
                      tunnel: w1492 -> [w1507]
                      tunnel: w1483 -> [w1506]
                      tunnel: w1491 -> [w1505]
                      tunnel: w1490 -> [w1504]
                      tunnel: dbl[] [0.59774, 0.65238, 0.68545, 0.71584] -> [w1499] mode=indexing
                      tunnel: [w1498] -> w1479 mode=indexing
                      tunnel: [w1497] -> w1482
                      n558 = for {
                        N: 5 -> [_]
                        tunnel: w1511 -> [w1529]
                        tunnel: w1510 -> [w1528]
                        tunnel: w1509 -> [w1524]
                        tunnel: w1508 -> [w1522]
                        tunnel: w1507 -> [w1521]
                        tunnel: w1506 -> [w1520]
                        tunnel: w1505 -> [w1518]
                        tunnel: w1504 -> [w1515]
                        tunnel: [w1514] -> w1503 mode=indexing
                        tunnel: [w1513] -> w1497
                        n559 = call "TesterOption (SubVI).vi"("2 Options"=FALSE, "On/Off"=TRUE, "Tester Option"=w1529, "VISA Refnum in"=w1524) -> ("error out"=w1525:errorcluster)  [unwired: 6 in, 1 out]
                        n560 = call "Write panel message (SubVI).vi"("Stop BurnIn"=w1518, 4:"rpm"=w1515, 5:"rpm"=FALSE ("rpm"), "PrintTime"=FALSE, "Stop"=w1520, "error in (no error)"=w1525, "Time to wait"=1.0, "Strin"=w1522, "String in"=w1521) -> ("error out"=w1523:errorcluster)  [unwired: 2 in]
                        n561 = call "SerialMarvinSendGet.vi"("error in (no error)"=w1523, "write buffer"="TA[5]\r\n", "VISA resource name"=w1528) -> ("error out"=w1513:errorcluster, "read buffer"=w1526:string)  [unwired: 7 in]
                        n562 = Fract/Exp String To Number(string=w1526) -> (number=w1514:dbl)  [unwired: 3 in, 1 out]
                      }
                      n563 = Add Array Elements(numeric array=w1503) -> (sum=w1502:dbl)
                      n564 = Divide(x=w1502, y=5.0) -> (x/y=w1500:dbl)
                      n565 = Subtract(x=w1500, y=w1499) -> (x-y=w1498:dbl)
                    }
                    n566 = property class="Bool (strict)"(reference=w1483, error in=w1482) -> ("Value"=w1488:bool)  [unwired: 2 out]
                    n567 = Select(t=T14."Stop", s=w1488, f=T14."AO[1]=Meas.") -> (s? t:f=w1484:T14)
                    n568 = Array Size(array=w1479) -> (size(s)=w1478:i32)
                    n569 = Add Array Elements(numeric array=w1479) -> (sum=w1481:dbl)
                    n570 = Divide(x=w1481, y=w1478) -> (x/y=→"AO[1]Meas":dbl)
                  }
                  frame "AO[1]=0" {
                    n571 = call "SerialMarvinSendGet.vi"("write buffer"="EP=1\r\nAO[1]=0\r\n", "VISA resource name"=w1556) -> ("error out"=w1551:errorcluster)  [unwired: 8 in, 1 out]
                    n572 = call "TesterOption (SubVI).vi"("2 Options"=FALSE, "error in (no error)"=w1551, "On/Off"=FALSE, "Tester Option"=T11."Power", "VISA Refnum in"=w1552) -> ("error out"=w1550:errorcluster, "VISA Refnum out"=w1538:refnum<visa-resource-name>)  [unwired: 5 in]
                    n573 = call "Write panel message (SubVI).vi"("Stop BurnIn"=w1546, 4:"rpm"=w1547, 5:"rpm"=FALSE ("rpm"), "PrintTime"=TRUE, "Stop"=w1532, "error in (no error)"=w1550, "Time to wait"=20.0, "Strin"="2. Temperature sensor calibration test in process...\nSet Parameters...", "String in"=w1544) -> ("error out"=w1539:errorcluster)  [unwired: 2 in]
                    n574 = call "TesterOption (SubVI).vi"("2 Options"=FALSE, "error in (no error)"=w1539, "On/Off"=FALSE, "Tester Option"=T11."Venable", "VISA Refnum in"=w1538) -> ("error out"=w1533:errorcluster)  [unwired: 5 in, 1 out]
                    n575 = property class="Bool (strict)"(reference=w1532, error in=w1533) -> ("Value"=w1537:bool)  [unwired: 2 out]
                    n576 = Select(t=T14."Stop", s=w1537, f=T14."TA[5]") -> (s? t:f=w1535:T14)
                  }
                  frame "Start" {
                    n577 = call "Write panel message (SubVI).vi"("Stop BurnIn"=w1576, 4:"rpm"=w1575, 5:"rpm"=FALSE ("rpm"), "PrintTime"=FALSE, "Stop"=w1578, "Time to wait"=0.1, "Strin"="2. Temperature sensor calibration test in process...\nInitialization state...", "String in"=w1580) -> ("error out"=w1581:errorcluster)  [unwired: 3 in]
                    n578 = call "TesterOption (SubVI).vi"("2 Options"=FALSE, "error in (no error)"=w1581, "On/Off"=FALSE, "Tester Option"=T11."Venable", "VISA Refnum in"=w1560) -> ("error out"=w1583:errorcluster)  [unwired: 5 in, 1 out]
                    n579 = call "CANSendMotorSpeed.vi"("Remote"=TRUE, "error in (no error)"=w1583, "Motor Speed RPM"=u16 0, "UUT"=w1585, "CAN Cluster in"=w1586) -> ("error out"=w1570:errorcluster)  [unwired: 6 in]
                    n580 = call "SerialMarvinSendGet.vi"("error in (no error)"=w1570, "write buffer"="AO[1]\r\n", "VISA resource name"=w1572) -> ("error out"=w1559:errorcluster, "read buffer"=w1569:string)  [unwired: 7 in]
                    n581 = Equal?(x=w1569, y="0.0") -> (x = y?=w1561:bool)
                    n582 = property class="Bool (strict)"(reference=w1578, error in=w1559) -> ("Value"=w1590:bool)  [unwired: 2 out]
                    n583 = Select(t=T14."TA[5]", s=w1561, f=T14."AO[1]=0") -> (s? t:f=w1565:T14)
                    n584 = Select(t=T14."Stop", s=w1590, f=w1565) -> (s? t:f=w1563:T14)
                  }
                }
              }
            }
          }
        }
        frame "Auxiliary" {
          w1594 = "9. Auxiliary test in process..." ("Value")
          w1606 = "9" ("Test Paragraph")
          n585 = control-ref of="Pannel User Message"() -> (w1605:refnum<vi>)
          n586 = property class="Str"(reference=w1605, error in=w1602, "Value"=w1594) -> (error out=w1604:errorcluster)  [unwired: 1 out]
          n587 = call "Table_ScrollaBarMarvin.vi"("error in"=w1604, "Line to focus"=w1606, "reference in"=w1603) -> ("error out"=w1612:errorcluster)  [unwired: 2 out]
          n588 = property class="Tbl (strict)"(reference=w1603, error in=w1612) -> (reference out=w1601:refnum<vi>, error out=w1611:errorcluster, "Value"=w1610:string[][])
          n589 = Index Array(array=w1610, index (col)=0 ("disabled index (col)")) -> (element=w1609:string[])  [unwired: 1 in]
          n590 = call "Find_Number_Line.vi"("error in"=w1611, "Test Paragraph"=w1606, "Row Headers[]"=w1609) -> ("error out"=w1607:errorcluster, "Line number"=w1592:i32)  [unwired: 1 out]
          n591 = call "Reset old test Values (SubVI).vi"("error in"=w1607, "Atr in"=w1601, "Test Paragraph"=w1606) -> ("error out"=w1599:errorcluster)  [unwired: 8 in]
          n592 = property on="VISA Tester" class="VISAName"() -> ("Value"=w1593:refnum<visa-resource-name>)  [unwired: 2 in, 2 out]
          n593 = control-ref of="Stop Burn-in"() -> (w1596:refnum<vi>)
          n594 = control-ref of="Stop Button"() -> (w1597:refnum<vi>)
          n595 = control-ref of="Pannel User Message"() -> (w1598:refnum<vi>)
          n596 = control-ref of="ATR"() -> (w1591:refnum<vi>)
          n597 = control-ref of="Config_CANAT"() -> ()  [unwired: 1 out]
          n598 = control-ref of="Motor Speed RPM"() -> (w1595:refnum<vi>)
          n599 = while {
            shift-right: [w1617] -> _
            shift-left: enum16{"Stop", "CoolingON", "HotGunON", "Start"}."Start" -> [w1624]
            tunnel: w1599 -> [w1615]
            tunnel: w1598 -> [w1623]
            tunnel: w1597 -> [w1622]
            tunnel: w1596 -> [w1621]
            tunnel: w1595 -> [w1620]
            tunnel: w1594 -> [w1619]
            tunnel: w1593 -> [w1618]
            tunnel: w1592 -> [w1614]
            tunnel: w1591 -> [w1613]
            stop <- w1616 stop-if-true
            n600 = case shown="\"CoolingON\"" w1624 {
              tunnel: w1623 -> [_ w1669 w1764 w1824]
              tunnel: w1622 -> [_ w1664 w1759 w1810]
              tunnel: w1621 -> [_ w1668 w1763 w1823]
              tunnel: w1620 -> [_ w1667 w1762 w1819]
              tunnel: w1619 -> [_ w1658 w1753 w1818]
              tunnel: w1618 -> [_ w1659 w1754 w1811]
              tunnel: [w1626 w1661 w1756 w1806] -> w1617
              tunnel: [w1625 FALSE FALSE FALSE] -> w1616
              tunnel: w1615 -> [_ w1657 w1752 _]
              tunnel: w1614 -> [_ w1652 w1747 _]
              tunnel: w1613 -> [_ w1648 w1744 _]
              frame "Stop", Default {
                n601 = flat-sequence {
                  tunnel: [enum16{"Stop", "CoolingON", "HotGunON", "Start"}."Stop"] -> w1626
                  tunnel: [TRUE] -> w1625
                  frame #0 {
                    n602 = property on="VISA Tester" class="VISAName"() -> ("Value"=w1630:refnum<visa-resource-name>)  [unwired: 2 in, 2 out]
                    n603 = call "TesterOption (SubVI).vi"("2 Options"=FALSE, "On/Off"=FALSE, "Tester Option"=T11."Venable", "VISA Refnum in"=w1630) -> ()  [unwired: 6 in, 2 out]
                  }
                  frame #1 {
                  }
                }
              }
              frame "CoolingON" {
                n604 = while {
                  tunnel: w1669 -> [w1704]
                  tunnel: w1668 -> [w1703]
                  tunnel: w1667 -> [w1699]
                  tunnel: [w1696] -> w1637
                  tunnel: w1664 -> [w1687]
                  tunnel: w1659 -> [w1673]
                  tunnel: w1658 -> [w1691]
                  tunnel: w1657 -> [w1688]
                  shift-right: [w1680] -> _
                  shift-left: 0.0 -> [w1681]
                  shift-right: [w1676] -> w1636
                  shift-left: 0.0 ("Value") -> [w1678]
                  tunnel: [w1671] -> w1640
                  stop <- w1685 stop-if-true
                  n605 = control-ref of="Power transistor Heat sink Temp."() -> (w1697:refnum<vi>)
                  n606 = property class="DigNum (strict)"(reference=w1697, error in=w1688) -> (error out=w1694:errorcluster, "Value"=w1676:dbl)  [unwired: 1 out]
                  n607 = Equal?(x=w1676, y=w1678) -> (x = y?=w1677:bool)
                  n608 = Number To Fractional String(number=w1676, precision (6)=i16 2) -> (F-format string=w1690:string)  [unwired: 2 in]
                  n609 = case shown="True" w1677 {
                    tunnel: w1681 -> [_ w1724]
                    tunnel: [0.0 w1722] -> w1680
                    tunnel: [FALSE w1721] -> w1679
                    frame False {
                    }
                    frame True {
                      n610 = Increment(x=w1724) -> (x+1=w1722:dbl)
                      n611 = Greater Or Equal?(x=w1722, y=300.0) -> (x >= y?=w1721:bool)
                    }
                  }
                  n612 = Concatenate Strings(w1691, "\nPCB Temperature [C]: " ("string"), w1690) -> (w1689:string)
                  n613 = call "Write panel message (SubVI).vi"("Stop BurnIn"=w1703, 4:"rpm"=w1699, 5:"rpm"=FALSE ("rpm"), "PrintTime"=FALSE, "Stop"=w1687, "error in (no error)"=w1694, "Time to wait"=0.2, "Strin"=w1689, "String in"=w1704) -> ("error out"=w1693:errorcluster)  [unwired: 2 in]
                  n614 = property class="Bool (strict)"(reference=w1687) -> ("Value"=w1686:bool)  [unwired: 1 in, 2 out]
                  n615 = Less Or Equal?(x=w1676, y=52.0) -> (x <= y?=w1675:bool)
                  n616 = call "GetADCTester (SubVI).vi"("error in (no error)"=w1693, "GetADCTester"=T13."Fan", "VISA Refnum in"=w1673) -> ("error out"=w1696:errorcluster, "ADCValOutput Single"=w1683:dbl)  [unwired: 6 in, 1 out]
                  n617 = Greater?(x=w1683, y=u32 2400) -> (0:w1672:bool)
                  n618 = case shown="True" w1675 {
                    tunnel: [w1711 w1718] -> w1674
                    tunnel: w1675 -> [w1711 w1718]
                    tunnel: w1673 -> [w1709 w1716]
                    tunnel: [w1705 w1712] -> w1671
                    frame False {
                      n619 = call "Time Delay11"() -> ("error out"=w1708:errorcluster)  [unwired: 11 in]
                      n620 = call "GetADCTester (SubVI).vi"("error in (no error)"=w1708, "GetADCTester"=T13."Fan", "VISA Refnum in"=w1709) -> ("ADCValOutput Single"=w1707:dbl)  [unwired: 6 in, 2 out]
                      n621 = Greater?(x=w1707, y=2400.0) -> (0:w1705:bool)
                    }
                    frame True {
                      n622 = call "Time Delay10"() -> ("error out"=w1715:errorcluster)  [unwired: 11 in]
                      n623 = call "GetADCTester (SubVI).vi"("error in (no error)"=w1715, "GetADCTester"=T13."Fan", "VISA Refnum in"=w1716) -> ("ADCValOutput Single"=w1714:dbl)  [unwired: 6 in, 2 out]
                      n624 = Greater?(x=w1714, y=2400.0) -> (0:w1712:bool)
                    }
                  }
                  n625 = Compound Arithmetic op=OR(w1672, w1686, w1674, w1679) -> (w1685:bool)
                }
                n626 = In Range and Coerce(upper limit=56.0, x=w1636, lower limit=52.0) -> (In Range?=w1639:bool)  [unwired: 1 out]
                n627 = Build Array(w1640, w1639) -> (w1641:bool[])
                n628 = And Array Elements(Boolean array=w1641) -> (logical AND=→"AuxiOFFResult":bool)
                n629 = Add(x=w1652, y=3) -> (x+y=w1650:i32)
                n630 = call "PassOrFail (SubVI).vi"("index (row)"=w1650, "error in (no error)"=w1637, "Data in"=w1636, "Pass?Fail"=w1639, "Table in"=w1648) -> ("error out"=w1654:errorcluster)  [unwired: 6 in]
                n631 = Select(t="OFF", s=w1640, f="ON") -> (s? t:f=w1644:string)
                n632 = Increment(x=w1650) -> (x+1=w1649:i32)
                n633 = call "PassOrFail (SubVI).vi"("String Res"=w1644, "index (row)"=w1649, "error in (no error)"=w1654, "Data in"=-3.0, "Pass?Fail"=w1640, "Table in"=w1648) -> ("error out"=w1653:errorcluster)  [unwired: 5 in]
                n634 = call "TesterOption (SubVI).vi"("2 Options"=FALSE, "error in (no error)"=w1653, "On/Off"=FALSE, "Tester Option"=T11."Venable" ("Tester Option 2"), "VISA Refnum in"=w1659) -> ("error out"=w1634:errorcluster)  [unwired: 5 in, 1 out]
                n635 = call "Time Delay14"("error in (no error)"=w1634) -> ("error out"=w1633:errorcluster)  [unwired: 10 in]
                n636 = property class="Bool (strict)"(reference=w1664, error in=w1633) -> ("Value"=w1670:bool)  [unwired: 2 out]
                n637 = Select(t=enum16{"Stop", "CoolingON", "HotGunON", "Start"}."Stop", s=w1670, f=enum16{"Stop", "CoolingON", "HotGunON", "Start"}."Stop") -> (s? t:f=w1661:enum16{"Stop", "CoolingON", "HotGunON", "Start"})
              }
              frame "HotGunON" {
                n638 = while {
                  tunnel: w1764 -> [w1797]
                  tunnel: w1763 -> [w1796]
                  tunnel: w1762 -> [w1792]
                  tunnel: [w1788] -> w1734
                  tunnel: w1759 -> [w1779]
                  tunnel: w1754 -> [w1789]
                  tunnel: w1753 -> [w1783]
                  tunnel: w1752 -> [w1780]
                  shift-right: [w1772] -> _
                  shift-left: 0.0 -> [w1773]
                  shift-right: [w1769] -> _
                  shift-left: 0.0 ("Value") -> [w1770]
                  tunnel: [w1767] -> w1732
                  stop <- w1777 stop-if-true
                  n639 = control-ref of="Power transistor Heat sink Temp."() -> (w1790:refnum<vi>)
                  n640 = property class="DigNum (strict)"(reference=w1790, error in=w1780) -> (error out=w1786:errorcluster, "Value"=w1769:dbl)  [unwired: 1 out]
                  n641 = Equal?(x=w1769, y=w1770) -> (x = y?=w1768:bool)
                  n642 = Number To Fractional String(number=w1769, precision (6)=i16 2) -> (F-format string=w1782:string)  [unwired: 2 in]
                  n643 = case shown="True" w1768 {
                    tunnel: w1773 -> [_ w1803]
                    tunnel: [0.0 w1801] -> w1772
                    tunnel: [FALSE w1800] -> w1771
                    frame False {
                    }
                    frame True {
                      n644 = Increment(x=w1803) -> (x+1=w1801:dbl)
                      n645 = Greater Or Equal?(x=w1801, y=300.0) -> (x >= y?=w1800:bool)
                    }
                  }
                  n646 = Concatenate Strings(w1783, "\nPCB Temperature [C]: " ("string"), w1782) -> (w1781:string)
                  n647 = call "Write panel message (SubVI).vi"("Stop BurnIn"=w1796, 4:"rpm"=w1792, 5:"rpm"=FALSE ("rpm"), "PrintTime"=FALSE, "Stop"=w1779, "error in (no error)"=w1786, "Time to wait"=0.2, "Strin"=w1781, "String in"=w1797) -> ("error out"=w1785:errorcluster)  [unwired: 2 in]
                  n648 = property class="Bool (strict)"(reference=w1779) -> ("Value"=w1778:bool)  [unwired: 1 in, 2 out]
                  n649 = call "GetADCTester (SubVI).vi"("error in (no error)"=w1785, "GetADCTester"=T13."Fan", "VISA Refnum in"=w1789) -> ("error out"=w1788:errorcluster, "ADCValOutput Single"=w1775:dbl)  [unwired: 6 in, 1 out]
                  n650 = Greater Or Equal?(x=w1769, y=61.0) -> (x >= y?=w1766:bool)
                  n651 = Less?(x=w1775, y=u32 100) -> (x < y?=w1767:bool)
                  n652 = Compound Arithmetic op=OR(w1767, w1778, w1766, w1771) -> (w1777:bool)
                }
                n653 = control-ref of="Power transistor Heat sink Temp."() -> (w1737:refnum<vi>)
                n654 = property class="DigNum (strict)"(reference=w1737, error in=w1734) -> (error out=w1736:errorcluster, "Value"=w1735:dbl)  [unwired: 1 out]
                n655 = In Range and Coerce(upper limit=62.0, x=w1735, lower limit=58.0) -> (In Range?=w1731:bool)  [unwired: 1 out]
                n656 = Build Array(w1732, w1731) -> (w1733:bool[])
                n657 = Increment(x=w1747) -> (x+1=w1746:i32)
                n658 = call "PassOrFail (SubVI).vi"("index (row)"=w1746, "error in (no error)"=w1736, "Data in"=w1735, "Pass?Fail"=w1731, "Table in"=w1744) -> ("error out"=w1749:errorcluster)  [unwired: 6 in]
                n659 = And Array Elements(Boolean array=w1733) -> (logical AND=→"AuxiONResult":bool)
                n660 = Increment(x=w1746) -> (x+1=w1745:i32)
                n661 = Select(t="ON", s=w1732, f="OFF") -> (s? t:f=w1742:string)
                n662 = call "PassOrFail (SubVI).vi"("String Res"=w1742, "index (row)"=w1745, "error in (no error)"=w1749, "Data in"=-3.0, "Pass?Fail"=w1732, "Table in"=w1744) -> ("error out"=w1748:errorcluster)  [unwired: 5 in]
                n663 = call "TesterOption (SubVI).vi"("On/Off 2"=FALSE, "Tester Option 2"=T11."Venable", "2 Options"=TRUE, "error in (no error)"=w1748, "On/Off"=FALSE, "Tester Option"=T11."Fan", "VISA Refnum in"=w1754) -> ("error out"=w1726:errorcluster)  [unwired: 3 in, 1 out]
                n664 = call "Time Delay13"("error in (no error)"=w1726) -> ("error out"=w1725:errorcluster)  [unwired: 10 in]
                n665 = property class="Bool (strict)"(reference=w1759, error in=w1725) -> ("Value"=w1765:bool)  [unwired: 2 out]
                n666 = Select(t=enum16{"Stop", "CoolingON", "HotGunON", "Start"}."Stop", s=w1765, f=enum16{"Stop", "CoolingON", "HotGunON", "Start"}."CoolingON") -> (s? t:f=w1756:enum16{"Stop", "CoolingON", "HotGunON", "Start"})
              }
              frame "Start" {
                n667 = call "Write panel message (SubVI).vi"("Stop BurnIn"=w1823, 4:"rpm"=w1819, 5:"rpm"=FALSE ("rpm"), "PrintTime"=TRUE, "Stop"=w1810, "Time to wait"=3.0, "Strin"=w1818, "String in"=w1824) -> ("error out"=w1817:errorcluster)  [unwired: 3 in]
                n668 = call "TesterOption (SubVI).vi"("On/Off 2"=TRUE, "Tester Option 2"=T11."Fan", "2 Options"=TRUE, "error in (no error)"=w1817, "On/Off"=FALSE, "Tester Option"=T11."Venable", "VISA Refnum in"=w1811) -> ("error out"=w1809:errorcluster)  [unwired: 3 in, 1 out]
                n669 = call "Time Delay"("error in (no error)"=w1809) -> ("error out"=w1804:errorcluster)  [unwired: 10 in]
                n670 = property class="Bool (strict)"(reference=w1810, error in=w1804) -> ("Value"=w1825:bool)  [unwired: 2 out]
                n671 = Select(t=enum16{"Stop", "CoolingON", "HotGunON", "Start"}."Stop", s=w1825, f=enum16{"Stop", "CoolingON", "HotGunON", "Start"}."HotGunON") -> (s? t:f=w1806:enum16{"Stop", "CoolingON", "HotGunON", "Start"})
              }
            }
          }
        }
      }
    }
    n672 = flat-sequence {
      tunnel: w187 -> [_]
      frame #0 {
        w195 = T20."Enabled" ("Disabled")
        w196 = FALSE ("Start")
        n673 = property on="Start" class="Bool (strict)"("Value"=w196, "DisabledEnum"=w195) -> ()  [unwired: 2 in, 2 out]
        n674 = property on="Report" class="Bool (strict)"("Value"=w196, "DisabledEnum"=w195) -> ()  [unwired: 2 in, 2 out]
      }
    }
  }
  n675 = while {
    shift-right: [w1844] -> _
    shift-left: T10."Initialize" -> [w1843]
    shift-right: [w1840] -> _
    shift-left: _ -> [w1839]
    shift-right: [w1838] -> _
    shift-left: w23 -> [w1836]
    shift-right: [w1837] -> _
    shift-left: refnum<vi> refnum ("Config_CANAT") -> [w1835]
    shift-right: [w1833] -> _
    shift-left: w20 -> [w1834]
    tunnel: "ATR" -> [_]
    tunnel: w11 -> [w1832]
    tunnel: w10 -> [w1831]
    shift-right: [w1829] -> _
    shift-left: 0 -> [w1830]
    tunnel: w8 -> [w1828]
    tunnel: w6 -> [w1827]
    tunnel: w5 -> [_]
    tunnel: w21 -> [w1842]
    tunnel: [w1841] -> _
    stop <- w1826 stop-if-true
    n676 = case shown="\"MainProgram\"" w1843 {
      tunnel: [T10."MainProgram" w1948 w2018 T10."Erase ATR Table"] -> w1844
      tunnel: [FALSE w1934 FALSE FALSE] -> w1826
      tunnel: [w1852 w1939 w2012 w2856] -> w1841
      tunnel: w1842 -> [_ w1959 w2016 _]
      tunnel: [w1889 refnum<visa-resource-name> refnum ("VISA resource name") w2013 w2861] -> w1840
      tunnel: w1839 -> [w1889 w1967 w2014 _]
      tunnel: [w1879 w1928 w2008 w2854] -> w1838
      tunnel: [w1878 refnum<vi> refnum ("Config_CANAT") w2009 w2857] -> w1837
      tunnel: w1836 -> [w1879 w1969 w2011 w2854]
      tunnel: w1835 -> [w1878 w1951 w2010 _]
      tunnel: w1834 -> [w1877 w1962 w2007 w2853]
      tunnel: [w1877 w1927 w2006 w2853] -> w1833
      tunnel: w1832 -> [_ _ w2005 _]
      tunnel: w1831 -> [_ _ w2004 _]
      tunnel: w1830 -> [w1866 w1953 w2003 w2850]
      tunnel: [w1866 w1953 w2002 w2850] -> w1829
      tunnel: w1828 -> [w1856 _ w2001 _]
      tunnel: w1827 -> [_ _ w2000 _]
      frame "Erase ATR Table", Default {
        w1845 = T20."Enabled" ("Disabled")
        w1860 = "Marvin" ("section")
        w1873 = refnum<visa-resource-name> "COM4" ("VISA resource name")
        w1884 = FALSE ("Visible")
        n677 = property on="Serial Com" class="Bool"(error in=errorcluster {"status"=FALSE, "code"=0, "source"=""} ("error out"), "Visible"=TRUE) -> (error out=w1874:errorcluster)  [unwired: 1 in, 1 out]
        n678 = property on="VISA Marvin" class="VISAName"(error in=w1874, "Visible"=w1884, "Value"=w1873) -> (error out=w1886:errorcluster)  [unwired: 1 in, 1 out]
        n679 = property on="VISA Marvin" class="VISAName"(error in=w1874, "Value"=w1873) -> ()  [unwired: 1 in, 2 out]
        n680 = property on="Status" class="Bool (strict)"(error in=w1886, "Value"=w1884) -> (error out=w1848:errorcluster)  [unwired: 1 in, 1 out]
        n681 = call "Select UUT"("error in (no error)"=w1848) -> ("EBAY"=w1846:bool, "error out"=w1847:errorcluster)  [unwired: 17 in]
        n682 = case shown="True" w1846 {
          tunnel: [string[][] [["1", "Communication Test", "", "", "", "", ""], ["1.1", "Serial RS-232", "N/A", "-", "", "", ""], ["1.2", "CAN Bus", "N/A", "-", "", "", ""], ["", "", "", "", "", "", ""], ["2", "Temperature Sensor Calibration", "", "", "", "", ""], ["2.1", "Sensor Reading Analog Offset", "0", "+/-0.100", ".", "", ""], ["", "", "", "", "", "", ""], ["3", "Motor Termistor Input Test", "", "", "", "", ""], ["3.1", "60 Degree", "60", "+/-3.00", "C", "", ""], ["3.2", "90 Degree", "90", "+/-3.00", "C", "", ""], ["3.3", "120 Degree", "120", "+/-3.00", "C", "", ""], ["", "", "", "", "", "", ""], ["4", "Enable Test", "", "", "", "", ""], ["4.1", "Fan Speed at Opened Enable ", "5000", "+/-200.0", "rpm", "", ""], ["4.2", "Fan Speed at Opened Enable ", "0", "+/-200.0", "rpm", "", ""], ["4.3", "Fan Speed at Closed Enable ", "5000", "+/-200.0", "rpm", "", ""], ["4.4", "Motor Rotation Direction", "Counter-clockwise (Inlet)", "-", "", "", ""], ["", "", "", "", "", "", ""], ["5", "Speed Command Test", "", "", "", "", ""], ["5.1", "Fan Speed", "6000", "+/-200.0", "rpm", "", ""], ["5.2", "Fan Speed", "9000", "+/-200.0", "rpm", "", ""], ["5.3", "Fan Speed", "12100", "+/-200.0", "rpm", "", ""], ["", "", "", "", "", "", ""], ["6", "Motor Stop time", "< 50", "-", "sec", "", ""], ["", "", "", "", "", "", ""], ["7", "Burn-in Test", "", "", "", "", ""], ["7.1", "DC Input Current", "28", "+/-5.000", "A", "", ""], ["7.2", "Fan Speed", "12100", "+/-200.0", "rpm", "", ""], ["7.3", "Ambient Temperature", "25", "+/-13.00", "C", "", ""], ["7.4", "After 10 min of operation", "", "-", "C", "", ""], ["7.5", "After 20 min of operation", "", "-", "C", "", ""], ["7.6", "After 30 min of operation", "", "-", "C", "", ""], ["", "", "", "", "", "", ""], ["8", "Visual Inspection", "", "", "", "", ""], ["8.1", "Verification of Components Not Installed", "N/A", "-", "", "", ""], ["8.2", "Manufacturing Defects", "N/A", "-", "", "", ""], ["", "", "", "", "", "", ""], ["9", "Power Supply Testing", "", "", "", "", ""], ["9.1", "Input Current Drawn", "", "", "", "", ""], ["9.2", "DC Input Current", "< 150", "-", "mA", "", ""], ["", "", "", "", "", "", ""], ["10", "Power Supply Voltages", "", "", "", "", ""], ["10.1", "12V", "12.0", "+/-0.500", "V", "", ""], ["10.2", "5V", "5.0", "+/-0.200", "V", "", ""], ["10.3", "3.3V", "3.3", "+/-0.100", "V", "", ""], ["10.4", "1.8V", "1.8", "+/-0.100", "V", "", ""], ["", "", "", "", "", "", ""], ["11", "Reverse Polarity Test - DC Input Current", "< 1", "-", "mA", "", ""], ["", "", "", "", "", "", ""], ["12", "Functional Test Procedure", "", "", "", "", ""], ["12.1", "Weight Check", "4180", "+/-10.00", "gr", "", ""], ["", "", "", "", "", "", ""], ["13", "Insulation Resistance Test", "", "", "", "", ""], ["13.1", "J3.B to Chassis", "> 1M", "-", "ohms", "", ""], ["13.2", "J1.16 to Chassis", "> 100K", "-", "ohms", "", ""], ["", "", "", "", "", "", ""], ["14", "Bonding Resistance", "", "", "", "", ""], ["14.1", "J1 Body to Chassis", "< 2m", "-", "ohms", "", ""], ["14.2", "J2  Body to Chassis", "< 2m", "-", "ohms", "", ""], ["14.3", "J3  Body to Chassis", "< 2m", "-", "ohms", "", ""], ["", "", "", "", "", "", ""], ["15", "CANbus Resistance Test", "", "", "", "", ""], ["15.1", "J1.17 to J1.18", "> 10K", "-", "ohms", "", ""], ["", "", "", "", "", "", ""], ["16", "Sealing Test", "N/A", "-", "", "", ""]] ("ArrAHU 2") string[][] [["1", "Communication Test", "", "", "", "", ""], ["1.1", "Serial RS-232", "N/A", "-", "", "", ""], ["1.2", "CAN Bus", "N/A", "-", "", "", ""], ["", "", "", "", "", "", ""], ["2", "Temperature Sensor Calibration", "", "", "", "", ""], ["2.1", "Sensor Reading Analog Offset", "0", "+/-0.100", ".", "", ""], ["", "", "", "", "", "", ""], ["3", "Motor Termistor Input Test", "", "", "", "", ""], ["3.1", "60 Degree", "60", "+/-3.00", "C", "", ""], ["3.2", "90 Degree", "90", "+/-3.00", "C", "", ""], ["3.3", "120 Degree", "120", "+/-3.00", "C", "", ""], ["", "", "", "", "", "", ""], ["4", "Enable Test", "", "", "", "", ""], ["4.1", "Fan Speed at Opened Enable ", "5000", "+/-200.0", "rpm", "", ""], ["4.2", "Fan Speed at Opened Enable ", "0", "+/-200.0", "rpm", "", ""], ["4.3", "Fan Speed at Closed Enable ", "5000", "+/-200.0", "rpm", "", ""], ["4.4", "Motor Rotation Direction", "Counter-clockwise (Inlet)", "-", "", "", ""], ["", "", "", "", "", "", ""], ["5", "Speed Command Test", "", "", "", "", ""], ["5.1", "Fan Speed", "6000", "+/-200.0", "rpm", "", ""], ["5.2", "Fan Speed", "11500", "+/-200.0", "rpm", "", ""], ["5.3", "Fan Speed", "15100", "+/-200.0", "rpm", "", ""], ["", "", "", "", "", "", ""], ["6", "Motor Stop time", "< 50", "-", "sec", "", ""], ["", "", "", "", "", "", ""], ["7", "Temperature Control Algorithm Test", "", "", "", "", ""], ["7.1", "Tair <   68 ± 2 oC", "6000", "+/-200.0", "rpm", "", ""], ["7.2", "Measured Temp.", "", "", "C", "", ""], ["7.3", "Tair >= 68 ± 2 oC", "11500", "+/-200.0", "rpm", "", ""], ["7.4", "Transition Temp.", "", "", "C", "", ""], ["7.5", "Tair >= 88 ± 2 oC", "15100", "+/-400.0", "rpm", "", ""], ["7.6", "Transition Temp.", "", "", "C", "", ""], ["7.7", "Tair <= 80 ± 2 oC", "11500", "+/-200.0", "rpm", "", ""], ["7.8", "Transition Temp.", "", "", "C", "", ""], ["7.9", "Tair <= 60 ± 2 oC", "6000", "+/-200.0", "rpm", "", ""], ["7.10", "Transition Temp.", "", "", "C", "", ""], ["", "", "", "", "", "", ""], ["8", "Burn-in Test", "", "", "", "", ""], ["8.1", "DC Input Current", "50", "+/-5.000", "A", "", ""], ["8.2", "Fan Speed", "15100", "+/-200.0", "rpm", "", ""], ["8.3", "Ambient Temperature", "25", "+/-13.00", "C", "", ""], ["8.4", "After 10 min of operation", "", "-", "C", "", ""], ["8.5", "After 20 min of operation", "", "-", "C", "", ""], ["8.6", "After 30 min of operation", "", "-", "C", "", ""], ["", "", "", "", "", "", ""], ["9", "Auxiliary Fan Test", "", "", "", "", ""], ["9.1", "Auxiliary Cooling Fan ON", "60", "+/-2.00", "C", "", ""], ["9.2", "Fan status", "ON", "-", "-", "", ""], ["9.3", "Auxiliary Cooling Fan OFF", "54", "+/-2.00", "C", "", ""], ["9.4", "Fan status", "OFF", "-", "-", "", ""], ["", "", "", "", "", "", ""], ["10", "Visual Inspection", "", "", "", "", ""], ["10.1", "Verification of Components Not Installed", "N/A", "-", "", "", ""], ["10.2", "Manufacturing Defects", "N/A", "-", "", "", ""], ["", "", "", "", "", "", ""], ["11", "Power Supply Testing", "", "", "", "", ""], ["11.1", "DC Input Current Drawn", "< 150", "-", "mA", "", ""], ["", "", "", "", "", "", ""], ["12", "Power Supply Voltages", "", "", "", "", ""], ["12.1", "12V", "12.0", "+/-0.500", "V", "", ""], ["12.2", "5V", "5.0", "+/-0.200", "V", "", ""], ["12.3", "3.3V", "3.3", "+/-0.100", "V", "", ""], ["12.4", "1.8V", "1.8", "+/-0.100", "V", "", ""], ["", "", "", "", "", "", ""], ["13", "Reverse Polarity Test - DC Input Current", "< 1", "-", "mA", "", ""], ["", "", "", "", "", "", ""], ["14", "Functional Test Procedure", "", "", "", "", ""], ["14.1", "Weight Check", "4180", "+/-10.00", "gr", "", ""], ["", "", "", "", "", "", ""], ["15", "Insulation Resistance Test", "", "", "", "", ""], ["15.1", "J3.B to Chassis", "> 1M", "-", "ohms", "", ""], ["15.2", "J1.16 to Chassis", "> 100K", "-", "ohms", "", ""], ["", "", "", "", "", "", ""], ["16", "Bonding Resistance", "", "", "", "", ""], ["16.1", "J1 Body to Chassis", "< 2m", "-", "ohms", "", ""], ["16.2", "J2  Body to Chassis", "< 2m", "-", "ohms", "", ""], ["16.3", "J3  Body to Chassis", "< 2m", "-", "ohms", "", ""], ["", "", "", "", "", "", ""], ["17", "CANbus Resistance Test", "", "", "", "", ""], ["17.1", "J1.17 to J1.18", "> 10K", "-", "ohms", "", ""], ["", "", "", "", "", "", ""], ["18", "Sealing Test", "N/A", "-", "", "", ""]] ("ArrEbay 2")] -> w1882
          tunnel: ["AHU" "EBAY"] -> w1881
          tunnel: [w1899 w1911] -> w1880
          tunnel: w1847 -> [w1900 w1911]
          tunnel: [w1895 u8 95] -> w1853
          frame False {
            (unwired) string[][] [["6.1", "Visual Inspection", "", "", "", "", ""], ["6.1.1", "Verification of Components Not Installed", "N/A", "-", "", "", ""], ["", "", "", "", "", "", ""], ["6.1.2", "Manufacturing Defects", "N/A", "-", "", "", ""], ["", "", "", "", "", "", ""], ["6.2", "Power Supply Testing", "", "", "", "", ""], ["6.2.1", "Input Current Drawn", "", "", "", "", ""], ["6.2.1.1", "DC Input Current", "< 150", "-", "mA", "", ""], ["", "", "", "", "", "", ""], ["6.2.2", "Power Supply Voltages", "", "", "", "", ""], ["6.2.2.1", "12V", "12.0", "+/-0.500", "V", "", ""], ["6.2.2.2", "5V", "5.0", "+/-0.200", "V", "", ""], ["6.2.2.3", "3.3V", "3.3", "+/-0.100", "V", "", ""], ["6.2.2.4", "1.8V", "1.8", "+/-0.100", "V", "", ""], ["", "", "", "", "", "", ""], ["7", "Functional Test Procedure", "", "", "", "", ""], ["7.1", "Weight Check", "3800", "+/-100.0", "gr", "", ""], ["", "", "", "", "", "", ""], ["7.2", "Insulation Resistance Test", "", "", "", "", ""], ["7.2.1", "J3.B to Chassis", "> 1M", "-", "W", "", ""], ["7.2.2", "J1.16 to Chassis", "> 100K", "-", "W", "", ""], ["", "", "", "", "", "", ""], ["7.2", "Bonding Resistance", "", "", "", "", ""], ["7.2.3", "J1 Body to Chassis", "< 2m", "-", "W", "", ""], ["7.2.4", "J2  Body to Chassis", "< 2m", "-", "W", "", ""], ["7.2.5", "J3  Body to Chassis", "< 2m", "-", "W", "", ""], ["", "", "", "", "", "", ""], ["7.2.1", "CANbus Resistance Test", "", "", "", "", ""], ["7.2.1.1", "J1.17 to J1.18", "> 10K", "-", "W", "", ""], ["", "", "", "", "", "", ""], ["7.3", "Sealing Test", "N/A", "-", "", "", ""], ["", "", "", "", "", "", ""], ["7.4", "Communication Test", "", "", "", "", ""], ["7.4.1", "Serial RS-232", "N/A", "-", "", "", ""], ["7.4.2", "CAN Bus", "N/A", "-", "", "", ""], ["", "", "", "", "", "", ""], ["7.5", "Performances Tests", "", "", "", "", ""], ["7.5.1", "Reverse Polarity Test", "", "", "", "", ""], ["7.5.1.1", "DC Input Current", "< 1", "-", "mA", "", ""], ["", "", "", "", "", "", ""], ["7.5.2", "Enable Test", "", "", "", "", ""], ["7.5.2.1", "Fan Speed at Opened Enable ", "5000", "+/-200.0", "rpm", "", ""], ["7.5.2.2", "Fan Speed at Opened Enable ", "0", "+/-200.0", "rpm", "", ""], ["7.5.2.3", "Fan Speed at Closed Enable ", "5000", "+/-200.0", "rpm", "", ""], ["7.5.2.4", "Motor Rotation Direction", "Counter-clockwise (Inlet)", "-", "", "", ""], ["", "", "", "", "", "", ""], ["7.5.3", "Stop Time Test ", "", "", "", "", ""], ["7.5.3.1", "Motor Stop time", "< 50", "-", "sec", "", ""], ["", "", "", "", "", "", ""], ["7.5.4", "Speed Command Test", "", "", "", "", ""], ["7.5.4.1", "Fan Speed", "6000", "+/-200.0", "rpm", "", ""], ["7.5.4.2", "Fan Speed", "9000", "+/-200.0", "rpm", "", ""], ["7.5.4.3", "Fan Speed", "12100", "+/-200.0", "rpm", "", ""], ["", "", "", "", "", "", ""], ["7.5.5", "Temperature Sensor Calibration Test", "", "", "", "", ""], ["7.5.5.1", "Sensor Reading Analog Offset", "0", "+/-0.100", ".", "", ""], ["", "", "", "", "", "", ""], ["7.5.6", "Burn-in Test", "", "", "", "", ""], ["7.5.6.1", "DC Input Current", "28", "+/-3.000", "A", "", ""], ["7.5.6.2", "Fan Speed", "12100", "+/-200.000", "rpm", "", ""], ["7.5.6.3", "Ambient Temperature", "25", "+/-13.00", "C", "", ""], ["7.5.6.4", "After 10 min of operation", "", "", "C", "", ""], ["7.5.6.5", "After 20 min of operation", "", "", "C", "", ""], ["7.5.6.6", "After 30 min of operation", "", "", "C", "", ""], ["", "", "", "", "", "", ""], ["9", "Motor Temp Test", "", "", "", "", ""], ["9.1", "60 C", "60", "+/-3.000", "C", "", ""], ["9.2", "90 C", "90", "+/-3.000", "C", "", ""], ["9.3", "120 C", "120", "+/-3.000", "C", "", ""]] ("data")
            n683 = while {
              shift-right: [w1907] -> w1899
              shift-left: w1900 -> [w1908]
              tunnel: [w1902] -> w1898
              stop <- w1906 stop-if-true
              n684 = call "AHU UUT (subVI).vi"("error in (no error)"=w1908) -> ("AHU 47"=w1903:bool, "AHU 63"=w1902:bool, "OK"=w1905:bool, "error out"=w1907:errorcluster)  [unwired: 15 in]
              n685 = Exclusive Or(1:w1903, 2:w1902) -> (0:w1904:bool)
              n686 = And(x=w1905, y=w1904) -> (x .and. y?=w1906:bool)
            }
            n687 = Select(t=u8 63, s=w1898, f=u8 47) -> (s? t:f=w1895:u8)
          }
          frame True {
            (unwired) string[][] [["6.1", "Visual Inspection", "", "", "", "", ""], ["6.1.1", "Verification of Components Not Installed", "N/A", "-", "", "", ""], ["", "", "", "", "", "", ""], ["6.1.2", "Manufacturing Defects", "N/A", "-", "", "", ""], ["", "", "", "", "", "", ""], ["6.2", "Power Supply Testing", "", "", "", "", ""], ["6.2.1", "Input Current Drawn", "", "", "", "", ""], ["6.2.1.1", "DC Input Current", "< 150", "-", "mA", "", ""], ["", "", "", "", "", "", ""], ["6.2.2", "Power Supply Voltages", "", "", "", "", ""], ["6.2.2.1", "12V", "12.0", "+/-0.500", "V", "", ""], ["6.2.2.2", "5V", "5.0", "+/-0.200", "V", "", ""], ["6.2.2.3", "3.3V", "3.3", "+/-0.100", "V", "", ""], ["6.2.2.4", "1.8V", "1.8", "+/-0.100", "V", "", ""], ["", "", "", "", "", "", ""], ["7", "Functional Test Procedure", "", "", "", "", ""], ["7.1", "Weight Check", "4180", "+/-10.00", "gr", "", ""], ["", "", "", "", "", "", ""], ["7.2", "Insulation Resistance Test", "", "", "", "", ""], ["7.2.1", "J3.B to Chassis", "> 1M", "-", "W", "", ""], ["7.2.2", "J1.16 to Chassis", "> 100K", "-", "W", "", ""], ["", "", "", "", "", "", ""], ["7.2", "Bonding Resistance", "", "", "", "", ""], ["7.2.3", "J1 Body to Chassis", "< 2m", "-", "W", "", ""], ["7.2.4", "J2  Body to Chassis", "< 2m", "-", "W", "", ""], ["7.2.5", "J3  Body to Chassis", "< 2m", "-", "W", "", ""], ["", "", "", "", "", "", ""], ["7.2.1", "CANbus Resistance Test", "", "", "", "", ""], ["7.2.1.1", "J1.17 to J1.18", "> 10K", "-", "W", "", ""], ["", "", "", "", "", "", ""], ["7.3", "Sealing Test", "N/A", "-", "", "", ""], ["", "", "", "", "", "", ""], ["7.4", "Communication Test", "", "", "", "", ""], ["7.4.1", "Serial RS-232", "N/A", "-", "", "", ""], ["7.4.2", "CAN Bus", "N/A", "-", "", "", ""], ["", "", "", "", "", "", ""], ["7.5", "Performances Tests", "", "", "", "", ""], ["7.5.1", "Reverse Polarity Test", "", "", "", "", ""], ["7.5.1.1", "DC Input Current", "< 1", "-", "mA", "", ""], ["", "", "", "", "", "", ""], ["7.5.2", "Enable Test", "", "", "", "", ""], ["7.5.2.1", "Fan Speed at Opened Enable ", "5000", "+/-200.0", "rpm", "", ""], ["7.5.2.2", "Fan Speed at Opened Enable ", "0", "+/-200.0", "rpm", "", ""], ["7.5.2.3", "Fan Speed at Closed Enable ", "5000", "+/-200.0", "rpm", "", ""], ["7.5.2.4", "Motor Rotation Direction", "Counter-clockwise (Inlet)", "-", "", "", ""], ["", "", "", "", "", "", ""], ["7.5.3", "Stop Time Test ", "", "", "", "", ""], ["7.5.3.1", "Motor Stop time", "< 50", "-", "sec", "", ""], ["", "", "", "", "", "", ""], ["7.5.4", "Speed Command Test", "", "", "", "", ""], ["7.5.4.1", "Fan Speed", "6000", "+/-200.0", "rpm", "", ""], ["7.5.4.2", "Fan Speed", "11500", "+/-200.0", "rpm", "", ""], ["7.5.4.3", "Fan Speed", "15100", "+/-200.0", "rpm", "", ""], ["", "", "", "", "", "", ""], ["7.5.5", "Temperature Sensor Calibration Test", "", "", "", "", ""], ["7.5.5.1", "Sensor Reading Analog Offset", "0", "+/-0.100", ".", "", ""], ["", "", "", "", "", "", ""], ["7.5.6", "Temperature Control Algorithm Test", "", "", "", "", ""], ["7.5.6.1", "Tair <   68 ± 2 oC", "6000", "+/-200.0", "rpm", "", ""], ["7.5.6.2", "Measured Temp.", "", "", "C", "", ""], ["7.5.6.3", "Tair >= 68 ± 2 oC", "11500", "+/-200.0", "rpm", "", ""], ["7.5.6.4", "Transition Temp.", "", "", "C", "", ""], ["7.5.6.5", "Tair >= 88 ± 2 oC", "15100", "+/-400.0", "rpm", "", ""], ["7.5.6.6", "Transition Temp.", "", "", "C", "", ""], ["7.5.6.7", "Tair <= 80 ± 2 oC", "11500", "+/-200.0", "rpm", "", ""], ["7.5.6.8", "Transition Temp.", "", "", "C", "", ""], ["7.5.6.9", "Tair <= 60 ± 2 oC", "6000", "+/-200.0", "rpm", "", ""], ["7.5.6.10", "Transition Temp.", "", "", "C", "", ""], ["", "", "", "", "", "", ""], ["7.5.7", "Burn-in Test", "", "", "", "", ""], ["7.5.7.1", "DC Input Current", "50", "+/-5.000", "A", "", ""], ["7.5.7.2", "Fan Speed", "15100", "+/-200.0", "rpm", "", ""], ["7.5.7.3", "Ambient Temperature", "25", "+/-13.00", "C", "", ""], ["7.5.7.4", "After 10 min of operation", "", "-", "C", "", ""], ["7.5.7.5", "After 20 min of operation", "", "-", "C", "", ""], ["7.5.7.6", "After 30 min of operation", "", "-", "C", "", ""], ["", "", "", "", "", "", ""], ["8", "Auxiliary", "", "", "", "", ""], ["8.1", "Auxiliary Cooling Fan ON", "60", "+/-2.00", "C", "", ""], ["8.2", "Fan status", "ON", "-", "-", "", ""], ["8.3", "Auxiliary Cooling Fan OFF", "55", "+/-2.00", "C", "", ""], ["8.4", "Fan status", "OFF", "-", "-", "", ""], ["", "", "", "", "", "", ""], ["9", "Motor Temp. Test", "", "", "", "", ""], ["9.1", "60 Degree", "60", "+/-3.00", "C", "", ""], ["9.2", "90 Degree", "90", "+/-3.00", "C", "", ""], ["9.3", "120 Degree", "120", "+/-3.00", "C", "", ""]] ("data")
          }
        }
        "UUT" <- w1881
        "UUT" <- w1853
        n688 = for {
          tunnel: w1882 -> [w1917] mode=indexing
          tunnel: w1880 -> [w1915]
          tunnel: [w1914] -> w1876
          tunnel: w1882 -> [w1913]
          i -> [w1916]
          n689 = for {
            tunnel: w1917 -> [_] mode=indexing
            tunnel: w1916 -> [w1923]
            tunnel: w1915 -> [w1920]
            tunnel: [w1919] -> w1914
            tunnel: w1913 -> [w1918]
            i -> [w1924]
            n690 = Bundle By Name(cluster=T21 {"Row"=0, "Column"=0} ("Active Cell:Active Cell"), "Row"=w1923, "Column"=w1924) -> (w1922:T21)
            n691 = control-ref of="ATR"() -> (w1921:refnum<vi>)
            n692 = property class="Tbl (strict)"(reference=w1921, error in=w1920, "Active Cell"=w1922, "Cell BG Color"=u32 16777226, "Value"=w1918) -> (error out=w1919:errorcluster)  [unwired: 1 out]
          }
        }
        n693 = call "COM EvolutionBoard.vi"("error in (no error)"=w1876, "VISA resource name 2"=refnum<visa-resource-name> "COM1" ("VISA resource name")) -> ("error out"=w1872:errorcluster, "VISA resource name out"=w1871:refnum<visa-resource-name>)  [unwired: 8 in]
        n694 = call "TesterOption (SubVI).vi"("2 Options"=FALSE, "error in (no error)"=w1872, "On/Off"=FALSE, "Tester Option"=T11."Venable", "VISA Refnum in"=w1871) -> ("error out"=w1852:errorcluster, "VISA Refnum out"=→"VISA Tester":refnum<visa-resource-name>)  [unwired: 5 in]
        n695 = case shown="95" w1853 {
          tunnel: ["AHU Software Version" ("key") "EBAY Software Version" ("key")] -> w1862
          tunnel: ["AHU Serial Number" ("key") "EBAY Serial Number" ("key")] -> w1863
          frame 47, 63, Default {
          }
          frame 95 {
          }
        }
        n696 = call <vilib>:"Open Config Data.vi"("create file if necessary (T)"=FALSE, "configuration file path"=w1856) -> ("error out"=w1857:errorcluster, "refnum"=w1858:T18)  [unwired: 1 in, 7 out]
        n697 = call-poly <vilib>:"Read Key.vi"("section"=w1860, "error in (no error)"=w1857, "key"=w1862, "refnum"=w1858) -> ("error out"=w1864:errorcluster, "value"=→"UUT SoftwareVer":string, "refnum out"=w1861:T18)  [unwired: 2 in, 3 out]
        n698 = property on="Start" class="Bool (strict)"("DisabledEnum"=w1845) -> ()  [unwired: 2 in, 2 out]
        n699 = property on="Report" class="Bool (strict)"("DisabledEnum"=w1845) -> ()  [unwired: 2 in, 2 out]
        n700 = call-poly <vilib>:"Read Key.vi"("section"=w1860, "error in (no error)"=w1864, "key"=w1863, "refnum"=w1861) -> ("error out"=w1851:errorcluster, "value"=w1849:string, "refnum out"=w1850:T18)  [unwired: 2 in, 3 out]
        n701 = call <vilib>:"Close Config Data.vi"("error in (no error)"=w1851, "refnum"=w1850) -> ()  [unwired: 8 in, 2 out]
        n702 = Decimal String To Number(string=w1849) -> (number=w1854:i32)  [unwired: 2 in, 1 out]
        n703 = Increment(x=w1854) -> (x+1=→"Next SN":i32)
      }
      frame "Stop" {
        n704 = flat-sequence {
          tunnel: w1959 -> [w1997]
          tunnel: [w1996] -> w1952
          frame #0 {
            n705 = control-ref of="Pannel User Message"() -> (w1999:refnum<vi>)
            n706 = property class="Str"(reference=w1999, error in=w1997, "Value"="Program Stopped...\r\nPlease turn OFF All Power sinks") -> (error out=w1996:errorcluster)  [unwired: 1 out]
          }
        }
        n707 = control-ref of="VISA Tester"() -> (w1960:refnum<vi>)
        n708 = property class="VISAName"(reference=w1960, error in=w1952) -> ("Value"=w1958:refnum<visa-resource-name>)  [unwired: 2 out]
        n709 = disable-structure shown="Enabled" {
          disable-tunnel: w1952 -> [w1984 w1985]
          disable-tunnel: w1951 -> [w1982 _]
          disable-tunnel: [w1981 w1985] -> w1938
          frame Disabled {
            n710 = call "Clear CAN Buffer.vi"("error in (no error)"=w1984, "Cluster in"=w1982) -> ("error out"=w1983:errorcluster)  [unwired: 8 in, 1 out]
            n711 = call "Close CAN Device.vi"("error in (no error)"=w1983, "Cluster in"=w1982) -> ("error out"=w1981:errorcluster)  [unwired: 8 in, 1 out]
          }
          frame Enabled {
          }
        }
        n712 = VISA Close(VISA resource name=w1967, error in (no error)=w1952) -> (error out=w1961:errorcluster)
        n713 = property on="Stop Button" class="Bool (strict)"() -> ("Value"=w1930:bool)  [unwired: 2 in, 2 out]
        n714 = call "TesterOption (SubVI).vi"("2 Options"=FALSE, "On/Off"=FALSE, "Tester Option"=T11."Power", "VISA Refnum in"=w1958) -> ("error out"=w1947:errorcluster, "VISA Refnum out"=w1957:refnum<visa-resource-name>)  [unwired: 6 in]
        n715 = property on="ClosePanel" class="Bool (strict)"() -> ("Value"=w1931:bool)  [unwired: 2 in, 2 out]
        n716 = VISA Close(VISA resource name=w1957, error in (no error)=w1947) -> (error out=w1944:errorcluster)
        n717 = Or(x=w1931, y=w1930) -> (x .or. y?=w1929:bool)
        n718 = Flush Queue(queue=w1962, error in (no error)=w1961) -> (queue out=w1964:refnum<queue>, error out=w1963:errorcluster)  [unwired: 1 out]
        n719 = Flush Queue(queue=w1969, error in (no error)=w1961) -> (queue out=w1968:refnum<queue>, error out=w1970:errorcluster)  [unwired: 1 out]
        n720 = case shown="False" w1929 {
          tunnel: w1970 -> [w1972 w1980]
          tunnel: w1968 -> [w1974 w1976]
          tunnel: w1964 -> [w1973 w1975]
          tunnel: w1963 -> [w1971 w1979]
          tunnel: [w1972 w1978] -> w1946
          tunnel: [w1971 w1977] -> w1945
          tunnel: [w1974 w1976] -> w1928
          tunnel: [w1973 w1975] -> w1927
          frame False {
          }
          frame True {
            n721 = Release Queue(queue=w1975, error in (no error)=w1979) -> (error out=w1977:errorcluster)  [unwired: 1 in, 2 out]
            n722 = Release Queue(queue=w1976, error in (no error)=w1980) -> (error out=w1978:errorcluster)  [unwired: 1 in, 2 out]
          }
        }
        n723 = Merge Errors(w1946, w1945, w1944, w1938) -> (w1943:errorcluster)
        n724 = property on="Refresh Button" class="Bool (strict)"() -> ("Value"=w1932:bool)  [unwired: 2 in, 2 out]
        n725 = call <vilib>:"Clear Errors.vi"("error in (no error)"=w1943) -> ("error out"=w1942:errorcluster)  [unwired: 5 in, 1 out]
        n726 = property on="Stop Button" class="Bool (strict)"() -> ("Value"=w1936:bool)  [unwired: 2 in, 2 out]
        n727 = property on="ClosePanel" class="Bool (strict)"(error in=w1942) -> (error out=w1940:errorcluster, "Value"=w1941:bool)  [unwired: 1 in, 1 out]
        n728 = Not(x=w1932) -> (.not. x?=w1933:bool)
        n729 = Select(t=T10."Initialize", s=w1932, f=T10."Stop") -> (s? t:f=w1948:T10)
        n730 = Not(x=w1936) -> (.not. x?=w1935:bool)
        n731 = Compound Arithmetic op=AND(w1941, w1935, w1933) -> (w1937:bool)
        n732 = case shown="False" w1937 {
          tunnel: w1940 -> [w1988 w1992]
          tunnel: [w1988 w1992] -> w1939
          tunnel: [w1987 w1991] -> w1934
          tunnel: w1932 -> [w1986 _]
          frame False {
            n733 = case shown="False" w1986 {
              tunnel: [TRUE FALSE] -> w1987
              frame False {
              }
              frame True {
              }
            }
          }
          frame True {
            n734 = flat-sequence {
              tunnel: [TRUE] -> w1991
              frame #0 {
              }
              frame #1 {
                n735 = control-ref of="This VI"() -> (w1995:refnum<vi>)
                n736 = property class="VI"(reference=w1995, "FP.State"=T22."Closed" ("Front Panel Window:State")) -> ()  [unwired: 1 in, 2 out]
              }
            }
          }
        }
      }
      frame "MainProgram" {
        n737 = event shown="[6] \"Start\": Value Change" {
          selector: w2005 -> [_ _ _ _ _ _ _ _ _ _ _ _ _]
          dyn-events: _ -> [_ _ _ _ _ _ _ _ _ _ _ _ _]
          timeout: 120 -> [_ _ _ _ _ _ _ _ _ _ _ _ _]
          tunnel: [T10."MainProgram" T10."MainProgram" T10."MainProgram" T10."MainProgram" T10."MainProgram" T10."Stop" T10."MainProgram" w2590 T10."MainProgram" T10."MainProgram" T10."MainProgram" T10."Stop" T10."MainProgram"] -> w2018
          tunnel: [w2020 w2113 w2178 w2185 w2194 w2212 w2237 w2649 w2715 w2728 w2738 w2819 w2825] -> w2012
          tunnel: w2016 -> [w2033 w2113 w2177 w2187 w2194 w2212 w2244 w2649 w2716 w2727 w2734 w2819 w2830]
          tunnel: [w2041 w2107 w2179 w2186 w2195 w2210 w2233 w2598 w2713 w2725 w2739 w2817 w2823] -> w2013
          tunnel: w2014 -> [w2041 w2107 w2179 w2186 w2195 w2210 w2233 w2598 w2713 w2725 _ w2817 w2823]
          tunnel: w2011 -> [w2035 w2119 w2173 w2182 w2191 w2209 w2242 w2629 w2712 w2724 w2742 w2816 w2828]
          tunnel: w2010 -> [w2030 w2118 w2174 w2183 w2192 w2208 w2215 w2628 w2711 w2723 w2741 w2815 w2821]
          tunnel: [w2032 w2118 w2174 w2183 w2192 w2208 w2215 w2628 w2711 w2723 w2741 w2815 w2821] -> w2009
          tunnel: [w2034 w2119 w2173 w2182 w2191 w2209 w2242 w2629 w2712 w2724 w2742 w2816 w2828] -> w2008
          tunnel: w2007 -> [w2028 w2117 w2172 w2181 w2190 w2207 w2241 w2627 w2710 w2722 w2740 w2814 w2827]
          tunnel: [w2028 w2117 w2172 w2181 w2190 w2207 w2236 w2627 w2710 w2722 w2740 w2814 w2827] -> w2006
          tunnel: w2004 -> [_ _ _ _ _ _ _ w2596 _ _ _ _ _]
          tunnel: w2003 -> [w2029 w2116 w2171 w2180 w2189 w2205 w2231 w2602 w2709 w2721 w2736 w2813 w2826]
          tunnel: [w2029 w2116 w2171 w2180 w2189 w2205 w2231 w2601 w2709 w2721 w2736 w2813 w2826] -> w2002
          tunnel: w2001 -> [_ w2114 _ _ _ _ _ w2600 _ _ _ _ _]
          tunnel: w2000 -> [_ w2106 _ _ _ _ _ _ _ _ _ _ _]
          event Timeout {
            n738 = event-data() -> ()  [unwired: 1 in, 3 out]
            n739 = property class="Clust (strict)"(reference=w2030, error in=w2033) -> (reference out=w2032:refnum<vi>, error out=w2031:errorcluster, "Value"=w2038:T7)
            n740 = Unbundle By Name(w2038) -> ("DevType"=w2039:T2, "CanIndex"=w2037:T1)
            n741 = property on="ClosePanel" class="Bool (strict)"("Value"=FALSE ("ClosePanel")) -> ()  [unwired: 2 in, 2 out]
            n742 = call "VCI_Receive.vi"("CANIndex"=w2037, "DevIndex"=u32 0, "DevType"=w2039) -> ("Recieve"=w2036:T26[])  [unwired: 3 in, 5 out]
            n743 = Empty Array?(array=w2036) -> (empty?=w2023:bool)
            n744 = case shown="False" w2023 {
              tunnel: w2037 -> [w2055 _]
              tunnel: w2032 -> [w2053 _]
              tunnel: w2035 -> [w2052 w2088]
              tunnel: w2031 -> [w2051 w2087]
              tunnel: w2036 -> [w2056 _]
              tunnel: [w2046 w2087] -> w2020
              tunnel: [w2045 w2088] -> w2034
              tunnel: [TRUE FALSE] -> w2019
              frame False {
                n745 = call "Demo_MakeDispBuff.vi"("Channel"=w2055, "Type"=enum16{"接收", "发送"}."接收", "OBJs"=w2056) -> ("Buffer"=w2054:T27)
                n746 = for {
                  N: 3 -> [_]
                  tunnel: w2054 -> [w2070]
                  tunnel: w2053 -> [w2069]
                  tunnel: w2052 -> [w2060]
                  tunnel: w2051 -> [w2059]
                  tunnel: [w2062] -> w2049 mode=indexing
                  tunnel: [w2060] -> w2048
                  tunnel: [w2059] -> w2047
                  i -> [w2058]
                  n747 = property class="Clust (strict)"(reference=w2069) -> ("Value"=w2067:T7)  [unwired: 1 in, 2 out]
                  n748 = Index Array(array=w2070, index=w2058) -> (element=w2063:T28)
                  n749 = Unbundle By Name(w2063) -> ("Channel"=w2065:T1, "VCI_CAN_OBJ"=w2068:T26)  [unwired: 2 out]
                  n750 = Unbundle By Name(w2067) -> ("CanIndex"=w2066:T1)
                  n751 = Equal?(x=w2066, y=w2065) -> (x = y?=w2064:bool)
                  n752 = case shown="True" w2064 {
                    tunnel: w2068 -> [_ w2081]
                    tunnel: [w2071 w2077] -> w2062
                    tunnel: T23 {"ID"=0, "MSGTYPE"=0, "LEN"=0, "aDATA"=[]} ("Msg") -> [w2071 w2076]
                    frame False {
                    }
                    frame True {
                      n753 = Unbundle By Name(w2081) -> ("ID"=w2075:u32, "DataLen"=w2080:u8, "Data"=w2078:u8[])
                      n754 = Bundle By Name(cluster=w2076, "ID"=w2075, "MSGTYPE"=u8 0, "LEN"=w2080, "aDATA"=w2078) -> (w2077:T23)
                      n755 = Unbundle By Name(w2077) -> ("ID"=w2073:u32)
                      n756 = Split Number(x=w2073) -> (lo(x)=w2074:u16)  [unwired: 1 out]
                      n757 = Split Number(x=w2074) -> (lo(x)=w2072:u8)  [unwired: 1 out]
                      n758 = case shown="63" w2072 {
                        tunnel: ["EBAY 5F" "" "AHU 3F" "AHU 2F"] -> _
                        frame 95 {
                        }
                        frame Default {
                        }
                        frame 63 {
                        }
                        frame 47 {
                        }
                      }
                    }
                  }
                }
                n759 = Enqueue Element(queue=w2048, element=w2049, error in (no error)=w2047) -> (queue out=w2045:refnum<queue>, error out=w2046:errorcluster)  [unwired: 2 out]
              }
              frame True {
              }
            }
            n760 = control-ref of="ATR"() -> (w2022:refnum<vi>)
            n761 = property on="CAN Status" class="Bool (strict)"("Value"=w2019) -> ()  [unwired: 2 in, 2 out]
            n762 = call "PassFailUUT (SubVI).vi"("error in (no error)"=w2020, "Table in"=w2022) -> ("PassFaileUUTresult"=w2021:bool)  [unwired: 7 in, 2 out]
            n763 = property on="Test Failed" class="Bool (strict)"("Value"=w2021) -> ()  [unwired: 2 in, 2 out]
            n764 = property on="Automation" class="Bool (strict)"() -> ("Value"=w2025:bool)  [unwired: 2 in, 2 out]
            n765 = property on="Start" class="Bool (strict)"() -> ("Value"=w2027:bool)  [unwired: 2 in, 2 out]
            n766 = Or(x=w2025, y=w2027) -> (x .or. y?=w2026:bool)
            n767 = case shown="False" w2026 {
              frame False {
                n768 = property on="Pannel User Message" class="Str"("Value"="You can press start to execute(s) test(s).") -> ()  [unwired: 2 in, 2 out]
              }
              frame True {
              }
            }
          }
          event "SetSN": Value Change {
            n769 = event-data() -> ()  [unwired: 1 in, 6 out]
            n770 = property on="UUT" class="DigNum (strict)"() -> ("Value"=w2097:u8)  [unwired: 2 in, 2 out]
            n771 = Equal?(x=w2097, y=u8 95) -> (x = y?=w2095:bool)
            n772 = control-ref of="ATR"() -> (w2098:refnum<vi>)
            n773 = Select(t=u8 50 ("y"), s=w2095, f=u8 36 ("y")) -> (s? t:f=w2090:u8)
            n774 = property on="Current SN" class="DigNum (strict)"(error in=w2113) -> (error out=w2092:errorcluster, "Value"=w2112:i32)  [unwired: 1 in, 1 out]
            n775 = call "PassFailUUT (SubVI).vi"("error in (no error)"=w2092, "Table in"=w2098) -> ("Total Pass"=w2091:u8)  [unwired: 7 in, 2 out]
            n776 = Equal To 0?(x=w2112) -> (x = 0?=w2109:bool)
            n777 = Equal?(x=w2112, y=-1) -> (x = y?=w2110:bool)
            n778 = Equal?(x=w2091, y=w2090) -> (x = y?=w2089:bool)
            n779 = Or(x=w2110, y=w2109) -> (x .or. y?=w2108:bool)
            n780 = property on="CAN Status" class="Bool (strict)"() -> ("Value"=w2099:bool)  [unwired: 2 in, 2 out]
            n781 = property on="Status" class="Bool (strict)"() -> ("Value"=w2104:bool)  [unwired: 2 in, 2 out]
            n782 = And(x=w2104, y=w2099) -> (x .and. y?=w2100:bool)
            n783 = case shown="True" w2100 {
              tunnel: w2114 -> [_ w2133]
              tunnel: w2108 -> [_ w2122]
              tunnel: w2107 -> [_ w2132]
              tunnel: w2106 -> [_ w2131]
              tunnel: [errorcluster {"status"=FALSE, "code"=0, "source"=""} ("error out") w2130] -> w2103
              tunnel: [w2120 w2129] -> w2105
              tunnel: w2089 -> [_ w2123]
              frame False {
                w2120 = FALSE ("Value")
                n784 = property on="SetSN" class="Bool (strict)"("Value"=w2120) -> ()  [unwired: 2 in, 2 out]
                n785 = call "Display Message to User10"() -> ()  [unwired: 10 in, 2 out]
              }
              frame True {
                n786 = property on="Test Failed" class="Bool (strict)"() -> ("Value"=w2127:bool)  [unwired: 2 in, 2 out]
                n787 = property on="Automation" class="Bool (strict)"() -> ("Value"=w2129:bool)  [unwired: 2 in, 2 out]
                n788 = Not(x=w2127) -> (.not. x?=w2128:bool)
                n789 = Select(t=w2128, s=w2129, f=w2131) -> (s? t:f=w2125:bool)
                n790 = Or(x=w2123, y=w2125) -> (x .or. y?=w2124:bool)
                n791 = And(x=w2122, y=w2124) -> (x .and. y?=w2126:bool)
                n792 = case shown="False" w2126 {
                  tunnel: w2133 -> [_ w2163]
                  tunnel: w2132 -> [_ w2156]
                  tunnel: [w2135 w2148] -> w2130
                  tunnel: w2122 -> [w2134 _]
                  frame False {
                    n793 = case shown="False" w2134 {
                      tunnel: [w2137 w2138] -> w2135
                      frame False {
                        n794 = call "Display Message to User9"() -> ("error out"=w2137:errorcluster)  [unwired: 10 in, 1 out]
                      }
                      frame True {
                        n795 = call "Display Message to User3"() -> ("error out"=w2138:errorcluster)  [unwired: 10 in, 1 out]
                      }
                    }
                    n796 = property on="Automation" class="Bool (strict)"(error in=w2135, "Value"=FALSE ("Automation")) -> ()  [unwired: 1 in, 2 out]
                  }
                  frame True {
                    w2155 = FALSE ("SetSN")
                    n797 = property on="Next SN" class="DigNum (strict)"() -> ("Value"=w2139:i32)  [unwired: 2 in, 2 out]
                    n798 = property on="VISA Tester" class="VISAName"() -> ("Value"=w2146:refnum<visa-resource-name>)  [unwired: 2 in, 2 out]
                    n799 = call "TesterOption (SubVI).vi"("2 Options"=FALSE, "On/Off"=FALSE, "Tester Option"=T11."Venable", "VISA Refnum in"=w2146) -> ("error out"=w2141:errorcluster)  [unwired: 6 in, 1 out]
                    n800 = call <vilib>:"Clear Errors.vi"("error in (no error)"=w2141) -> ("error out"=w2142:errorcluster)  [unwired: 5 in, 1 out]
                    n801 = Number To Decimal String(number=w2139) -> (decimal integer string=w2140:string)  [unwired: 1 in]
                    "UUT SN Report" <- w2140
                    n802 = Search and Replace String(input string="EP=1\r\nSN=0\r\n" ("write buffer"), search string="0", replace string=w2140) -> (result string=w2158:string)  [unwired: 5 in, 3 out]
                    n803 = call "SerialMarvinSendGet.vi"("error in (no error)"=w2142, "Clear Log"=FALSE, "write buffer"=w2158, "VISA resource name"=w2156) -> ("error out"=w2147:errorcluster)  [unwired: 6 in, 1 out]
                    n804 = property on="UUT" class="DigNum (strict)"(error in=w2147) -> ("Value"=w2164:u8)  [unwired: 1 in, 2 out]
                    n805 = case shown="47, 63, Default" w2164 {
                      tunnel: ["AHU Serial Number" ("key") "EBAY Serial Number" ("key")] -> w2167
                      frame 47, 63, Default {
                      }
                      frame 95 {
                      }
                    }
                    n806 = call <vilib>:"Open Config Data.vi"("create file if necessary (T)"=FALSE, "configuration file path"=w2163) -> ("error out"=w2161:errorcluster, "refnum"=w2162:T18)  [unwired: 1 in, 7 out]
                    n807 = call-poly <vilib>:"Write Key.vi"("section"="Marvin", "error in (no error)"=w2161, "value"=w2140, "key"=w2167, "refnum"=w2162) -> ("error out"=w2151:errorcluster, "refnum out"=w2150:T18)  [unwired: 4 in, 1 out]
                    n808 = call <vilib>:"Close Config Data.vi"("error in (no error)"=w2151, "refnum"=w2150) -> ("error out"=w2149:errorcluster)  [unwired: 8 in, 1 out]
                    n809 = property on="Current SN" class="DigNum (strict)"("Value"=w2139) -> ()  [unwired: 2 in, 2 out]
                    n810 = property on="SetSN" class="Bool (strict)"(error in=w2149, "Value"=w2155) -> (error out=w2154:errorcluster)  [unwired: 1 in, 1 out]
                    n811 = property on="Automation" class="Bool (strict)"(error in=w2154, "Value"=w2155) -> (error out=w2153:errorcluster)  [unwired: 1 in, 1 out]
                    n812 = Increment(x=w2139) -> (x+1=w2152:i32)
                    n813 = property on="Next SN" class="DigNum (strict)"(error in=w2153, "Value"=w2152) -> (error out=w2148:errorcluster)  [unwired: 1 in, 1 out]
                  }
                }
              }
            }
            n814 = property on="SetSN" class="Bool (strict)"(error in=w2103, "Value"=FALSE ("SetSN")) -> (error out=w2102:errorcluster)  [unwired: 1 in, 1 out]
            n815 = case shown="True" w2105 {
              tunnel: w2102 -> [_ _]
              frame False {
              }
              frame True {
                w2170 = TRUE ("Value (Signaling)")
                n816 = property on="Report" class="Bool (strict)"("Val(Sgnl)"=w2170, "Value"=w2170) -> ()  [unwired: 2 in, 2 out]
              }
            }
          }
          event "ATR": Mouse Enter {
            n817 = event-data() -> ()  [unwired: 1 in, 4 out]
            n818 = call-poly <vilib>:"Set Cursor.vi"("error in (no error)"=w2177, "icon"=u16 1) -> ("error out"=w2178:errorcluster)  [unwired: 8 in, 1 out]
          }
          event "ATR": Mouse Leave {
            n819 = event-data() -> ()  [unwired: 1 in, 4 out]
            n820 = call-poly <vilib>:"Set Cursor.vi"("error in (no error)"=w2187, "icon"=u16 0) -> ("error out"=w2185:errorcluster)  [unwired: 8 in, 1 out]
          }
          event "ATR": Mouse Down? {
            n821 = event-data() -> ("Coords"=w2202:T29)  [unwired: 1 in, 4 out]
            n822 = invoke on="ATR" class="Tbl (strict)" method="Point To Row Column"("Point"=w2202) -> ("InBounds"=w2198:bool, "CellPosition"=w2197:T21)  [unwired: 5 in, 4 out]
            n823 = Greater Than 0?(x=w2197) -> (x > 0?=w2201:cluster{"Row":bool, "Column":bool})
            n824 = Cluster To Array(cluster=w2201) -> (array=w2200:bool[])
            n825 = Or Array Elements(Boolean array=w2200) -> (logical OR=w2199:bool)
            n826 = Or(x=w2198, y=w2199) -> (x .or. y?=w2196:bool)
            n827 = event-data("Discard?"=w2196) -> ()  [unwired: 1 in, 1 out]
          }
          event Panel Close? {
            n828 = event-data() -> ("VIRef"=w2206:refnum<vi>)  [unwired: 1 in, 3 out]
            n829 = Close Reference(reference=w2206) -> ()  [unwired: 1 in, 1 out]
            n830 = disable-structure shown="Disabled" {
              frame Disabled {
                n831 = property on="Stop Button" class="Bool (strict)"("Val(Sgnl)"=TRUE ("Stop Button"), "Value"=FALSE ("Stop Button")) -> ()  [unwired: 2 in, 2 out]
              }
              frame Enabled {
              }
            }
            n832 = event-data("Discard?"=TRUE) -> ()  [unwired: 1 in, 1 out]
            "ClosePanel" <- TRUE ("ClosePanel")
          }
          event "Start": Value Change {
            w2232 = T16 [] items=["Auxiliary", "Temp Sens Cal", "Com Test", "Enable Test", "Speed Command", "Stop Time", "Temp Control", "Burn in", "Visual Inspec", "Empty"]
            n833 = event-data() -> ()  [unwired: 1 in, 2 out]
            n834 = property on="VISA Tester" class="VISAName"() -> ("Value"=w2230:refnum<visa-resource-name>)  [unwired: 2 in, 2 out]
            n835 = property on="UUT" class="Str"(error in=w2244) -> (error out=w2226:errorcluster, "Value"=w2243:string)  [unwired: 1 in, 1 out]
            n836 = control-ref of="Pannel User Message"() -> (w2223:refnum<vi>)
            n837 = control-ref of="Motor Speed RPM"() -> (w2218:refnum<vi>)
            n838 = call "TesterOption (SubVI).vi"("2 Options"=FALSE, "error in (no error)"=w2226, "On/Off"=FALSE, "Tester Option"=T11."Venable", "VISA Refnum in"=w2230) -> ("error out"=w2225:errorcluster)  [unwired: 5 in, 1 out]
            n839 = control-ref of="Stop Burn-in"() -> (w2221:refnum<vi>)
            n840 = control-ref of="Stop Button"() -> (w2222:refnum<vi>)
            n841 = call "Write panel message (SubVI).vi"("Stop BurnIn"=w2221, 4:"rpm"=w2218, 5:"rpm"=FALSE ("rpm"), "PrintTime"=TRUE, "Stop"=w2222, "error in (no error)"=w2225, "Time to wait"=5.0, "Strin"="TESTER BIT TEST OPERATION IN PROCESS", "String in"=w2223) -> ("error out"=w2224:errorcluster)  [unwired: 2 in]
            n842 = while {
              tunnel: w2243 -> [w2272]
              tunnel: [w2271] -> w2239
              tunnel: [w2270] -> w2238
              shift-right: [w2267] -> _
              shift-left: enum16{"Stop", "Tests", "Bit test", "Start"}."Start" -> [w2269]
              tunnel: w2233 -> [w2268]
              tunnel: w2232 -> [w2266]
              tunnel: w2224 -> [w2251]
              tunnel: w2222 -> [w2260]
              tunnel: w2221 -> [w2259]
              tunnel: w2223 -> [w2258]
              tunnel: w2218 -> [w2257]
              tunnel: w2215 -> [w2250]
              stop <- w2265 stop-if-true
              n843 = property class="Clust (strict)"(reference=w2250, error in=w2251) -> ("Value"=w2253:T7)  [unwired: 2 out]
              n844 = Unbundle By Name(w2253) -> ("DevType"=w2255:T2, "CanIndex"=w2254:T1)
              n845 = property on="VISA Tester" class="VISAName"() -> ("Value"=w2263:refnum<visa-resource-name>)  [unwired: 2 in, 2 out]
              n846 = call "VCI_Receive.vi"("CANIndex"=w2254, "DevIndex"=u32 0, "DevType"=w2255) -> ("Recieve"=w2256:T26[])  [unwired: 3 in, 5 out]
              n847 = Empty Array?(array=w2256) -> (empty?=w2249:bool)
              n848 = Not(x=w2249) -> (.not. x?=w2248:bool)
              n849 = property on="CAN Status" class="Bool (strict)"("Value"=w2248) -> (error out=w2247:errorcluster)  [unwired: 2 in, 1 out]
              n850 = property on="CAN Status" class="Bool (strict)"(error in=w2247) -> (error out=w2246:errorcluster, "Value"=w2261:bool)  [unwired: 1 in, 1 out]
              n851 = property on="Status" class="Bool (strict)"(error in=w2246) -> (error out=w2262:errorcluster, "Value"=w2264:bool)  [unwired: 1 in, 1 out]
              n852 = case shown="\"Start\"" w2269 {
                tunnel: w2272 -> [_ w2287 w2397 _]
                tunnel: [w2277 w2286 w2432 w2538] -> w2271
                tunnel: [w2273 w2285 w2395 w2530] -> w2270
                tunnel: w2268 -> [_ _ w2413 w2543]
                tunnel: w2258 -> [_ _ _ w2542]
                tunnel: w2260 -> [_ _ _ w2541]
                tunnel: w2259 -> [_ _ _ w2540]
                tunnel: w2257 -> [_ _ _ w2539]
                tunnel: [w2276 w2284 w2400 w2534] -> w2267
                tunnel: w2266 -> [w2277 _ w2432 w2538]
                tunnel: [w2275 w2283 FALSE FALSE] -> w2265
                tunnel: w2264 -> [_ _ _ w2536]
                tunnel: w2263 -> [_ _ w2414 _]
                tunnel: w2262 -> [w2273 _ _ _]
                tunnel: w2261 -> [_ _ _ w2531]
                frame "Stop", Default {
                  n853 = property on="Start" class="Bool (strict)"(error in=w2273, "Value"=FALSE ("Start")) -> ()  [unwired: 1 in, 2 out]
                  n854 = flat-sequence {
                    tunnel: [enum16{"Stop", "Tests", "Bit test", "Start"}."Stop"] -> w2276
                    tunnel: w2273 -> [_]
                    tunnel: [TRUE] -> w2275
                    frame #0 {
                    }
                  }
                }
                frame "Tests" {
                  w2280 = FALSE ("Stop Burn-in")
                  w2282 = T20."Disabled and Grayed Out" ("Disabled")
                  n855 = case shown="\"AHU\", Default" w2287 {
                    tunnel: [w2302 w2351] -> w2286
                    tunnel: [w2301 w2350] -> w2285
                    tunnel: [w2290 w2338] -> w2281
                    frame "AHU", Default {
                      n856 = call "Load Program Process AHU.vi"() -> ("Speed Command Test"=w2295:bool, "Enable Test"=w2296:bool, "Burn-in Test"=w2293:bool, "Auxiliary"=w2291:bool, "Temperature Sensor Calibration Test"=w2298:bool, "Communication Test"=w2297:bool, "Stop Time Test"=w2294:bool, "Visual Inspection"=w2292:bool, "OK"=w2299:bool, "Automation"=w2290:bool, "error out"=w2301:errorcluster)  [unwired: 8 in, 9 out]
                      n857 = Or(x=w2299, y=w2290) -> (x .or. y?=w2300:bool)
                      n858 = case shown="True" w2300 {
                        tunnel: [w2303 w2313] -> w2302
                        tunnel: w2290 -> [_ w2312]
                        tunnel: w2298 -> [_ w2311]
                        tunnel: w2297 -> [_ w2310]
                        tunnel: w2296 -> [_ w2309]
                        tunnel: w2295 -> [_ w2308]
                        tunnel: w2294 -> [_ w2307]
                        tunnel: w2293 -> [_ w2306]
                        tunnel: w2292 -> [_ w2305]
                        tunnel: w2291 -> [_ w2304]
                        frame False {
                          w2303 = T16 [] items=["Auxiliary", "Temp Sens Cal", "Com Test", "Enable Test", "Speed Command", "Stop Time", "Temp Control", "Burn in", "Visual Inspec", "Empty"]
                        }
                        frame True {
                          n859 = case shown="False" w2312 {
                            tunnel: [w2336 w2337] -> w2313
                            tunnel: w2311 -> [w2318 _]
                            tunnel: w2310 -> [w2317 _]
                            tunnel: w2309 -> [w2319 _]
                            tunnel: w2308 -> [w2316 _]
                            tunnel: w2307 -> [w2315 _]
                            tunnel: w2306 -> [w2329 _]
                            tunnel: w2305 -> [w2314 _]
                            tunnel: w2304 -> [_ _]
                            frame False {
                              w2322 = T24."Empty" ("f")
                              n860 = Select(t=T24."Com Test" ("f"), s=w2317, f=w2322) -> (s? t:f=w2328:T24)
                              n861 = Select(t=T24."Temp Sens Cal" ("f"), s=w2318, f=w2322) -> (s? t:f=w2327:T24)
                              n862 = Select(t=T24."Stop Time" ("f"), s=w2315, f=w2322) -> (s? t:f=w2326:T24)
                              n863 = Select(t=T24."Enable Test" ("f"), s=w2319, f=w2322) -> (s? t:f=w2325:T24)
                              n864 = Select(t=T24."Speed Command" ("f"), s=w2316, f=w2322) -> (s? t:f=w2324:T24)
                              n865 = Select(t=T24."Burn in" ("f"), s=w2329, f=w2322) -> (s? t:f=w2323:T24)
                              n866 = Select(t=T24."Visual Inspec" ("f"), s=w2314, f=w2322) -> (s? t:f=w2320:T24)
                              n867 = Build Array(w2328, w2327, w2326, w2325, w2324, w2323, w2320) -> (w2336:T16)
                            }
                            frame True {
                              w2337 = T16 [enum."Com Test", enum."Temp Sens Cal", enum."Stop Time", enum."Enable Test", enum."Speed Command", enum."Burn in", enum."Visual Inspec"] items=["Auxiliary", "Temp Sens Cal", "Com Test", "Enable Test", "Speed Command", "Stop Time", "Temp Control", "Burn in", "Visual Inspec", "Empty"]
                            }
                          }
                        }
                      }
                    }
                    frame "EBAY" {
                      n868 = call "Load Program Process EBAY.vi"() -> ("Speed Command Test"=w2344:bool, "Enable Test"=w2345:bool, "Burn-in Test"=w2342:bool, "Temperature Control Algorithm Test"=w2341:bool, "Auxiliary"=w2339:bool, "Temperature Sensor Calibration Test"=w2347:bool, "Communication Test"=w2346:bool, "Stop Time Test"=w2343:bool, "Visual Inspection"=w2340:bool, "OK"=w2348:bool, "Automation"=w2338:bool, "error out"=w2350:errorcluster)  [unwired: 8 in, 8 out]
                      n869 = Or(x=w2348, y=w2338) -> (x .or. y?=w2349:bool)
                      n870 = case shown="True" w2349 {
                        tunnel: [w2352 w2363] -> w2351
                        tunnel: w2338 -> [_ w2362]
                        tunnel: w2347 -> [_ w2361]
                        tunnel: w2346 -> [_ w2360]
                        tunnel: w2345 -> [_ w2359]
                        tunnel: w2344 -> [_ w2358]
                        tunnel: w2343 -> [_ w2357]
                        tunnel: w2342 -> [_ w2356]
                        tunnel: w2341 -> [_ w2355]
                        tunnel: w2340 -> [_ w2354]
                        tunnel: w2339 -> [_ w2353]
                        frame False {
                          w2352 = T16 [] items=["Auxiliary", "Temp Sens Cal", "Com Test", "Enable Test", "Speed Command", "Stop Time", "Temp Control", "Burn in", "Visual Inspec", "Empty"]
                        }
                        frame True {
                          n871 = case shown="False" w2362 {
                            tunnel: [w2392 w2393] -> w2363
                            tunnel: w2361 -> [w2368 _]
                            tunnel: w2360 -> [w2367 _]
                            tunnel: w2359 -> [w2366 _]
                            tunnel: w2358 -> [w2365 _]
                            tunnel: w2357 -> [w2364 _]
                            tunnel: w2356 -> [w2370 _]
                            tunnel: w2355 -> [w2369 _]
                            tunnel: w2354 -> [w2383 _]
                            tunnel: w2353 -> [w2374 _]
                            frame False {
                              w2372 = T24."Empty" ("f")
                              n872 = Select(t=T24."Com Test" ("f"), s=w2367, f=w2372) -> (s? t:f=w2382:T24)
                              n873 = Select(t=T24."Temp Sens Cal" ("f"), s=w2368, f=w2372) -> (s? t:f=w2381:T24)
                              n874 = Select(t=T24."Stop Time" ("f"), s=w2364, f=w2372) -> (s? t:f=w2380:T24)
                              n875 = Select(t=T24."Enable Test" ("f"), s=w2366, f=w2372) -> (s? t:f=w2379:T24)
                              n876 = Select(t=T24."Speed Command" ("f"), s=w2365, f=w2372) -> (s? t:f=w2378:T24)
                              n877 = Select(t=T24."Temp Control" ("f"), s=w2369, f=w2372) -> (s? t:f=w2377:T24)
                              n878 = Select(t=T24."Burn in" ("f"), s=w2370, f=w2372) -> (s? t:f=w2376:T24)
                              n879 = Select(t=T24."Visual Inspec" ("f"), s=w2383, f=w2372) -> (s? t:f=w2375:T24)
                              n880 = Select(t=T24."Auxiliary" ("f"), s=w2374, f=w2372) -> (s? t:f=w2371:T24)
                              n881 = Build Array(w2382, w2381, w2380, w2379, w2378, w2377, w2376, w2371, w2375) -> (w2392:T16)
                            }
                            frame True {
                              w2393 = T16 [enum."Com Test", enum."Temp Sens Cal", enum."Stop Time", enum."Enable Test", enum."Speed Command", enum."Temp Control", enum."Burn in", enum."Auxiliary", enum."Visual Inspec"] items=["Auxiliary", "Temp Sens Cal", "Com Test", "Enable Test", "Speed Command", "Stop Time", "Temp Control", "Burn in", "Visual Inspec", "Empty"]
                            }
                          }
                        }
                      }
                    }
                  }
                  "Automation" <- w2281
                  n882 = flat-sequence {
                    tunnel: [enum16{"Stop", "Tests", "Bit test", "Start"}."Tests"] -> w2284
                    tunnel: [TRUE] -> w2283
                    frame #0 {
                    }
                  }
                  n883 = property on="Stop Button" class="Bool (strict)"("Value"=w2280) -> ()  [unwired: 2 in, 2 out]
                  n884 = property on="Stop Burn-in" class="Bool (strict)"("Value"=w2280) -> ()  [unwired: 2 in, 2 out]
                  n885 = property on="Start" class="Bool (strict)"("DisabledEnum"=w2282) -> ()  [unwired: 2 in, 2 out]
                  n886 = property on="Report" class="Bool (strict)"("DisabledEnum"=w2282) -> ()  [unwired: 2 in, 2 out]
                }
                frame "Bit test" {
                  # "Stop"
                  n887 = call "SerialMarvinSendGet.vi"("write buffer"="TA[1]\r\n", "VISA resource name"=w2413) -> ("error out"=w2426:errorcluster, "read buffer"=w2429:string)  [unwired: 8 in]
                  n888 = Fract/Exp String To Number(string=w2429) -> (number=w2428:dbl)  [unwired: 3 in, 1 out]
                  n889 = Less Or Equal?(x=w2428, y=100.0) -> (x <= y?=w2411:bool)
                  n890 = call "TesterOption (SubVI).vi"("On/Off 2"=FALSE, "Tester Option 2"=T11."Venable", "2 Options"=TRUE, "error in (no error)"=w2426, "On/Off"=TRUE, "Tester Option"=T11."25C", "VISA Refnum in"=w2414) -> ("error out"=w2416:errorcluster)  [unwired: 3 in, 1 out]
                  n891 = call "Time Delay5"("error in (no error)"=w2416) -> ("error out"=w2415:errorcluster)  [unwired: 10 in]
                  n892 = call "SerialMarvinSendGet.vi"("error in (no error)"=w2415, "write buffer"="TA[2]\r\n", "VISA resource name"=w2413) -> ("error out"=w2412:errorcluster, "read buffer"=w2418:string)  [unwired: 7 in]
                  n893 = case shown="\"EBAY\"" w2397 {
                    tunnel: w2414 -> [w2462 _ w2490]
                    tunnel: w2413 -> [_ _ w2493]
                    tunnel: w2412 -> [w2463 w2481 w2492]
                    tunnel: [w2456 w2481 w2488] -> w2399
                    tunnel: [w2453 "" w2483] -> w2406
                    tunnel: [w2452 bool[] [] w2482] -> w2404
                    frame "AHU" {
                      n894 = call "TesterOption (SubVI).vi"("On/Off 2"=FALSE, "Tester Option 2"=T11."Venable", "2 Options"=TRUE, "error in (no error)"=w2463, "On/Off"=TRUE, "Tester Option"=T11."K17", "VISA Refnum in"=w2462) -> ("error out"=w2465:errorcluster)  [unwired: 3 in, 1 out]
                      n895 = call "Time Delay7"("error in (no error)"=w2465) -> ("error out"=w2464:errorcluster)  [unwired: 10 in]
                      n896 = call "GetADCTester (SubVI).vi"("error in (no error)"=w2464, "GetADCTester"=T13."Current", "TimeToGet"=5, "VISA Refnum in"=w2462) -> ("error out"=w2456:errorcluster, "ADCValOutput Single"=w2458:dbl)  [unwired: 5 in, 1 out]
                      n897 = Less Or Equal?(x=w2458, y=50.0) -> (x <= y?=w2457:bool)
                      n898 = Build Array(w2457) -> (w2452:bool[])
                      n899 = for {
                        tunnel: w2452 -> [w2478] mode=indexing
                        tunnel: string[] ["CURRENT OPERATION FAILED!"] -> [w2474] mode=indexing
                        shift-right: [w2476] -> w2453
                        shift-left: "" -> [w2475]
                        n900 = Concatenate Strings(w2474, "  TEST FAILED!" ("string"), "\r\n") -> (w2471:string)
                        n901 = Select(t=w2471, s=w2478, f=w2475) -> (s? t:f=w2477:string)
                        n902 = Concatenate Strings(w2475, w2477) -> (w2476:string)
                      }
                    }
                    frame Default {
                    }
                    frame "EBAY" {
                      w2491 = T30 [enum."Fan", enum."Current"] items=["Term1", "Term2", "Current", "Fan", "TempCPU"]
                      n903 = call "TesterOption (SubVI).vi"("On/Off 2"=FALSE, "Tester Option 2"=T11."Venable", "2 Options"=TRUE, "error in (no error)"=w2492, "On/Off"=TRUE, "Tester Option"=T11."K17", "VISA Refnum in"=w2490) -> ("error out"=w2495:errorcluster)  [unwired: 3 in, 1 out]
                      n904 = call "Time Delay6"("error in (no error)"=w2495) -> ("error out"=w2494:errorcluster)  [unwired: 10 in]
                      n905 = call "SerialMarvinSendGet.vi"("error in (no error)"=w2494, "write buffer"="TA[3]\r\n", "VISA resource name"=w2493) -> ("error out"=w2489:errorcluster, "read buffer"=w2497:string)  [unwired: 7 in]
                      n906 = Fract/Exp String To Number(string=w2497) -> (number=w2498:dbl)  [unwired: 3 in, 1 out]
                      n907 = for {
                        tunnel: w2491 -> [w2522] mode=indexing
                        tunnel: w2490 -> [w2521]
                        tunnel: w2489 -> [w2519]
                        tunnel: [w2518] -> w2488
                        tunnel: [w2515] -> w2486 mode=indexing
                        i -> [w2516]
                        n908 = call "GetADCTester (SubVI).vi"("error in (no error)"=w2519, "GetADCTester"=w2522, "TimeToGet"=0, "VISA Refnum in"=w2521) -> ("error out"=w2518:errorcluster, "ADCValOutput Single"=w2517:dbl)  [unwired: 5 in, 1 out]
                        n909 = case shown="1" w2516 {
                          tunnel: w2517 -> [w2525 w2528 _]
                          tunnel: [w2523 w2526 FALSE] -> w2515
                          frame 1 {
                            n910 = Less Or Equal?(x=w2525, y=50.0) -> (x <= y?=w2523:bool)
                          }
                          frame 0 {
                            n911 = Greater Or Equal?(x=w2528, y=2200.0) -> (x >= y?=w2526:bool)
                          }
                          frame Default {
                          }
                        }
                      }
                      n912 = Less Or Equal?(x=w2498, y=100.0) -> (x <= y?=w2487:bool)
                      n913 = Build Array (concatenate)(w2487, w2486) -> (w2482:bool[])
                      n914 = for {
                        tunnel: w2482 -> [w2505] mode=indexing
                        tunnel: string[] ["TA[3] OPERATION FAILED!", "EBAY FAN OPERATION FAILED!", "CURRENT OPERATION FAILED!"] -> [w2508] mode=indexing
                        shift-right: [w2510] -> w2483
                        shift-left: "" -> [w2509]
                        n915 = Concatenate Strings(w2508, "\r\n") -> (w2506:string)
                        n916 = case shown="False" w2505 {
                          tunnel: [w2513 w2514] -> w2510
                          tunnel: w2509 -> [w2512 w2514]
                          tunnel: w2506 -> [w2511 _]
                          frame False {
                            n917 = Concatenate Strings(w2512, w2511) -> (w2513:string)
                          }
                          frame True {
                          }
                        }
                      }
                    }
                  }
                  n918 = Fract/Exp String To Number(string=w2418) -> (number=w2419:dbl)  [unwired: 3 in, 1 out]
                  n919 = Less Or Equal?(x=w2419, y=100.0) -> (x <= y?=w2410:bool)
                  n920 = Build Array(w2411, w2410) -> (w2405:bool[])
                  n921 = for {
                    tunnel: w2405 -> [w2441] mode=indexing
                    tunnel: string[] ["TA[1] OPERATION FAILED!", "TA[2] OPERATION FAILED!"] -> [w2445] mode=indexing
                    shift-right: [w2447] -> w2407
                    shift-left: "" -> [w2446]
                    tunnel: w2399 -> [w2442]
                    tunnel: [w2442] -> w2398
                    n922 = Concatenate Strings(w2445, "\r\n") -> (w2443:string)
                    n923 = case shown="False" w2441 {
                      tunnel: [w2450 w2451] -> w2447
                      tunnel: w2446 -> [w2449 w2451]
                      tunnel: w2443 -> [w2448 _]
                      frame False {
                        n924 = Concatenate Strings(w2449, w2448) -> (w2450:string)
                      }
                      frame True {
                      }
                    }
                  }
                  n925 = Build Array (concatenate)(w2405, w2404) -> (w2403:bool[])
                  n926 = And Array Elements(Boolean array=w2403) -> (logical AND=w2394:bool)
                  n927 = case shown="False" w2394 {
                    tunnel: w2407 -> [w2439 _]
                    tunnel: w2406 -> [w2438 _]
                    tunnel: w2398 -> [w2436 w2440]
                    tunnel: [w2436 w2440] -> w2396
                    frame False {
                      n928 = Concatenate Strings(w2439, w2438) -> (w2437:string)
                      n929 = One Button Dialog(message=w2437) -> ()  [unwired: 1 in, 1 out]
                    }
                    frame True {
                    }
                  }
                  n930 = case shown="False" w2394 {
                    tunnel: w2396 -> [w2434 w2435]
                    tunnel: [w2433 w2435] -> w2395
                    frame False {
                      n931 = call "Display Message to User6"("error in (no error)"=w2434) -> ("error out"=w2433:errorcluster)  [unwired: 9 in, 1 out]
                    }
                    frame True {
                    }
                  }
                  n932 = Select(t=enum16{"Stop", "Tests", "Bit test", "Start"}."Tests", s=w2394, f=enum16{"Stop", "Tests", "Bit test", "Start"}."Stop") -> (s? t:f=w2400:enum16{"Stop", "Tests", "Bit test", "Start"})
                }
                frame "Start" {
                  n933 = And(x=w2531, y=w2536) -> (x .and. y?=w2532:bool)
                  n934 = case shown="True" w2532 {
                    tunnel: w2543 -> [_ w2570]
                    tunnel: w2542 -> [_ w2561]
                    tunnel: w2541 -> [_ w2557]
                    tunnel: w2540 -> [_ w2555]
                    tunnel: w2539 -> [_ w2554]
                    tunnel: [FALSE w2553] -> w2535
                    tunnel: [w2549 w2552] -> w2530
                    tunnel: [FALSE TRUE] -> w2533
                    frame False {
                      n935 = call "Display Message to User5"() -> ("error out"=w2549:errorcluster)  [unwired: 10 in, 1 out]
                    }
                    frame True {
                      n936 = property on="VISA Tester" class="VISAName"() -> (error out=w2568:errorcluster, "Value"=w2567:refnum<visa-resource-name>)  [unwired: 2 in, 1 out]
                      n937 = call "TesterOption (SubVI).vi"("2 Options"=FALSE, "error in (no error)"=w2568, "On/Off"=FALSE, "Tester Option"=T11."Venable", "VISA Refnum in"=w2567) -> ("error out"=w2563:errorcluster)  [unwired: 5 in, 1 out]
                      n938 = call "Write panel message (SubVI).vi"("Stop BurnIn"=w2555, 4:"rpm"=w2554, 5:"rpm"=FALSE ("rpm"), "PrintTime"=FALSE, "Stop"=w2557, "error in (no error)"=w2563, "Time to wait"=3.0, "Strin"="TESTER BIT TEST OPERATION IN PROCESS\nPlease wait...", "String in"=w2561) -> ("error out"=w2562:errorcluster)  [unwired: 2 in]
                      n939 = property on="UUT SoftwareVer" class="Str"() -> ("Value"=w2551:string)  [unwired: 2 in, 2 out]
                      n940 = call "SerialMarvinSendGet.vi"("error in (no error)"=w2562, "write buffer"="VR\r\n", "VISA resource name"=w2570) -> ("error out"=w2552:errorcluster, "read buffer"=w2569:string)  [unwired: 7 in]
                      n941 = Equal?(x=w2569, y=w2551) -> (x = y?=w2553:bool)
                    }
                  }
                  n942 = case shown="False" w2535 {
                    tunnel: [enum16{"Stop", "Tests", "Bit test", "Start"}."Stop" enum16{"Stop", "Tests", "Bit test", "Start"}."Bit test"] -> w2534
                    tunnel: w2533 -> [w2544 _]
                    frame False {
                      n943 = case shown="True" w2544 {
                        frame False {
                        }
                        frame True {
                          n944 = call "Display Message to User4"() -> ()  [unwired: 10 in, 2 out]
                        }
                      }
                    }
                    frame True {
                    }
                  }
                }
              }
            }
            n945 = Bundle By Name(cluster=T8 {"VISA"="COM1", "Array Test"=[]}, "VISA"=w2233, "Array Test"=w2239) -> (w2235:T8)
            n946 = Enqueue Element(queue=w2241, element=w2235, error in (no error)=w2238) -> (queue out=w2236:refnum<queue>, error out=w2237:errorcluster)  [unwired: 2 out]
          }
          event "Report", "Stop Button": Value Change {
            w2608 = "Marvin" ("section")
            n947 = event-data() -> ("CtlRef"=w2594:refnum<vi>)  [unwired: 1 in]
            n948 = local read "UUT"() -> (w2604:string)
            n949 = call <vilib>:"Application Directory.vi"() -> ("Application Directory"=w2636:path)
            n950 = Build Path(base path=w2636, name or relative path="Reports") -> (appended path=w2639:path)
            n951 = property on="CAN Status" class="Bool (strict)"() -> ("Value"=w2572:bool)  [unwired: 2 in, 2 out]
            n952 = property on="Status" class="Bool (strict)"() -> ("Value"=w2573:bool)  [unwired: 2 in, 2 out]
            n953 = case shown="\"EBAY\", Default" w2604 {
              tunnel: ["REV EBAY" ("key") "REV AHU" ("key")] -> w2606
              frame "EBAY", Default {
              }
              frame "AHU" {
              }
            }
            n954 = call <vilib>:"Check if File or Folder Exists.vi"("path"=w2639) -> ("error out"=w2637:errorcluster, "file or folder exists?"=w2640:bool, "dup path"=w2638:path)  [unwired: 8 in]
            n955 = And(x=w2573, y=w2572) -> (x .and. y?=w2574:bool)
            n956 = case shown="False" w2640 {
              tunnel: w2637 -> [w2706 w2707]
              tunnel: w2638 -> [w2705 w2708]
              tunnel: [w2704 w2708] -> w2645
              tunnel: [w2703 w2707] -> w2642
              frame False {
                n957 = Create Folder(path (use dialog)=w2705, error in=w2706) -> (created path=w2704:path, error out=w2703:errorcluster)  [unwired: 1 in, 1 out]
              }
              frame True {
              }
            }
            n958 = case shown="True" w2574 {
              tunnel: [w2652 w2671] -> w2625
              tunnel: [w2652 w2670] -> w2603
              tunnel: w2598 -> [_ w2658]
              tunnel: [w2652 w2663] -> w2595
              tunnel: [w2652 w2662] -> w2597
              tunnel: [w2652 w2666] -> w2588
              tunnel: [w2652 w2665] -> w2580
              frame False {
                (unwired) "47"
                (unwired) " 413-8005_47_AHU"
                (unwired) "413-8005-1-47"
                (unwired) "5.3.9" ("read buffer")
                (unwired) "95"
                (unwired) "414-8005_95_EBAY_"
                (unwired) "414-8005-95"
                (unwired) "414-8005-95   "
                w2652 = "N_A" ("read buffer")
                n959 = disable-structure shown="Disabled" {
                  frame Disabled {
                    n960 = call "Display Message to User7"() -> ()  [unwired: 10 in, 2 out]
                  }
                  frame Enabled {
                  }
                }
                n961 = Decimal String To Number(string="1" ("Value")) -> (number=w2653:i32)  [unwired: 2 in, 1 out]
                n962 = Number To Decimal String(number=w2653, width (-)=i16 4) -> ()  [unwired: 1 out]
              }
              frame True {
                n963 = call "SerialMarvinSendGet.vi"("write buffer"="SN\r\n", "VISA resource name"=w2658) -> ("error out"=w2657:errorcluster, "read buffer"=w2660:string)  [unwired: 8 in]
                n964 = call "Time Delay2"("error in (no error)"=w2657) -> ("error out"=w2656:errorcluster)  [unwired: 10 in]
                n965 = Decimal String To Number(string=w2660) -> (number=w2659:i32)  [unwired: 2 in, 1 out]
                n966 = Number To Decimal String(number=w2659, width (-)=i16 4) -> (decimal integer string=w2663:string)
                n967 = call "SerialMarvinSendGet.vi"("error in (no error)"=w2656, "write buffer"="VR\r\n", "VISA resource name"=w2658) -> ("error out"=w2667:errorcluster, "read buffer"=w2662:string)  [unwired: 7 in]
                n968 = property on="UUT" class="DigNum (strict)"(error in=w2667) -> ("Value"=w2669:u8)  [unwired: 1 in, 2 out]
                n969 = case shown="95, Default" w2669 {
                  tunnel: ["414-8005_95_EBAY_" " 413-8005_47_AHU" " 413-8005_63_AHU"] -> w2671
                  tunnel: ["414-8005-95   " w2677 w2680] -> w2670
                  tunnel: ["414-8005-95" w2677 w2680] -> w2666
                  tunnel: ["95" "47" "63"] -> w2665
                  frame 95, Default {
                  }
                  frame 47 {
                    w2677 = "413-8005-1-47"
                    (unwired) "AHU-L (47) 413-8005-1"
                  }
                  frame 63 {
                    w2680 = "413-8005-2-63"
                    (unwired) "AHU-R (63) 413-8005-2"
                  }
                }
              }
            }
            n970 = Get Date/Time String(want seconds? (F)=TRUE) -> (date string=w2641:string)  [unwired: 2 in, 1 out]
            n971 = call <vilib>:"Open Config Data.vi"("create file if necessary (T)"=FALSE, "configuration file path"=w2600) -> ("refnum"=w2615:T18)  [unwired: 1 in, 8 out]
            n972 = property on="Logger Path" class="Path"(error in=w2642, "Value"=w2645, "StartPath"=w2645) -> (error out=w2643:errorcluster)  [unwired: 1 in, 1 out]
            n973 = Search and Replace String(replace all?=TRUE ("replace all? (F)"), input string=w2641, search string="/") -> (result string=w2622:string)  [unwired: 5 in, 3 out]
            n974 = call-poly <vilib>:"Read Key.vi"("section"=w2608, "key"=w2606, "refnum"=w2615) -> ("error out"=w2610:errorcluster, "value"=w2613:string, "refnum out"=w2612:T18)  [unwired: 5 in, 1 out]
            n975 = property on="Logger Path" class="Path"(error in=w2643) -> (error out=w2618:errorcluster, "StartPath"=w2621:path)  [unwired: 1 in, 1 out]
            n976 = call-poly <vilib>:"Read Key.vi"("section"=w2608, "error in (no error)"=w2610, "key"="Tester Software Ver", "refnum"=w2612) -> ("error out"=w2607:errorcluster, "value"=w2605:string, "refnum out"=w2611:T18)  [unwired: 4 in, 1 out]
            n977 = Concatenate Strings("ATR" ("string"), w2625, w2595, "_", w2622, ".docx" ("string")) -> (w2619:string)
            n978 = call <vilib>:"Close Config Data.vi"("error in (no error)"=w2607, "refnum"=w2611) -> ()  [unwired: 8 in, 2 out]
            n979 = Build Path(base path=w2621, name or relative path=w2619) -> (appended path=w2620:path)
            n980 = call "HeaderuRayon.vi"("Oper."=w2596, "VR"=w2597, "S/N"=w2595, "UUT"=w2603, "UA"=w2580, "UUTHeader"=w2604, "Tester Software Ver"=w2605) -> ("HEADER1"=w2646:string)  [unwired: 1 in]
            n981 = Concatenate Strings("  Rev-" ("string"), w2613) -> (w2599:string)
            n982 = while {
              tunnel: w2619 -> [w2688]
              tunnel: w2621 -> [w2685]
              shift-right: [w2687] -> w2617
              shift-left: w2620 -> [w2686]
              shift-right: [w2683] -> w2601
              shift-left: w2602 -> [w2684]
              tunnel: w2618 -> [w2689]
              tunnel: [w2690] -> _
              stop <- w2682 continue-if-true
              n983 = call <vilib>:"Check if File or Folder Exists.vi"("error in (no error)"=w2689, "path"=w2686) -> ("error out"=w2690:errorcluster, "file or folder exists?"=w2682:bool)  [unwired: 7 in, 1 out]
              n984 = case shown="True" w2682 {
                tunnel: w2688 -> [_ w2702]
                tunnel: w2684 -> [_ w2694]
                tunnel: [w2692 w2699] -> w2687
                tunnel: w2686 -> [w2692 _]
                tunnel: w2685 -> [_ w2700]
                tunnel: [1 w2693] -> w2683
                frame False {
                }
                frame True {
                  w2695 = ".docx" ("search string")
                  n985 = Search and Replace String(input string=w2702, search string=w2695) -> (result string=w2701:string)  [unwired: 6 in, 3 out]
                  n986 = Number To Decimal String(number=w2694) -> (decimal integer string=w2697:string)  [unwired: 1 in]
                  n987 = call <vilib>:"Space Constant.vi"() -> ("String"=w2696:string)
                  n988 = Concatenate Strings(w2701, w2696, w2697, w2695) -> (w2698:string)
                  n989 = Build Path(base path=w2700, name or relative path=w2698) -> (appended path=w2699:path)
                  n990 = Increment(x=w2694) -> (x+1=w2693:i32)
                }
              }
            }
            n991 = Open/Create/Replace File(file path (use dialog)=w2617, operation (0:open)=T25."create") -> (error out=w2631:errorcluster)  [unwired: 4 in, 2 out]
            n992 = control-ref of="ATR"() -> (w2647:refnum<vi>)
            n993 = property class="Tbl (strict)"(reference=w2647, error in=w2631) -> ("Value"=w2648:string[][])  [unwired: 2 out]
            n994 = call "MarvinReport.vi"("HEADER1"=w2646, "ATR Or"=w2647, "Steps   pfull"=w2648, "Footer UUT"=w2588, "pageNum"=3, "FILE NAME"=w2619, "Report Folder"=w2617, "REV"=w2599, "Test-Conductor"=w2596) -> ("error out"=w2583:errorcluster)  [unwired: 5 in, 1 out]
            n995 = call <vilib>:"Clear Errors.vi"("error in (no error)"=w2583) -> ("error out"=w2582:errorcluster)  [unwired: 5 in, 1 out]
            n996 = property class="Bool (strict)"(reference=w2594, error in=w2582) -> ("BoolText.Text"=w2593:string)  [unwired: 2 out]
            n997 = Equal?(x=w2593, y="Report") -> (x = y?=w2587:bool)
            n998 = Select(t=T10."MainProgram", s=w2587, f=T10."Stop") -> (s? t:f=w2590:T10)
            n999 = Select(t="Save Report...", s=w2587, f="Program Stopped...\r\nPlease turn OFF All Power sinks") -> (s? t:f=w2585:string)
            n1000 = property on="Report" class="Bool (strict)"(error in=w2582, "Value"=FALSE ("Report")) -> (error out=w2575:errorcluster)  [unwired: 1 in, 1 out]
            n1001 = property on="VISA Tester" class="VISAName"() -> ("Value"=w2579:refnum<visa-resource-name>)  [unwired: 2 in, 2 out]
            n1002 = property on="Pannel User Message" class="Str"("Value"=w2585) -> ()  [unwired: 2 in, 2 out]
            n1003 = call "TesterOption (SubVI).vi"("2 Options"=FALSE, "error in (no error)"=w2575, "On/Off"=FALSE, "Tester Option"=T11."Venable", "VISA Refnum in"=w2579) -> ()  [unwired: 5 in, 2 out]
          }
          event "Help Button": Value Change {
            n1004 = event-data() -> ()  [unwired: 1 in, 6 out]
            n1005 = vi-ref "Help.vi"() -> (w2718:refnum<vi>)
            n1006 = invoke class="VI" method="FP.Open"(reference=w2718, error in=w2716, "Activate"=TRUE ("Activate?"), "State"=T22."Standard") -> (error out=w2717:errorcluster)  [unwired: 1 in, 4 out]
            n1007 = call "Help.vi"("error in"=w2717) -> ("error out"=w2715:errorcluster)  [unwired: 7 in]
          }
          event "Serial Com": Value Change {
            n1008 = event-data() -> ()  [unwired: 1 in, 6 out]
            n1009 = property on="Serial Com" class="Bool"(error in=w2727, "Visible"=FALSE) -> (error out=w2731:errorcluster)  [unwired: 1 in, 1 out]
            n1010 = property on="VISA Marvin" class="VISAName"(error in=w2731, "Visible"=TRUE) -> (error out=w2728:errorcluster)  [unwired: 1 in, 1 out]
          }
          event "VISA Marvin": Value Change {
            n1011 = event-data() -> ()  [unwired: 1 in, 6 out]
            n1012 = property on="Serial Com" class="Bool"(error in=w2734, "Visible"=FALSE) -> (error out=w2733:errorcluster)  [unwired: 1 in, 1 out]
            n1013 = control-ref of="This VI"() -> (w2745:refnum<vi>)
            n1014 = property on="Pannel User Message" class="Str"(error in=w2734, "Value"="Serial connection in process" ("Pannel User Message")) -> ()  [unwired: 1 in, 2 out]
            n1015 = call "Serial InitMarvin.vi"("error in (no error)"=w2733, "VI reference (current VI)"=w2745, "VISA Refnum in"="VISA Marvin") -> ("error out"=w2737:errorcluster, "Boolean"=w2735:bool)  [unwired: 7 in]
            n1016 = property on="VISA Marvin" class="VISAName"(error in=w2737, "Visible"=FALSE) -> (error out=w2748:errorcluster)  [unwired: 1 in, 1 out]
            n1017 = property on="Serial Com" class="Bool"(error in=w2748, "Visible"=TRUE) -> (error out=w2744:errorcluster)  [unwired: 1 in, 1 out]
            n1018 = case shown="True" w2735 {
              tunnel: w2744 -> [w2751 w2763]
              tunnel: "VISA Marvin" -> [w2752 w2760]
              tunnel: [w2752 w2759] -> w2739
              tunnel: [w2751 w2758] -> w2738
              frame False {
              }
              frame True {
                n1019 = call "SerialMarvinSendGet.vi"("error in (no error)"=w2763, "Clear Log"=FALSE, "write buffer"="VC\r\n", "VISA resource name"=w2760) -> ("error out"=w2762:errorcluster, "read buffer"=w2756:string)  [unwired: 6 in]
                n1020 = Decimal String To Number(string=w2756) -> (number=w2755:i32)  [unwired: 2 in, 1 out]
                n1021 = Less Or Equal?(x=w2755, y=50) -> (x <= y?=w2753:bool)
                n1022 = property on="Status" class="Bool (strict)"("Value"=w2753) -> ()  [unwired: 2 in, 2 out]
                n1023 = case shown="True" w2753 {
                  tunnel: w2762 -> [w2764 w2788]
                  tunnel: w2760 -> [w2765 w2787]
                  tunnel: [w2765 w2778] -> w2759
                  tunnel: [w2764 w2772] -> w2758
                  frame False {
                  }
                  frame True {
                    n1024 = call <vilib>:"Clear Errors.vi"("error in (no error)"=w2788) -> ("error out"=w2789:errorcluster)  [unwired: 5 in, 1 out]
                    n1025 = control-ref of="ATR"() -> (w2775:refnum<vi>)
                    n1026 = VISA Flush I/O Buffer(VISA resource name=w2787, error in (no error)=w2789) -> (VISA resource name out=w2778:refnum<visa-resource-name>, error out=w2786:errorcluster)  [unwired: 1 in]
                    n1027 = call "Display Message to User2"("error in (no error)"=w2786) -> ("error out"=w2785:errorcluster, "Yes"=w2784:bool)  [unwired: 9 in]
                    n1028 = case shown="True" w2784 {
                      tunnel: w2785 -> [w2790 w2812]
                      tunnel: [w2790 w2791] -> w2783
                      tunnel: w2778 -> [_ w2809]
                      frame False {
                      }
                      frame True {
                        w2797 = FALSE ("2 Options")
                        n1029 = property on="UUT" class="DigNum (strict)"() -> ("Value"=w2811:u8)  [unwired: 2 in, 2 out]
                        n1030 = call "SetParam.vi"("RS"=TRUE, "error in (no error)"=w2812, "Param to Set in"=w2811, "Visa"=w2809) -> ("error out"=w2792:errorcluster)  [unwired: 7 in]
                        n1031 = control-ref of="Pannel User Message"() -> (w2808:refnum<vi>)
                        n1032 = control-ref of="Stop Burn-in"() -> (w2806:refnum<vi>)
                        n1033 = control-ref of="Stop Button"() -> (w2807:refnum<vi>)
                        n1034 = control-ref of="Motor Speed RPM"() -> (w2805:refnum<vi>)
                        n1035 = property on="VISA Tester" class="VISAName"() -> ("Value"=w2801:refnum<visa-resource-name>)  [unwired: 2 in, 2 out]
                        n1036 = call "TesterOption (SubVI).vi"("2 Options"=w2797, "error in (no error)"=w2792, "On/Off"=FALSE, "Tester Option"=T11."Power", "VISA Refnum in"=w2801) -> ("error out"=w2802:errorcluster, "VISA Refnum out"=w2804:refnum<visa-resource-name>)  [unwired: 5 in]
                        n1037 = call "Write panel message (SubVI).vi"("Stop BurnIn"=w2806, "rpm"=w2805, "PrintTime"=TRUE, "Stop"=w2807, "error in (no error)"=w2802, "Time to wait"=20.0, "Strin"="Restart the UUT\nPlease wait...", "String in"=w2808) -> ("error out"=w2803:errorcluster)  [unwired: 3 in]
                        n1038 = call "TesterOption (SubVI).vi"("2 Options"=w2797, "error in (no error)"=w2803, "On/Off"=FALSE, "Tester Option"=T11."Venable", "VISA Refnum in"=w2804) -> ("error out"=w2791:errorcluster)  [unwired: 5 in, 1 out]
                      }
                    }
                    n1039 = call "Find_Number_LineMARVIN.vi"("Test Paragraph"="2.1", "TableIn"=w2775) -> ("Line number"=w2776:i32)  [unwired: 3 in, 3 out]
                    n1040 = call "SerialMarvinSendGet.vi"("error in (no error)"=w2783, "write buffer"="SN\r\n", "VISA resource name"=w2778) -> ("error out"=w2779:errorcluster, "read buffer"=w2767:string)  [unwired: 7 in]
                    n1041 = call "SerialMarvinSendGet.vi"("error in (no error)"=w2779, "write buffer"="AO[1]\r\n", "VISA resource name"=w2778) -> ("error out"=w2773:errorcluster, "read buffer"=w2774:string)  [unwired: 7 in]
                    n1042 = Fract/Exp String To Number(string=w2774) -> (number=w2769:dbl)  [unwired: 3 in, 1 out]
                    n1043 = In Range and Coerce(upper limit=0.1 ("x"), x=w2769, lower limit=-0.1) -> (In Range?=w2768:bool)  [unwired: 1 out]
                    n1044 = call "PassOrFail (SubVI).vi"("Test#"="2", "index (row)"=w2776, "error in (no error)"=w2773, "Data in"=w2769, "Pass?Fail"=w2768, "Table in"=w2775) -> ("error out"=w2772:errorcluster)  [unwired: 5 in]
                    n1045 = property on="UUT SN Report" class="Str"("Value"=w2767) -> ()  [unwired: 2 in, 2 out]
                    n1046 = Decimal String To Number(string=w2767) -> (number=→"Current SN":i32)  [unwired: 2 in, 1 out]
                  }
                }
              }
            }
          }
          event "Refresh Button": Value Change {
            n1047 = event-data() -> ()  [unwired: 1 in, 6 out]
          }
          event "Settings": Value Change {
            n1048 = event-data() -> ()  [unwired: 1 in, 6 out]
            n1049 = control-ref of="VISA Tester"() -> (w2822:refnum<vi>)
            n1050 = control-ref of="UUT"() -> (w2820:refnum<vi>)
            n1051 = property on="Status" class="Bool (strict)"() -> ("Value"=w2824:bool)  [unwired: 2 in, 2 out]
            n1052 = case shown="True" w2824 {
              tunnel: w2830 -> [_ w2842]
              tunnel: [w2831 w2837] -> w2825
              tunnel: w2823 -> [_ w2836]
              tunnel: w2822 -> [_ w2835]
              tunnel: w2821 -> [_ w2834]
              tunnel: w2820 -> [_ w2833]
              frame False {
                n1053 = call "Display Message to User8"() -> ("error out"=w2831:errorcluster)  [unwired: 10 in, 1 out]
              }
              frame True {
                n1054 = vi-ref "Calibration (SubVI).vi"() -> (w2841:refnum<vi>)
                n1055 = invoke class="VI" method="FP.Open"(reference=w2841, error in=w2842, "Activate"=TRUE ("Activate?"), "State"=T22."Standard") -> (error out=w2838:errorcluster)  [unwired: 1 in, 4 out]
                n1056 = call "Calibration (SubVI).vi"("VISA UUT"=w2836, "error constant"=w2838, "UUT"=w2833, "CAN Cluster in"=w2834, "Visa Tester"=w2835) -> ("error constant 2"=w2837:errorcluster, "AO[1]Meas"=→"Cal":dbl)  [unwired: 5 in]
              }
            }
          }
        }
      }
      frame "Initialize" {
        w2846 = FALSE ("Visible")
        w2847 = FALSE ("Visible")
        w2848 = FALSE ("Visible")
        w2849 = FALSE ("Visible")
        w2861 = refnum<visa-resource-name> "COM1" ("VISA resource name")
        w2851 = FALSE ("Visible")
        w2844 = FALSE ("Serial Status")
        n1057 = property on="ComTestResult" class="Bool (strict)"("Value"=w2849) -> ()  [unwired: 2 in, 2 out]
        n1058 = property on="VenableResult" class="Bool (strict)"("Value"=w2849) -> ()  [unwired: 2 in, 2 out]
        n1059 = property on="VenableDirectionResult" class="Bool (strict)"("Value"=w2849) -> ()  [unwired: 2 in, 2 out]
        n1060 = property on="SpeedResult" class="Bool (strict)"("Value"=w2849) -> ()  [unwired: 2 in, 2 out]
        n1061 = property on="Serial Com" class="Bool"(error in=errorcluster {"status"=FALSE, "code"=0, "source"=""} ("error out"), "Visible"=TRUE) -> (error out=w2863:errorcluster)  [unwired: 1 in, 1 out]
        n1062 = property on="AuxiOFFResult" class="Bool (strict)"("Value"=w2848) -> ()  [unwired: 2 in, 2 out]
        n1063 = property on="AuxiONResult" class="Bool (strict)"("Value"=w2848) -> ()  [unwired: 2 in, 2 out]
        n1064 = property on="VisualInspectionResult" class="Bool (strict)"("Value"=w2848) -> ()  [unwired: 2 in, 2 out]
        n1065 = property on="SensCalResult" class="Bool (strict)"("Value"=w2848) -> ()  [unwired: 2 in, 2 out]
        n1066 = property on="VISA Marvin" class="VISAName"(error in=w2863, "Visible"=w2851, "Value"=w2861) -> (error out=w2852:errorcluster)  [unwired: 1 in, 1 out]
        n1067 = property on="Stop Burn-in" class="Bool (strict)"(error in=w2852, "Visible"=w2851) -> (error out=w2845:errorcluster)  [unwired: 1 in, 1 out]
        n1068 = property on="BurnDC" class="Bool (strict)"("Value"=w2847) -> ()  [unwired: 2 in, 2 out]
        n1069 = property on="BurnTemp" class="Bool (strict)"("Value"=w2847) -> ()  [unwired: 2 in, 2 out]
        n1070 = property on="BurnSpeed" class="Bool (strict)"("Value"=w2847) -> ()  [unwired: 2 in, 2 out]
        n1071 = property on="BurnResult" class="Bool (strict)"("Value"=w2847) -> ()  [unwired: 2 in, 2 out]
        n1072 = property on="Refresh Button" class="Bool (strict)"(error in=w2845, "Value"=FALSE ("Refresh Button")) -> ()  [unwired: 1 in, 2 out]
        n1073 = property on="StopTimeResult" class="Bool (strict)"("Value"=w2846) -> ()  [unwired: 2 in, 2 out]
        n1074 = property on="MotorTempResult" class="Bool (strict)"("Value"=w2846) -> ()  [unwired: 2 in, 2 out]
        n1075 = property on="TempControlResult" class="Bool (strict)"("Value"=w2846) -> ()  [unwired: 2 in, 2 out]
        n1076 = property on="Automation" class="Bool (strict)"("Value"=w2846) -> ()  [unwired: 2 in, 2 out]
        n1077 = flat-sequence {
          tunnel: w2845 -> [w2866]
          tunnel: [w2865] -> w2859
          tunnel: [w2869] -> w2858
          tunnel: w2859 -> [w2869]
          tunnel: [w2881] -> w2857
          tunnel: w2858 -> [w2882]
          tunnel: [w2882] -> w2856
          frame #0 {
            n1078 = control-ref of="This VI"() -> (w2867:refnum<vi>)
            n1079 = invoke class="VI" method="Default Vals.Reinit All"(reference=w2867, error in=w2866) -> (error out=w2865:errorcluster)  [unwired: 1 in, 2 out]
          }
          frame #1 {
            w2872 = u32 4294967295  # AccMask
            w2868 = T4 0 items=["使用Flash参数", "使用界面设置参数"] ("InitFlag")
            w2870 = T6 0 items=["normal operation", "Listen-only mode", "test mode"]  # Mode
            w2871 = T5 3 items=["接收所有类型"=1, "只接收标准帧"=2, "只接收扩展帧"=3] ("Fliter")
            w2876 = u8 10 items=["5k bps"=1, "10k bps"=2, "20k bps"=3, "40k bps"=4, "50k bps"=5, "80k bps"=6, "100k bps"=7, "125k bps"=8, "200k bps"=9, "250k bps"=10, "400k bps"=11, "500k bps"=12, "666k bps"=13, "800k bps"=14, "1000k bps"=15, "33.33k bps"=16, "66.66k bps"=17, "83.33k bps"=18]  # kBaudRate
            w2873 = u32 0  # AccCode
            w2874 = T2 4 items=["USB-CAN"=3, "USB-CAN2"=4] ("DevType")
            w2875 = T7 {"DevType"=3, "DevIndex"=0, "CanIndex"=0, "VCI_INIT_CONFIG"={"AccCode"=0, "AccMask"=0, "InitFlag"=1, "Fliter"=7, "Timing0"=0, "Timing1"=0, "Mode"=0}}  # Config
            # "CANalystII"
            n1080 = call "Demo_GetT0T1.vi"("kBaudRate"=w2876) -> ("Timing0"=w2878:u8, "Timing1"=w2879:u8)
            n1081 = Bundle By Name(cluster=w2875, "DevType"=w2874, "CanIndex"="Channel 2", "VCI_INIT_CONFIG.AccCode"=w2873, "VCI_INIT_CONFIG.AccMask"=w2872, "VCI_INIT_CONFIG.InitFlag"=w2868, "VCI_INIT_CONFIG.Fliter"=w2871, "VCI_INIT_CONFIG.Timing0"=w2878, "VCI_INIT_CONFIG.Timing1"=w2879, "VCI_INIT_CONFIG.Mode"=w2870) -> (→"Config_CANAT":T7)
          }
          frame #2 {
            w2883 = u16 284 items=["1M"=20, "500K"=28, "250K"=284, "125K"=796, "100K"=17199, "50K"=18223, "20K"=21295, "10K"=26415, "5K"=32639] ("baud in")
            n1082 = control-ref of="Config_CANAT"() -> (w2881:refnum<vi>)
            n1083 = call "InitCAN_ATII.vi"("Config"=w2881) -> ("Sts"=→"CAN Status":bool)
            n1084 = call "ChangeCANBaud.vi"("baud in"=w2883, "reference"=w2881) -> ()
          }
        }
        "Status" <- w2844
        "Test Failed" <- w2844
      }
    }
  }
  n1085 = property on="Settings" class="Bool (strict)"("Visible"=w7) -> ()  [unwired: 2 in, 2 out]
  n1086 = property on="Cal" class="DigNum (strict)"("Visible"=w7) -> ()  [unwired: 2 in, 2 out]
  n1087 = disable-structure shown="Disabled" {
    frame Disabled {
      w2885 = T20."Disabled and Grayed Out" ("Disabled")
      w2886 = FALSE ("Start")
      n1088 = property on="VISA Tester" class="VISAName" props=["Value"]() -> ()  [unwired: 2 in, 3 out]
      n1089 = property on="Current SN" class="DigNum (strict)" props=["Value"]() -> ()  [unwired: 2 in, 3 out]
      n1090 = property on="UUT" class="DigNum (strict)" props=["Value"]() -> ()  [unwired: 2 in, 3 out]
      n1091 = property on="Status" class="Bool (strict)" props=["Value"]() -> ()  [unwired: 2 in, 3 out]
      n1092 = property on="UUT SoftwareVer" class="Str" props=["Value"]() -> ()  [unwired: 2 in, 3 out]
      n1093 = property on="Next SN" class="DigNum (strict)" props=["Value"]() -> ()  [unwired: 3 in, 2 out]
      n1094 = property on="Start" class="Bool (strict)"("Value"=w2886, "DisabledEnum"=w2885) -> ()  [unwired: 2 in, 2 out]
      n1095 = property on="Report" class="Bool (strict)"("Value"=w2886, "DisabledEnum"=w2885) -> ()  [unwired: 2 in, 2 out]
    }
    frame Enabled {
    }
  }
  n1096 = disable-structure shown="Disabled" {
    frame Disabled {
      (unwired) 0.02003173828125 ("x")
      n1097 = control-ref of="Stop Burn-in"() -> ()  [unwired: 1 out]
      n1098 = control-ref of="Stop Button"() -> ()  [unwired: 1 out]
      n1099 = control-ref of="Motor Speed RPM"() -> ()  [unwired: 1 out]
      n1100 = control-ref of="Config_CANAT"() -> ()  [unwired: 1 out]
      n1101 = control-ref of="UUT"() -> ()  [unwired: 1 out]
      n1102 = call "GetADCTester (SubVI).vi"() -> ()  [unwired: 9 in, 3 out]
      n1103 = call "CANSendMotorSpeed.vi"() -> ()  [unwired: 11 in, 1 out]
      n1104 = control-ref of="Config_CANAT"() -> ()  [unwired: 1 out]
      n1105 = call "Find_Number_LineMARVIN.vi"() -> ()  [unwired: 5 in, 4 out]
      n1106 = property on="UUT" class="DigNum (strict)" props=["Value"]() -> ()  [unwired: 2 in, 3 out]
      n1107 = control-ref of="UUT"() -> ()  [unwired: 1 out]
      n1108 = call "DegToDAC (SubVI).vi"() -> ()  [unwired: 10 in, 2 out]
      n1109 = call "Write panel message (SubVI).vi"() -> ()  [unwired: 11 in, 1 out]
      n1110 = property on="VISA Tester" class="VISAName" props=["Value"]() -> ()  [unwired: 2 in, 3 out]
      n1111 = control-ref of="ATR"() -> ()  [unwired: 1 out]
      n1112 = call "TesterOption (SubVI).vi"() -> ()  [unwired: 10 in, 2 out]
      n1113 = call "TesterOption (SubVI).vi"() -> ()  [unwired: 10 in, 2 out]
      n1114 = call "PassOrFail (SubVI).vi"() -> ()  [unwired: 11 in, 1 out]
    }
    frame Enabled {
    }
  }
  n1115 = disable-structure shown="Disabled" {
    frame Disabled {
      n1116 = flat-sequence {
        frame #0 {
          n1117 = call "CANSendMotorSpeed.vi"("Remote"=TRUE, "Motor Speed RPM"=u16 0) -> ("error out"=w2888:errorcluster, "UUT"=w2891:refnum<vi>)  [unwired: 8 in]
          n1118 = property on="VISA Tester" class="VISAName"() -> ("Value"=w2887:refnum<visa-resource-name>)  [unwired: 2 in, 2 out]
          n1119 = call "TesterOption (SubVI).vi"("error in (no error)"=w2888, "On/Off"=FALSE, "Tester Option"=T11."Power", "VISA Refnum in"=w2887) -> ()  [unwired: 6 in, 2 out]
        }
      }
    }
    frame Enabled {
    }
  }
  "Pannel User Message" <- w5
